vi "ControlProgram6.6_8_updateFFB.vi"() -> ()   [LabVIEW 2016]
uses:
  <vilib>/Utility/miscctls.llb/LVPoint32TypeDef.ctl
  <vilib>/Platform/TimedLoop/XDataNode/timing_clust.ctl
  <vilib>/Platform/TimedLoop/XDataNode/nitl_modes.ctl
  <vilib>/Platform/TimedLoop/XDataNode/wakeup.ctl
  <vilib>/Instr/_visa.llb/Select Event Type.ctl
  <vilib>/vision/Avi1.llb/AviRefnum.ctl
  <vilib>/Utility/error.llb/DialogType.ctl
  <vilib>/DAQmx/write.llb/DAQmx Write (Analog 1D DBL NChan 1Samp).vi
  <vilib>/DAQmx/read.llb/DAQmx Read (Analog 2D DBL NChan NSamp).vi
  <vilib>/Analysis/baseanly.llb/Mean (DBL).vi
  <vilib>/DAQmx/write.llb/DAQmx Write (Digital Bool 1Line 1Point).vi
  <vilib>/DAQmx/create/channels.llb/DAQmx Create Channel (DO-Digital Output).vi
  <vilib>/DAQmx/create/channels.llb/DAQmx Create Channel (AI-Voltage-Basic).vi
  <vilib>/DAQmx/create/channels.llb/DAQmx Create Channel (AO-Voltage-Basic).vi
  <vilib>/DAQmx/configure/timing.llb/DAQmx Timing (Sample Clock).vi
  <vilib>/DAQmx/miscellaneous.llb/DAQmx Fill In Error Info.vi
  <vilib>/Instr/_visa.llb/VISA Configure Serial Port (Instr).vi
  Arnulf--joystick/git(most_up_to_date)/Logitech-joystick/Old Trap/FAST_Global_var.vi
  <vilib>/Utility/inputDevices.llb/mouseAcquire.vi
  <vilib>/Utility/inputDevices.llb/closeMouse.vi
  <vilib>/platform/TimedLoop/XDataNode/XDataNode.xnode
  <vilib>/Platform/TimedLoop/XDataNode/XDNodeRunTimeDep.lvlib
  <resource>/objmgr/daqmx.rc
  <vilib>/Analysis/NI_AALBase.lvlib
panel:
  out "offset ffb param":T1
  in  "Save file index":i32
  out "Saving Move":bool
  out "Move time":string
  out "Primary Video Display":T2(plugin-control)
  out "Flush Sample Start Time":u32=2111292881
  out "Sample flush time (s)":dbl=48.0
  in  "Inject Sample":bool
  out "Cal values":T3={"AX alpha"=612.9626061060078, "BX alpha"=549.6584469744151, "AX kappa"=0.3485731373010688, "BX kappa"=0.3853424216291352, "AX offset"=-0.03900484438240665, "BX offset"=-0.11295550662085417, "AY alpha"=582.7562541114835, "BY alpha"=571.1587543790358, "AY kappa"=0.37498408087930674, "BY kappa"=0.36252029651198364, "AY offset"=-0.21125584642206058, "BY offset"=-0.12469077200400738}
  in  "Inject Pump 1":bool
  in  "Inject Pump 2":bool
  in  "Tab Control 2":T4(tab)
  in  "Force FB script":bool
  in  "Got ADig bead":bool
  in  "Move Cap. 2 (ADig Top)":bool
  in  "Dump beads":bool
  in  "Got DNA bead":bool
  in  "Flow on\ncap 2?":bool=TRUE
  in  "Flow on\ncap 1?":bool=TRUE
  in  "Flow on\ndump?":bool=TRUE
  in  "Raster set":i32=1
  in  "Fish After TA?":bool=TRUE
  in  "Delta after tether":dbl=1700.0
  in  "TA Cancel Save?":bool=TRUE
  in  "Min fish\ndelta (nm)":dbl=1425.0 min=0.0 max=5000.0 step=50.0
  in  "Max fish\ndelta (nm)":dbl=1900.0 min=0.0 max=5000.0 step=25.0
  in  "Fish Speed (ms)":i32=5000
  in  "Wait (ms)":i32=1500
  in  "# attempts":dbl=10.0
  in  "Cutoff force (pN)":dbl=4.5
  in  "Raster after\n tether?":bool=TRUE
  out "Tether":bool
  out "Attempt #":i32
  in  "Flow on\nwhile fish?":bool=TRUE
  in  "Flow on\nafter raster?":bool=TRUE
  in  "Offset raster set":i32
  in  "Offset @ Delta (nm)":dbl=1700.0
  in  "Cal @ Delta (nm)":dbl=2500.0
  in  "Cal stage position":i32=3
  out "Cal Final Sampling Rate":dbl=125000.0
  in  "Cal Averaging":i32=1
  in  "Wait before dip (s)":dbl=3.0
  in  "Start dipping after?":bool
  in  "Start trap delta (nm)":dbl=1700.0
  in  "Repeat Dip":bool
  out "Dip #":i32
  in  "Dip attempts":dbl=3.0
  in  "Cancel Rep\n Dip":bool
  out "Return elasped time":i32
  in  "Return duration":dbl=15.0
  in  "Cancel dwell":bool=TRUE
  in  "Pause dwell":bool
  in  "Start/Return position":dbl=3.0
  in  "Dip duration":dbl=15.0
  in  "Dip position":dbl=4.0
  in  "Dip":bool
  out "Dip elasped time":i32
  in  "Stop":bool=TRUE
  in  "?":T5(tab)
  out "FAST X-Y":bool
  out "FAST Z":bool
  in  "Cal time (s)":dbl=5.0
  in  "Save N sets":bool
  in  "N sets":i32=200
  out "Cal sets to save":i32=500
  in  "Reset data stream":bool
  out "Buffer Overflow":bool
  out "Stage moving":bool
  in  "Comment":string
  in  "Raster scan":bool
  out "Saving":bool
  in  "Save cal":bool
  in  "Save Data":bool
  in  "Stop saving":bool
  out "Calibrating":bool
  out "Progress":dbl(slide) scale=0.0..100.0
  in  "Read Cal":bool
  in  "Fish":bool
  in  "Averaging Number":i32=1250
  out "Final Sampling Rate":dbl=100.0
  in  "Trap position (V)":cluster{"X":dbl, "Y":dbl}={"X"=3.9042624789680316, "Y"=0.2}
  in  "Trap delta (nm)":dbl=2500.0 min=0.0 max=5000.0 step=50.0
  in  "Fixed X":dbl=1.1
  in  "Fixed Y":dbl=0.15
  in  "Shutter 1 (B)":bool
  in  "Shutter 2 (A)":bool
  in  "Pulling direction":bool
  out "Raster scanning...":bool
  out "Current file name":path=path "D:/data/160111/160111_006.dat"
  in  "AX alpha":dbl=612.9626061060078 format="%#_3p"
  in  "BX alpha":dbl=549.6584469744151 format="%#_3g"
  in  "AX kappa":dbl=0.3485731373010688 format="%#_3g"
  in  "BX kappa":dbl=0.3853424216291352 format="%#_3g"
  in  "AX offset":dbl=-0.03900484438240665 format="%#_3g"
  in  "BX offset":dbl=-0.11295550662085417 format="%#_3g"
  in  "AY alpha":dbl=582.7562541114835 format="%#_3g"
  in  "BY alpha":dbl=571.1587543790358 format="%#_3g"
  in  "AY kappa":dbl=0.37498408087930674 format="%#_3g"
  in  "BY kappa":dbl=0.36252029651198364 format="%#_3g"
  in  "AY offset":dbl=-0.21125584642206058 format="%#_3g"
  in  "BY offset":dbl=-0.12469077200400738 format="%#_3g"
  out "Buffer status":u8(slide) scale=0.0..100.0
  in  "Target":bool
  in  "Set Current\nPos to (0,0,0)":bool
  in  "dump spot":string="Dump beads spot"
  in  "up flow spot":string="Upper flow spot"
  in  "low flow spot":string="Lower flow spot"
  in  "up cap":string="Upper capillary (ADig beads)"
  in  "bottom cap":string="Lower capillary (DNA beads)"
  in  "Move to Position 5":bool
  in  "Set Position 5":bool
  in  "Saved stage positions":dbl[][](array[numeric])=[[1.0, 0.0, 0.0, 0.0], [2.0, -0.13716, -3.21132, 0.01436], [3.0, 0.45, -0.73974, 0.005], [4.0, 0.45, -2.1978, 0.005], [5.0, 0.45, -2.63158, -0.02256]]
  in  "Set Position 2":bool
  in  "Move to Position 2":bool
  in  "Set Position 1":bool
  in  "Move to Position 1":bool
  in  "Set Position 4":bool
  in  "Move to Position 4":bool
  in  "Set Position 3":bool
  in  "Move to Position 3":bool
  out "Stage error":errorcluster
  in  "Clear Volume":bool
  out "Sample Flush Meter":u8(slide) scale=0.0..100.0
  out "Flushing Sample":bool
  in  "Flush Sample":bool
  in  "Normal \nRate (ul/hr)  3":dbl=100.0
  in  "Normal \nVolume (ul) 3":dbl=250.0
  in  "Normal \nVolume (ul) 2":dbl
  in  "Normal \nRate (ul/hr)":dbl
  in  "Normal \nVolume (ul)":dbl
  in  "Flush\nRate (ul/min)":dbl
  in  "Flush\nVolume (ul)":dbl
  in  "Flush \nRate (ul/min)  2":dbl
  in  "Flush Pump 2":bool
  in  "Flush\nVolume (ul)  2":dbl
  in  "Flush Pump 1":bool
  in  "Normal \nRate (ul/hr)  2":dbl
  in  "Write Wait":i32=1000
  in  "Flush \nRate (ul/min)  3":dbl=100.0
  in  "Flush\nVolume (ul)  3":dbl=80.0
  out "error out":errorcluster
  in  "Use Mouse to Move Trap?":bool
  in  "Pause Mouse/Mirror Connection":bool
  out "Reference Voltage":cluster{dbl, dbl}={0.0, -0.0}
  out "Saved voltage":cluster{dbl, dbl}={5.766666666666665, 1.45}
  out "Real Coordinates":cluster{"Horizontal":i32, "Vertical":i32}={"Horizontal"=897, "Vertical"=-1271}
  out "CoordinatesMousePressed":T6
  in  "reset offset ffb param":bool
  in  "Read \nOffset FFB param":bool
  in  "Force Feedback 2":bool
  in  "Offset 2":cluster{"Off Y":dbl, "Off X":dbl}={"Off Y"=1.5, "Off X"=0.17}
  in  "Setpoint voltage 2":cluster{"SP Y":dbl, "SP X":dbl}={"SP Y"=0.6, "SP X"=0.0}
  out "Sum error":dbl(knob) scale=-0.2..0.2
  out "Trap sep":waveform(dbl)[](graph)=[{"t0"=timestamp(4.489999999999949 s since 1904-01-01), "dt"=0.002, "Y"=[-1157.7639781743756, -1157.678951177374, -1157.7582331070425, -1157.7490409992681, -1157.8995617642552], "attributes"=variant("NI_ChannelName"=variant(string "T2 X"))}, {"t0"=timestamp(4.489999999999949 s since 1904-01-01), "dt"=0.002, "Y"=[-909.0775466981794, -909.1316439023619, -909.1322956759037, -909.1570630705896, -909.1264297140281], "attributes"=variant("NI_ChannelName"=variant(string "T2 Y"))}]
  in  "Set reading to\nsetpoint 1":bool
  in  "Offset Y (nm)":dbl format="%0.2f"
  in  "Offset X (nm)":dbl format="%0.2f"
  in  "Remove offsets":bool
  in  "Force Feedback 1":bool
  out "Feedback Output \nVoltage 2":cluster{dbl, dbl} {"?" format="%#_4g"; "?" format="%#_4g"}
  in  "Offset 1":cluster{"Off Y":dbl, "Off X":dbl}={"Off Y"=1.5, "Off X"=0.17}
  in  "Setpoint voltage 1":cluster{"SP Y":dbl, "SP X":dbl}={"SP Y"=0.6, "SP X"=0.0}
  in  "Feedback const":T7={"Ki_B_Y"=0.5, "Ki_B_X"=0.0, "Kp Y"=1.0, "Kp X"=0.0}
  out "Mean Trap Pos X 2 (nm)":dbl=-1157.769953044463 format="%0.2f"
  out "Mean Trp Pos Y 2 (nm)":dbl=-909.1249958122125 format="%0.2f"
  out "T2 X RMS (A)":dbl=0.7168002469275427 format="%0.2f"
  out "T2 Y RMS (A)":dbl=0.25997187037503383 format="%0.2f"
  in  "Set reading to\nsetpoint 2":bool
  in  "Scan range (nm)":dbl=425.0
  in  "Scan speed (nm/s)":dbl=100.0 min=0.0 max=100.0
  in  "Step size (nm)":dbl=1.0
  in  "Save scans":bool=TRUE
  in  "# scans":i32=1
  in  "Load param":bool
  in  "Scan Parameters":T8(array[cluster])
  in  "Trap delta\nafter (nm)":dbl=1550.0
  in  "Stop raster":bool
  out "Scan range (V)":dbl=0.47672462142456534
  out "Scan steps (mirror)":u64=425
  out "Scan increment (V)":dbl=0.0011217049915872126
  out "Time per step (ms)":dbl=10.0
  out "Total raster time (s)":dbl=8.5
  out "N sets to be saved":dbl=850.0
  out "moveX":string
  out "moveY":string
  in  "Grid Movable Trap":bool
  in  "take fixed bead\n Images":bool
  in  "Zoom Factor":sgl=7.0
  in  "Center Point":cluster{"X":i32, "Y":i32}={"X"=335, "Y"=271}
  in  "Intensity Upper":dbl=88.0
  in  "Intensity Lower":dbl=66.0
  out "Window Size":cluster{"Height":i32, "Width":i32}
  in  "Image Index":dbl=1.0 min=1.0
  in  "Save Image":bool
  in  "Averaging":bool
  in  "Reset Averaging":bool
  in  "Save Video":bool
  in  "New Video File":bool
  in  "Video Index":dbl=1.0 min=1.0 step=1.0
  in  "Video Capture Rate (Hz)":dbl=30.0
  in  "Initial Window Size":cluster{"Width":i32, "Height":i32}={"Width"=884, "Height"=619}
  in  "Initial Window Position":cluster{"X Position":i32, "Y Position":i32}={"X Position"=796, "Y Position"=4}
  out "Window Position":cluster{"X Position":i32, "Y Position":i32}={"X Position"=40, "Y Position"=40}
  out "Path Out":path
  in  "Target coordinates":cluster{"X1":dbl, "Y1":dbl, "X2":dbl, "Y2":dbl}={"X1"=328.0, "Y1"=274.0, "X2"=368.0, "Y2"=314.0}
  out "image8bitArray":u8[][](array[numeric])
  out "GreyscaleArray":u32[](array[numeric])
  in  "take background images":bool
  in  "# Samples/channel (in)":i32=40000 format="%.2f"
  out "Buffer size\n(Samples/channel)":u32=511
  out "DAQ rate\n(Samples/s)":dbl=125000.0 format="%#_6p"
  out "# Samples/channel":i32=1250
  out "# Samples/channel/s":dbl=100.0
  out "AvailSampPerChan":u32=9
  out "Data update period (s/set)":dbl=0.01 format="%#_6p"
  out "AvailSampPerChan 2":u32=110
  in  "PC samp per channel":i32=1000
  in  "Sampling Rate":dbl=125000.0 format="%0.0p"
  in  "DAQ Rate2":dbl=1000000.0 format="%#_6p"
  out "Data period (s)":dbl=8e-06 format="%#_6p"
  in  "Save user params":bool
  in  "User":string(combo)
  in  "Load user params":bool
  in  "Tether break\nforce (pN)":dbl=1.0
  in  "Path":path=path "E:/Data"
  out "Mirror task":refnum<k21>
  in  "Conv X (nm/V)":dbl=891.5
  in  "Conv Y (nm/V)":dbl=505.7
  in  "Min value Y":dbl format="%.1g"
  in  "Max value Y":dbl=10.0 format="%.1f"
  in  "Min value X":dbl format="%0.1f"
  in  "Max value X":dbl=10.0 format="%.1f"
  in  "HWP1":string="Half waveplate 1: differential trap power"
  in  "HWP0":string="Half waveplate 0: total trap power"
  in  "Move 1":bool
  in  "\"Degrees\" 1":dbl
  in  "Move 0":bool
  in  "\"Degrees\" 0":dbl
  in  "Y command":enum16{"Fish", "Dump", "Got ADig", "Got DNA"}(ring)
  in  "B command":enum16{"Got DNA", "Got ADig", "Dump", "Fish"}(ring)
  in  "A command":enum16{"Got ADig", "Dump", "Fish", "Got DNA"}(ring)
  in  "X command":enum16{"Dump", "Fish", "Got ADig", "Got DNA"}(ring)
  out "Logitech":bool
  out "START":bool
  out "BACK":bool
  out "Right stick button":bool
  out "Left Y":i8(slide) scale=-128.0..127.0
  out "Left X":i8(slide) scale=-128.0..127.0
  out "Right Y":i8(slide) scale=-128.0..127.0
  out "Right X":i8(slide) scale=-128.0..127.0
  out "X":bool
  out "Y":bool
  out "A":bool
  out "B":bool
  out "RB":bool
  out "LB":bool
  out "R":bool
  out "L":bool
  out "D":bool
  out "U":bool
  out "Left stick button":bool
  out "FAST Z":bool
  out "FAST X-Y":bool
  in  "XY Speed Definitions":T9={"Slow X velocity input"="0.05", "Slow Y velocity input"="0.05", "Fast1 X velocity input"="0.1", "Fast1 Y velocity input"="0.1", "Fast2 X velocity input"="0.2", "Fast2 Y velocity input"="0.2"}
  in  "Z Speed Definitions":cluster{"Slow Z":string, "Fast Z":string}={"Slow Z"="0.025", "Fast Z"="0.05"}
  in  "Z Wait time":string="120"
  in  "X-Y Wait time":string="125"
  in  "USB port":refnum<visa-resource-name>="USB0::0x046D::0xC21D::CC66247B::RAW"
  out "Deflection":T6
  in  "Sampling Rate":dbl=125000.0 format="%0.2f"
  in  "Averaging Number":i32=12500
  in  "DAQ Rate":dbl=1000000.0
  out "Final Sampling Rate":dbl
  in  "Tab Control":T10(tab)
  in  "Downsamp\nfact":dbl=250.0
  out "Bead sep":waveform(dbl)[](graph)=[{"t0"=timestamp(4.489999999999949 s since 1904-01-01), "dt"=0.002, "Y"=[8093.963535945606, 8103.1617772716045, 8385.72390184118, 8245.733099167523, 8154.925676756515], "attributes"=variant("NI_ChannelName"=variant(string "T2"))}, {"t0"=timestamp(4.489999999999949 s since 1904-01-01), "dt"=0.002, "Y"=[1717.924930434114, 1628.723007842151, 1787.6888378897193, 1598.475730715916, 1776.2517588078954], "attributes"=variant("NI_ChannelName"=variant(string "T1"))}]
  out "Force (pN)":waveform(dbl)[](graph)=[{"t0"=timestamp(4.489999999999949 s since 1904-01-01), "dt"=0.002, "Y"=[2821.5994183803123, 2824.8226375853515, 2923.3663028678166, 2874.5254578927593, 2842.869034836209], "attributes"=variant("NI_ChannelName"=variant(string "T2"))}, {"t0"=timestamp(4.489999999999949 s since 1904-01-01), "dt"=0.002, "Y"=[623.5850847499229, 591.0680427774053, 648.761979867749, 579.944408346982, 644.7436619059413], "attributes"=variant("NI_ChannelName"=variant(string "T1"))}]
  out "Mean force (pN)":dbl=1737.5286029210451 format="%0.2f"
  out "Force noise (pN)":dbl=26.83032703631318 format="%0.2f"
  out "Mean Bead Sep\n(nm)":dbl=4949.257225667222 format="%0.2f"
  out "Bead Sep Noise\n(A)":dbl=757.8078481959694 format="%0.2f"
  out "PSD 2":cluster{dbl[], dbl[]}(graph)
  out "PSD 1":cluster{dbl[], dbl[]}(graph)
  out "PSD 1 Sum":dbl(slide) scale=0.0..10.0
  out "PSD 2 Sum":dbl(slide) scale=0.0..10.0
  in  "Start":bool
  out "All signals 2":waveform(dbl)[](graph)=[{"t0"=timestamp(4.489999999999949 s since 1904-01-01), "dt"=0.002, "Y"=[0.0010396217068286443, 0.0010666908927528754, 0.001103298744846499, 0.0010651440823993424, 0.0010656596859401936], "attributes"=variant("NI_ChannelName"=variant(string "A y"))}, {"t0"=timestamp(4.489999999999949 s since 1904-01-01), "dt"=0.002, "Y"=[0.02000680227246931, 0.020097032918054827, 0.02003412926844257, 0.020136734401221615, 0.020087494249822452], "attributes"=variant("NI_ChannelName"=variant(string "A x"))}, {"t0"=timestamp(4.489999999999949 s since 1904-01-01), "dt"=0.002, "Y"=[-0.0014958587831537804, -0.0015046240440107857, -0.0014930229638311983, -0.001533240041751485, -0.0015262793936602433], "attributes"=variant("NI_ChannelName"=variant(string "B y"))}, {"t0"=timestamp(4.489999999999949 s since 1904-01-01), "dt"=0.002, "Y"=[0.0002901198559372817, 0.0002731049385577592, 0.00026511308349727467, 0.0002517073909711183, 0.0002916666665966012], "attributes"=variant("NI_ChannelName"=variant(string "B x"))}, {"t0"=timestamp(4.489999999999949 s since 1904-01-01), "dt"=0.002, "Y"=[-0.001511556786147372, -0.0015167122027053212, -0.0014612914746018214, -0.0014935128282145193, -0.0015064013696263116], "attributes"=variant("NI_ChannelName"=variant(string "A sum"))}, {"t0"=timestamp(4.489999999999949 s since 1904-01-01), "dt"=0.002, "Y"=[-0.0005242945138364382, -0.0005565158674093218, -0.000501095139248956, -0.0005771375336978897, -0.0005165613890095197], "attributes"=variant("NI_ChannelName"=variant(string "B sum"))}, {"t0"=timestamp(4.489999999999949 s since 1904-01-01), "dt"=0.002, "Y"=[0.0013303666019343777, 0.0014257418088905328, 0.0013368108726387405, 0.0013471217058124534, 0.0011782818123890176], "attributes"=variant("NI_ChannelName"=variant(string "Trap x"))}, {"t0"=timestamp(4.489999999999949 s since 1904-01-01), "dt"=0.002, "Y"=[0.0023382505474007294, 0.002231275652833831, 0.002229986798687363, 0.0021810103409340116, 0.002241586486003531], "attributes"=variant("NI_ChannelName"=variant(string "Trap y"))}]
  out "All signals":waveform(dbl)[](graph)=[{"t0"=timestamp(4.489999999999949 s since 1904-01-01), "dt"=0.002, "Y"=[0.0010396217068286443, 0.0010666908927528754, 0.001103298744846499, 0.0010651440823993424, 0.0010656596859401936], "attributes"=variant("NI_ChannelName"=variant(string "A y"))}, {"t0"=timestamp(4.489999999999949 s since 1904-01-01), "dt"=0.002, "Y"=[0.02000680227246931, 0.020097032918054827, 0.02003412926844257, 0.020136734401221615, 0.020087494249822452], "attributes"=variant("NI_ChannelName"=variant(string "A x"))}, {"t0"=timestamp(4.489999999999949 s since 1904-01-01), "dt"=0.002, "Y"=[-0.0014958587831537804, -0.0015046240440107857, -0.0014930229638311983, -0.001533240041751485, -0.0015262793936602433], "attributes"=variant("NI_ChannelName"=variant(string "B y"))}, {"t0"=timestamp(4.489999999999949 s since 1904-01-01), "dt"=0.002, "Y"=[0.0002901198559372817, 0.0002731049385577592, 0.00026511308349727467, 0.0002517073909711183, 0.0002916666665966012], "attributes"=variant("NI_ChannelName"=variant(string "B x"))}, {"t0"=timestamp(4.489999999999949 s since 1904-01-01), "dt"=0.002, "Y"=[-0.001511556786147372, -0.0015167122027053212, -0.0014612914746018214, -0.0014935128282145193, -0.0015064013696263116], "attributes"=variant("NI_ChannelName"=variant(string "A sum"))}, {"t0"=timestamp(4.489999999999949 s since 1904-01-01), "dt"=0.002, "Y"=[-0.0005242945138364382, -0.0005565158674093218, -0.000501095139248956, -0.0005771375336978897, -0.0005165613890095197], "attributes"=variant("NI_ChannelName"=variant(string "B sum"))}, {"t0"=timestamp(4.489999999999949 s since 1904-01-01), "dt"=0.002, "Y"=[0.0013303666019343777, 0.0014257418088905328, 0.0013368108726387405, 0.0013471217058124534, 0.0011782818123890176], "attributes"=variant("NI_ChannelName"=variant(string "Trap x"))}, {"t0"=timestamp(4.489999999999949 s since 1904-01-01), "dt"=0.002, "Y"=[0.0023382505474007294, 0.002231275652833831, 0.002229986798687363, 0.0021810103409340116, 0.002241586486003531], "attributes"=variant("NI_ChannelName"=variant(string "Trap y"))}]
  out "Chart Freq (Hz)":dbl=500.0
  # "Bead Calibration"
  # "Y"
  # "X"
  # "Pump #1 Controls"
  # "Pump #2 Controls"
  # "Sample Pump Controls"
  # "Retract the pumps manually. Change it back to INFUSE when you're done. Suck it up, don't whine."
  # "Shutter 1 (B)"
  # "Move to Lower Cap"
  # "Inject Sample"
  # "Move to Upper Cap"
  # "Shutter 2 (A)"
  # "Select the Joystick input:"
  # "Overflow happens when >40 commands\nsent in 5 seconds. Then 4 consecutive beeps."
  # "Try increasing wait time to reduce 'following error threshold exceeded' occurances."
  # "Left stick controls Z axis.\nRight on stick: neg Z-dir\nUp on stick: neg Z-dir"
  # "Toggles FAST Z"
  # "Toggles FAST X-Y"
  # "The default Newport max velocity is 0.4"
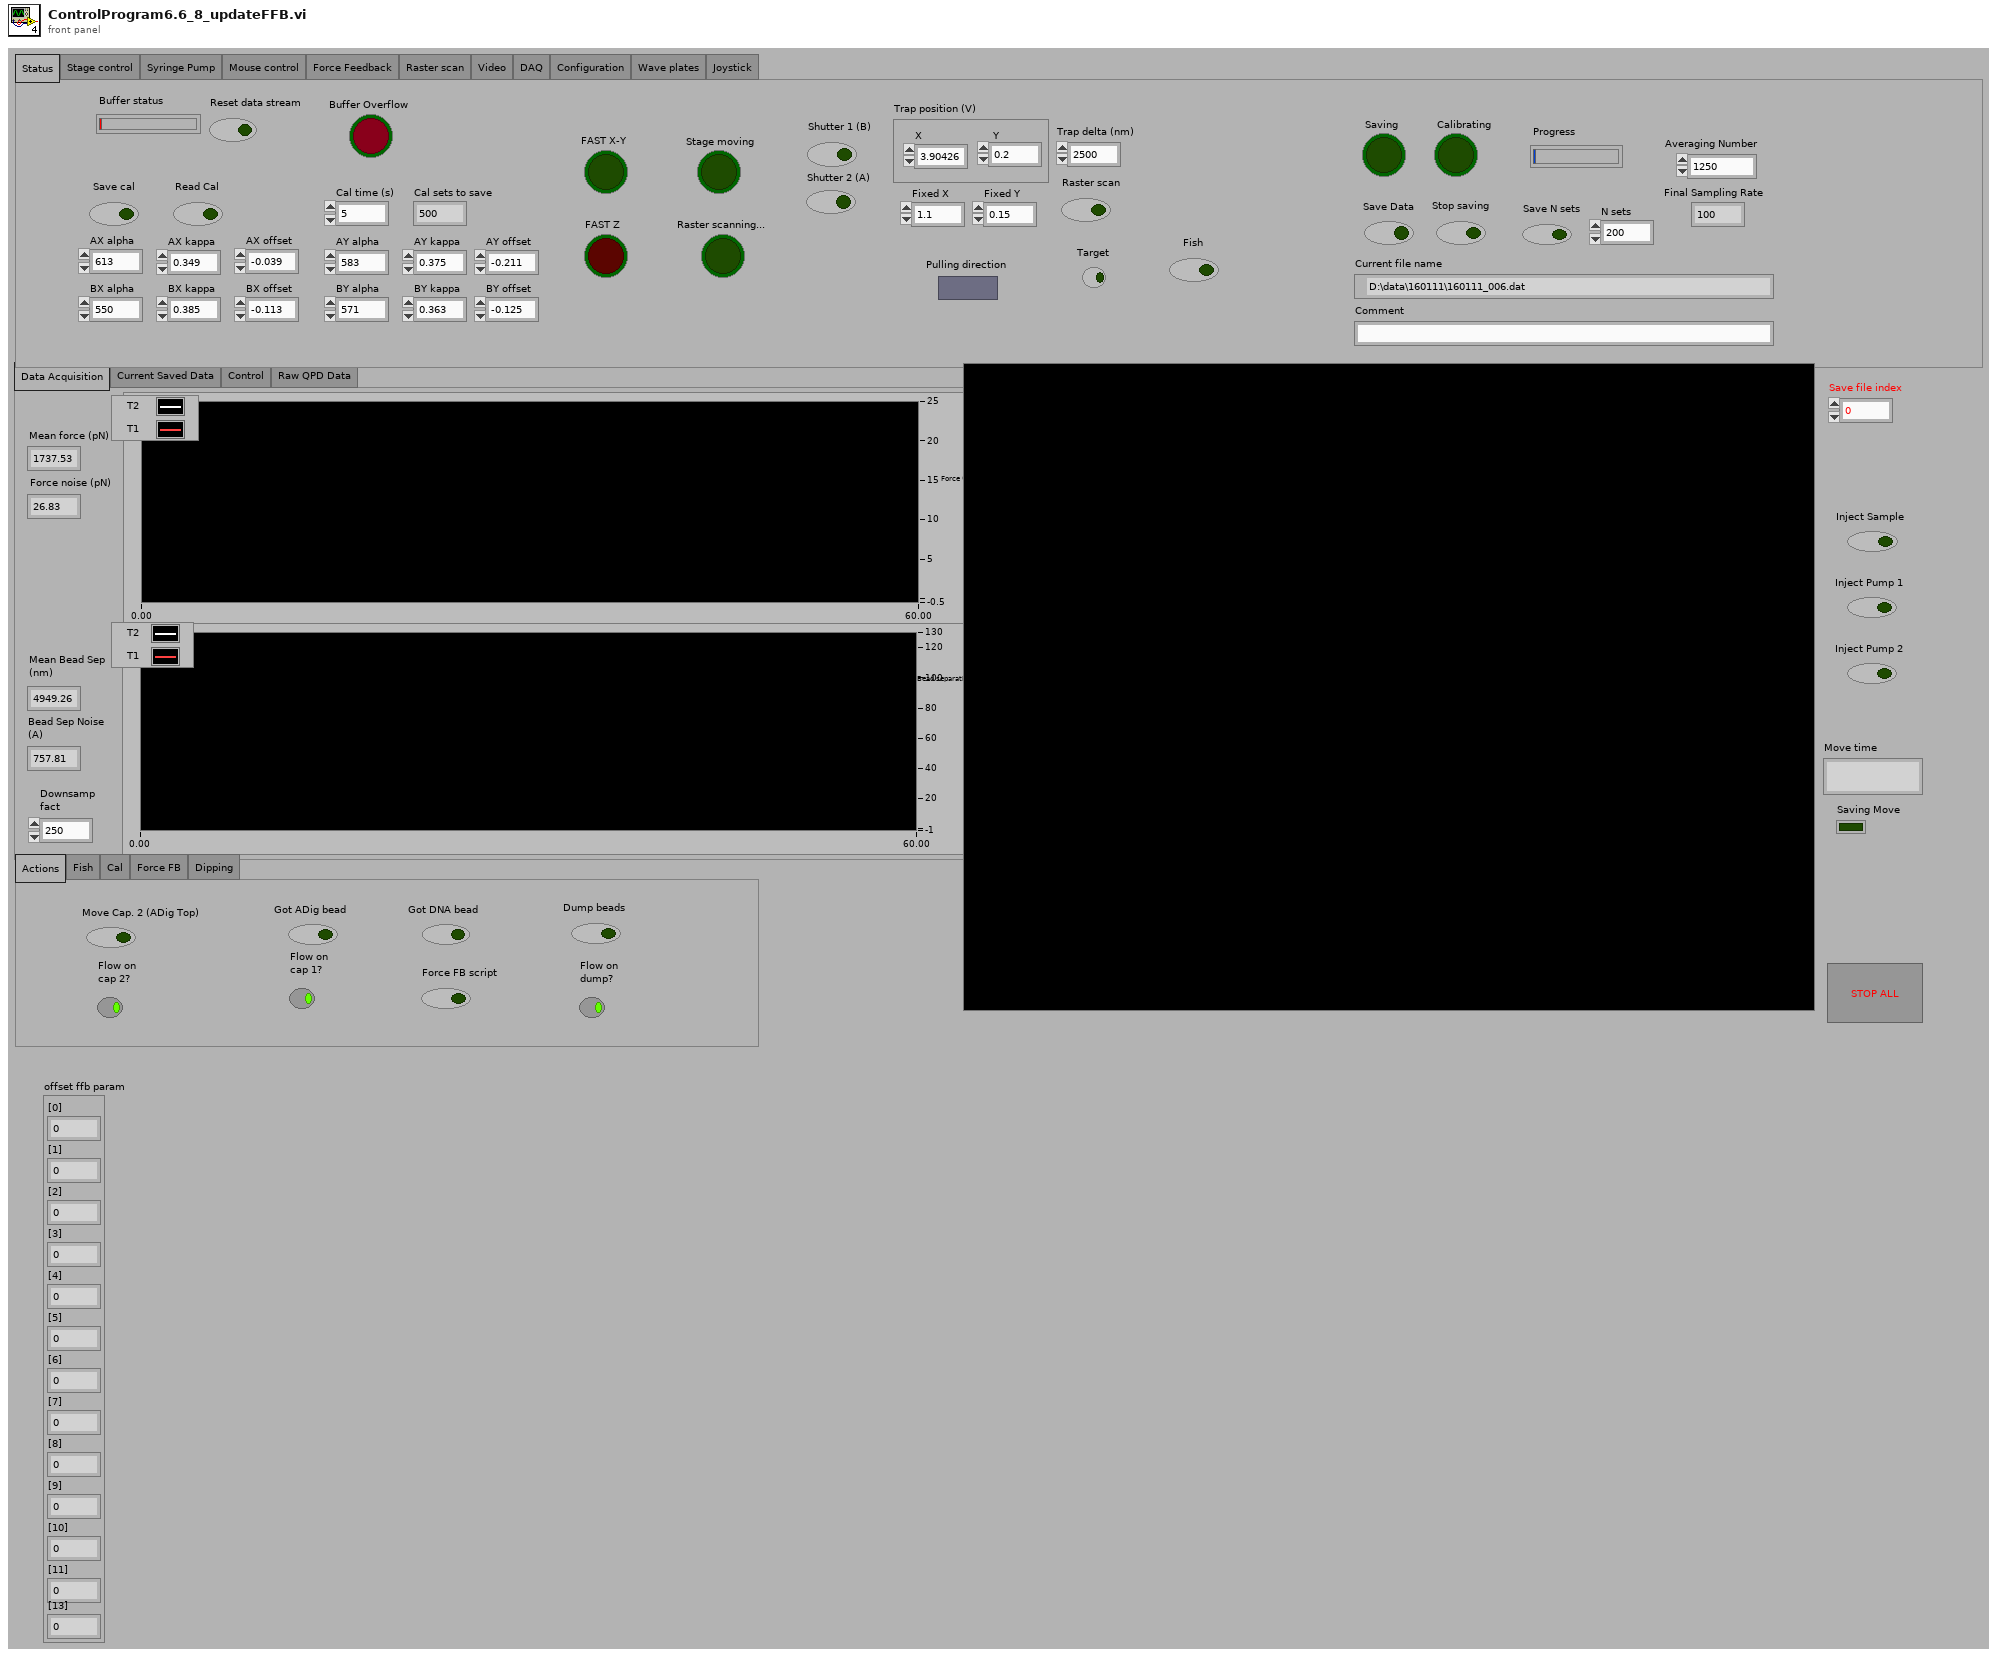
[diagram p1: front panel]
types:
  T1 = cluster{"[0]":dbl, "[1]":dbl, "[2]":dbl, "[3]":dbl, "[4]":dbl, "[5]":dbl, "[6]":dbl, "[7]":dbl, "[8]":dbl, "[9]":dbl, "[10]":dbl, "[11]":dbl, "[13]":dbl}
  T2 = typedef "IMAQ Image.ctl" = refnum<image>
  T3 = cluster{"AX alpha":dbl, "BX alpha":dbl, "AX kappa":dbl, "BX kappa":dbl, "AX offset":dbl, "BX offset":dbl, "AY alpha":dbl, "BY alpha":dbl, "AY kappa":dbl, "BY kappa":dbl, "AY offset":dbl, "BY offset":dbl}
  T4 = enum32{"Actions", "Fish", "Cal", "Force FB", "Dipping"}
  T5 = enum32{"Status", "Stage control", "Syringe Pump", "Mouse control", "Force Feedback", "Raster scan", "Video", "DAQ", "Configuration", "Wave plates", "Joystick"}
  T6 = typedef "LVPoint32TypeDef.ctl" = cluster{"Horizontal":i32, "Vertical":i32}
  T7 = cluster{"Ki_B_Y":dbl, "Ki_B_X":dbl, "Kp Y":dbl, "Kp X":dbl}
  T8 = cluster{"Label":string, "Scan range 1":dbl, "Step size 1":dbl, "Scan speed 1":i32, "# scans 2":i32}[]
  T9 = cluster{"Slow X velocity input":string, "Slow Y velocity input":string, "Fast1 X velocity input":string, "Fast1 Y velocity input":string, "Fast2 X velocity input":string, "Fast2 Y velocity input":string}
  T10 = enum32{"Data Acquisition", "Current Saved Data", "Control", "Raw QPD Data"}
  T11 = typedef "Select Event Type.ctl" = u32
  T12 = enum32{"setting", "request", "request control", "info", "statistics", "system settings", "I/O sub system", "HRT control", "camera descriptions", "device specific data", "event sub system settings", "event sub system results", "image memory manager"}
  T13 = typedef "AviRefnum.ctl" = refnum<k1>
  T14 = typedef "XDNodeRunTimeDep.lvlib/timing_clust.ctl" = cluster{"Expected End [f-1]":u64, "Actual End [f-1]":u64, "Finished Late? [f-1]":bool, "Expected End [i-1]":u64, "Actual End [i-1]":u64, "Finished Late? [i-1]":bool, "Expected Start [i]":u64, "Actual Start [i]":u64, "Expected Start [f]":u64, "Actual Start [f]":u64, "Source Name":string, "Structure Name":string, "Period":i64, "Deadline":i64, "Offset":i64, "Start":i64, "Priority":i32, "Timeout":i32, "Mode":T15, "Wakeup Reason":T16, "Error":errorcluster, "Source Type":string, "Secondary Source Type":string, "Global End Time":u64, "Global Start Time":u64, "Frame Duration":u64, "Iteration Duration":u64, "Assigned CPU":i32, "I/O Scan Engine Mode":u32}
  T15 = typedef "XDNodeRunTimeDep.lvlib/nitl_modes.ctl" = enum32{"No Change", "Process missed periods, maintain original phase", "Discard missed periods, maintain original phase", "Process missed periods, ignore original phase", "Discard missed periods, ignore original phase"}
  T16 = typedef "XDNodeRunTimeDep.lvlib/wakeup.ctl" = enum32{"Normal", "Aborted", "Asynchronous wakeup", "Timing source error", "Timed loop error", "Timeout"}
  T17 = typedef "Image Type" = u32
  T18 = typedef "imagedata.ctl" = cluster{"image type":i32, "image depth":i32, "image":u8[], "mask":u8[], "colors":u32[], "Rectangle":cluster{"left":i16, "top":i16, "right":i16, "bottom":i16}}
  T19 = enum16{"open", "replace", "create", "open or create", "replace or create", "replace or create with confirmation"}
  T20 = enum16{"big-endian, network order", "native, host order", "little-endian"}
  T21 = cluster{string, string, string, string, string, string, string, string}
  T22 = cluster{"LB":bool, "RB":bool, "BACK":bool, "Logitech":bool, "START":bool}
  T23 = cluster{"Right X":i8, "Right Y":i8, "Left X":i8, "Left Y":i8}
  T24 = enum32{"Status", "Stage control", "Syringe Pump", "Mouse control", "Force Feedback", "Raster scan", "Video", "DAQ", "Configuration", "Wave plates"}
  T25 = typedef "DialogType.ctl" = u16
  T26 = cluster{"button 1":bool, "button 2":bool, "button 3":bool, "button 4":bool}
  T27 = cluster{"[0]":dbl, "[1]":dbl, "[2]":dbl, "[3]":dbl, "[4]":dbl, "[5]":dbl, "[6]":dbl, "[7]":dbl, "[8]":dbl, "[9]":dbl, "[10]":dbl, "[11]":dbl}
  T28 = cluster{"[0]":dbl, "[1]":dbl, "[2]":dbl, "[3]":dbl, "[4]":dbl, "[5]":dbl, "[6]":dbl, "[7]":dbl, "[8]":dbl, "[9]":dbl, "[10]":dbl, "[11]":dbl, "[12]":dbl}
  T29 = cluster{"array[0]":dbl, "array[1]":dbl, "array[2]":dbl, "array[3]":dbl, "array[4]":dbl, "array[5]":dbl, "array[6]":dbl, "array[7]":dbl, "array[8]":dbl, "array[9]":dbl, "array[10]":dbl, "array[11]":dbl, "array[12]":dbl}
  T30 = cluster{"Label":string, "Scan range 1":dbl, "Step size 1":dbl, "Scan speed 1":i32, "# scans 2":i32}
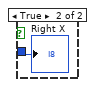
[diagram p5: hidden frame]
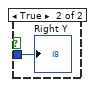
[diagram p6: hidden frame]
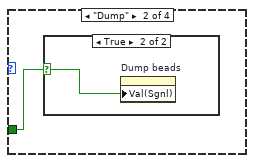
[diagram p10: hidden frame]
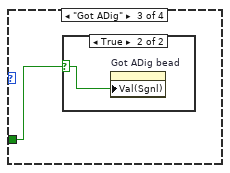
[diagram p12: hidden frame]
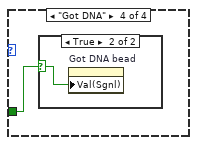
[diagram p14: hidden frame]
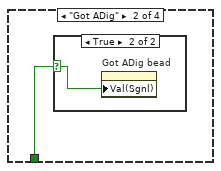
[diagram p17: hidden frame]
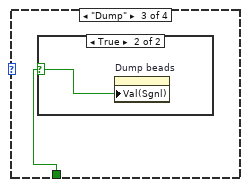
[diagram p19: hidden frame]
diagram:
  w10 = T11 1073684535 items=["Service Request"=1073684491, "Trigger"=3221168138, "Clear"=1073684493, "VXI Signal"=1073684512, "VXI/VME Interrupt"=3221168161, "VXI/VME Sysfail"=1073684509, "VXI/VME Sysreset"=1073684510, "GPIB CIC"=1073684498, "GPIB Talk"=1073684499, "GPIB Listen"=1073684500, "PXI Interrupt"=1073684514, "Serial Break"=1073684515, "Serial TermChar"=1073684516, "Serial CTS"=1073684521, "Serial DSR"=1073684522, "Serial DCD"=1073684524, "Serial RI"=1073684526, "Serial Character"=1073684533, "USB Interrupt"=1073684535, "All Enabled"=1073709055] ("Event Type")
  w49 = 10.0 ("Minimum Value")
  w50 = -10.0 ("Minimum Value")
  w52 = -2.0 ("Minimum Value")
  w53 = 2.0 ("Maximum Value")
  w78 = 10123 items=["Finite Samples"=10178, "Continuous Samples"=10123] ("sample mode")
  w98 = tag "Dev1/port2/line1"  # Shutter 2
  w101 = tag "Dev1/port1/line4"  # Shutter 1
  # "Open the RAW resource"
  # "Enable USB Interrupt Event"
  # "Create channels for movable mirror"
  # "Create channels for detectors"
  n1 = call-poly <vilib>:"DAQmx Create Virtual Channel.vi"("maximum value"=w53, "minimum value"=w52, "physical channels"=tag "Dev1/ai0" ("Physical Channel")) -> ("task out"=w54:refnum<k21>, "error out"=w77:errorcluster)  [unwired: 11 in]
  n2 = call-poly <vilib>:"DAQmx Create Virtual Channel.vi"("task in"=w54, "maximum value"=w53, "minimum value"=w52, "physical channels"=tag "Dev1/ai1", "error in"=w77) -> ("task out"=w75:refnum<k21>, "error out"=w74:errorcluster)  [unwired: 9 in]
  n3 = call-poly <vilib>:"DAQmx Create Virtual Channel.vi"("task in"=w75, "maximum value"=w53, "minimum value"=w52, "physical channels"=tag "Dev1/ai2", "error in"=w74) -> ("task out"=w66:refnum<k21>, "error out"=w65:errorcluster)  [unwired: 9 in]
  n4 = call-poly <vilib>:"DAQmx Create Virtual Channel.vi"("task in"=w66, "maximum value"=w53, "minimum value"=w52, "physical channels"=tag "Dev1/ai3" ("Physical Channel"), "error in"=w65) -> ("task out"=w51:refnum<k21>, "error out"=w71:errorcluster)  [unwired: 9 in]
  n5 = call-poly <vilib>:"DAQmx Create Virtual Channel.vi"("task in"=w51, "maximum value"=w49, "minimum value"=w50, "physical channels"=tag "Dev1/ai4", "error in"=w71) -> ("task out"=w69:refnum<k21>, "error out"=w68:errorcluster)  [unwired: 9 in]
  n6 = call-poly <vilib>:"DAQmx Create Virtual Channel.vi"("task in"=w69, "maximum value"=w49, "minimum value"=w50, "physical channels"=tag "Dev1/ai5", "error in"=w68) -> ("task out"=w64:refnum<k21>, "error out"=w63:errorcluster)  [unwired: 9 in]
  n7 = call-poly <vilib>:"DAQmx Create Virtual Channel.vi"("task in"=w64, "maximum value"=w49, "minimum value"=w50, "physical channels"=tag "Dev1/ai6", "error in"=w63) -> ("task out"=w58:refnum<k21>, "error out"=w56:errorcluster)  [unwired: 9 in]
  n8 = call-poly <vilib>:"DAQmx Create Virtual Channel.vi"("task in"=w58, "maximum value"=w49, "minimum value"=w50, "physical channels"=tag "Dev1/ai7", "error in"=w56) -> ("task out"=w57:refnum<k21>, "error out"=w55:errorcluster)  [unwired: 9 in]
  n9 = call-poly <vilib>:"DAQmx Timing.vi"("task/channels in"=w57, "sample mode"=w78, "samples per channel"="PC samp per channel", "rate"="Sampling Rate", "error in"=w55) -> ("task out"=w61:refnum<k21>, "error out"=w60:errorcluster)  [unwired: 9 in]
  n10 = call-poly <vilib>:"DAQmx Create Virtual Channel.vi"("maximum value"="Max value Y", "minimum value"="Min value Y", "physical channels"=tag "Dev1/ao1" ("Trap X Axis")) -> ("task out"=w46:refnum<k21>, "error out"=w48:errorcluster)  [unwired: 11 in]
  n11 = property class="DAQmx Timing"(reference=w61, error in=w60, "More:AI Convert:Rate"="DAQ Rate2") -> (reference out=w19:refnum<k21>, error out=w18:errorcluster, "SampClk.Rate"=→"DAQ rate\n(Samples/s)":dbl)
  n12 = call-poly <vilib>:"DAQmx Create Virtual Channel.vi"("task in"=w46, "maximum value"="Max value X", "minimum value"="Min value X", "physical channels"=tag "Dev1/ao0" ("Trap Y Axis"), "error in"=w48) -> ("task out"=w37:refnum<k21>, "error out"=w36:errorcluster)  [unwired: 9 in]
  "Mirror task" <- w37
  n13 = property class="DAQmx Buffer"(reference=w19, error in=w18) -> (reference out=w16:refnum<k21>, error out=w15:errorcluster, "Input.OnbrdBufSize"=→"Buffer size\n(Samples/channel)":u32)
  n14 = call <vilib>:"DAQmx Start Task.vi"("task/channels in"=w16, "error in"=w15) -> ("task out"=w38:refnum<k21>)  [unwired: 12 in, 1 out]
  n15 = flat-sequence "Video" {
    tunnel: [w114] -> w13
    tunnel: w13 -> [w155]
    frame #0 {
      n16 = while {
        stop <- w107 continue-if-true
        n17 = call "Close Video Capture.vi"() -> ("error code OUT"=w109:i32)
        n18 = Equal?(x=w109, y=0) -> (x = y?=w107:bool)
      }
      n19 = local write "Stop"(FALSE ("Stop All")) -> ()
    }
    frame #1 {
      n20 = call "DMR_Init.vi"() -> ()  [unwired: 3 out]
    }
    frame #2 {
      # "Setting the destination format to Mono8 makes sure that the image can be displayed in the intensity plot."
      n21 = call "DMR_GetDevice.vi"("search string IN"="DE514724602") -> ("device handle OUT"=w132:i32)  [unwired: 4 in, 2 out]
      n22 = call "DMR_OpenDevice.vi"("device handle IN"=w132) -> ("driver handle OUT"=w115:i32)  [unwired: 4 out]
      n23 = call "DMR_FindList.vi"("flags IN"=u32 0 ("flags"), "list name IN"="" ("String"), "list type IN"=T12."camera descriptions", "driver handle IN"=w115) -> ("list handle OUT"=w118:i32)  [unwired: 2 out]
      n24 = call "DMR_FindList.vi"("flags IN"=u32 0 ("flags"), "list name IN"="Base", "list type IN"=T12."setting", "driver handle IN"=w115) -> ("list handle OUT"=w116:i32)  [unwired: 2 out]
      n25 = call "OBJ_GetHandle.vi"("object name IN"="VideoStandard", "list handle IN"=w118) -> ("object handle OUT"=w112:i32)  [unwired: 3 out]
      n26 = call "OBJ_GetHandle.vi"("object name IN"="PixelFormat", "list handle IN"=w116) -> ("object handle OUT"=w126:i32)  [unwired: 3 out]
      n27 = call "OBJ_SetS.vi"("value index IN"=0, "value IN"="NTSC M", "object handle IN"=w112) -> ()  [unwired: 2 out]
      n28 = call "OBJ_SetS.vi"("value index IN"=0, "value IN"="Mono8" ("value"), "object handle IN"=w126) -> ()  [unwired: 2 out]
      n29 = call "OBJ_GetHandle.vi"("object name IN"="VideoChannel", "list handle IN"=w116) -> ("object handle OUT"=w122:i32)  [unwired: 3 out]
      n30 = while {
        tunnel: [w137] -> w114
        tunnel: w115 -> [w134]
        stop <- w135 continue-if-true
        n31 = call "DMR_ImageRequestSingle.vi"("request control IN"=0, "driver handle IN"=w134) -> ("error code OUT"=w136:i32, "driver handle OUT"=w137:i32)  [unwired: 2 out]
        n32 = Equal To 0?(x=w136) -> (x = 0?=w135:bool)
      }
      n33 = call "OBJ_SetI.vi"("value index IN"=0, "value IN"=0 ("Video channel"), "object handle IN"=w122) -> ()  [unwired: 2 out]
    }
    frame #3 {
      w143 = T17 0 items=["Grayscale (U8)", "Grayscale (I16)", "Grayscale (SGL)", "Complex (CSG)", "RGB (U32)", "HSL (U32)", "RGB (U64)"] ("Image Type")
      w151 = T17 0 items=["Grayscale (U8)", "Grayscale (I16)", "Grayscale (SGL)", "Complex (CSG)", "RGB (U32)", "HSL (U32)", "RGB (U64)"] ("Image Type")
      n34 = for "Create Greyscale map" {
        N: 256 -> [_]
        tunnel: [w157] -> w140 mode=indexing
        workers-P: _ -> [_]
        i -> [w160]
        n35 = To Unsigned Byte Integer(number=w160) -> (unsigned 8bit integer=w156:u8)
        n36 = Join Numbers(hi=w156, lo=w156) -> ((hi.lo)=w159:u16)
        n37 = Join Numbers(hi=w156, lo=w156) -> ((hi.lo)=w158:u16)
        n38 = Join Numbers(hi=w159, lo=w158) -> ((hi.lo)=w157:u32)
      }
      n39 = call "IMAQ Create"("Image Name"="Scaled video", "Image Type"=w143) -> ("New Image"=w142:T2)  [unwired: 2 in, 2 out]
      n40 = call "IMAQ Create"("Image Name"="Main video", "Image Type"=w151) -> ("New Image"=w152:T2)  [unwired: 2 in, 2 out]
      n41 = node-c288(0 ("Processor")) -> (w150:T14)  [unwired: 3 out]
      n42 = Initialize Array(u32 0 ("Window Number (0...15)"), 480 ("dimension size"), 640 ("dimension size")) -> (w145:u32[][])
      n43 = timed-loop {
        tunnel: w155 -> [w177]
        tunnel: [w176] -> w154
        tunnel: w152 -> [w175]
        timing: w150 -> [_]
        timing-out: [_] -> w149
        tunnel: w145 -> [w164]
        tunnel: w142 -> [w162]
        tunnel: w140 -> [w161]
        stop <- w163 stop-if-true
        # "This block performs the \nactual image capture."
        n44 = node-c288() -> ()  [unwired: 2 out]
        n45 = local read "Stop"() -> (w163:bool)
        n46 = Reciprocal(x="Video Capture Rate (Hz)") -> (1/x=w167:dbl)
        n47 = Multiply(x=w167, y=1000.0) -> (x*y=w165:dbl)
        n48 = call "DMR_ImageRequestWaitFor.vi"("queue number IN"=0, "timeout(ms) IN"=500, "driver handle IN"=w177) -> ("error code OUT"=w181:i32, "request number OUT"=w178:i32, "driver handle OUT"=w179:i32)
        n49 = feedback #1(T13 refnum ("Avi Refnum")) -> (w169:T13)
        n50 = case shown="True" "New Video File" {
          tunnel: [T13 refnum ("Avi Refnum") w198] -> w171
          tunnel: [FALSE TRUE] -> w172
          tunnel: w169 -> [_ w194]
          frame False {
          }
          frame True {
            n51 = call "Create new save file.vi"("Ext"=".avi" ("string"), "Index In"="Video Index") -> ("Path Out"=w190:path, "Index Out"=w191:dbl)  [unwired: 1 in]
            "Path Out" <- w190
            n52 = Not Equal?(x=w194, y=T13 refnum ("Avi Refnum")) -> (x != y?=w195:bool)
            n53 = Increment(x=w191) -> (x+1=w200:dbl)
            n54 = case shown="True" w195 {
              tunnel: w194 -> [_ w201]
              frame False {
              }
              frame True {
                n55 = call "IMAQ AVI Close"("Avi Refnum"=w201) -> ()  [unwired: 1 in, 10 out]
              }
            }
            n56 = local write "Video Index"(w200) -> ()
            n57 = call "IMAQ AVI Create"("Frames Per Second"=u32 30, "AVI Path"=w190) -> ("Avi Refnum"=w198:T13)  [unwired: 5 in, 4 out]
          }
        }
        n58 = Equal To 0?(x=w181) -> (x = 0?=w180:bool)
        n59 = Select(t=w171, s=w172, f=w169) -> (s? t:f=w170:T13)
        n60 = feedback-in #1(w170) -> ()
        n61 = case shown="True" w180 {
          tunnel: w179 -> [w202 w231]
          tunnel: w178 -> [_ w230]
          tunnel: [w202 w227] -> w176
          tunnel: w175 -> [_ w210]
          tunnel: w164 -> [_ w215]
          tunnel: w170 -> [_ w213]
          tunnel: w162 -> [_ w211]
          tunnel: w161 -> [_ w204]
          frame False {
          }
          frame True {
            w221 = u32 0 ("X-offset IN")
            n62 = call "DMR_GetImageRequestBufferData.vi"("driver handle IN"=w231, "request number IN"=w230) -> ("width OUT"=w220:i32, "height OUT"=w219:i32, "driver handle OUT"=w226:i32, "request number OUT"=w225:i32, "bytes per pixel OUT"=w222:i32)  [unwired: 13 out]
            n63 = call "DMR_GetImageRequestBufferImageData.vi"("driver handle IN"=w226, "request number IN"=w225, "bytes per pixel IN"=w222, "X-offset IN"=w221, "Y-offset IN"=w221, "height IN"=w219, "width IN"=w220) -> ("driver handle OUT"=w224:u32, "request number OUT"=w223:u32, "image OUT"=w216:u32[][])  [unwired: 10 out]
            n64 = call "DMR_ImageRequestUnlock.vi"("request number IN"=w223, "driver handle IN"=w224) -> ("driver handle OUT"=w229:i32)  [unwired: 1 in, 2 out]
            n65 = case shown="False" "Averaging" {
              tunnel: w216 -> [w307 w312]
              tunnel: [w307 w311] -> w212
              tunnel: w215 -> [_ w309]
              frame False {
              }
              frame True {
                (unwired) 1
                w317 = 1
                n66 = feedback #2(w309) -> (w308:u32[][])
                n67 = Add(x=w312, y=w308) -> (x+y=w313:u32[][])
                n68 = Select(t=w309, s="Reset Averaging", f=w313) -> (s? t:f=w315:u32[][])
                n69 = feedback-in #2(w315) -> ()
                n70 = feedback #3(w317) -> (w310:i32)
                n71 = Divide(x=w313, y=w310) -> (x/y=w314:dbl[][])
                n72 = Increment(x=w310) -> (x+1=w318:i32)
                n73 = To Unsigned Long Integer(number=w314) -> (unsigned 32bit integer=w311:u32[][])
                n74 = Select(t=w317, s="Reset Averaging", f=w318) -> (s? t:f=w316:i32)
                n75 = feedback-in #3(w316) -> ()
              }
            }
            n76 = call "DMR_ImageRequestSingle.vi"("request control IN"=0, "driver handle IN"=w229) -> ("driver handle OUT"=w227:i32)  [unwired: 3 out]
            n77 = disable-structure shown="Disabled" {
              disable-tunnel: w212 -> [w284 _]
              disable-tunnel: w211 -> [w283 _]
              frame Disabled {
                n78 = To Double Precision Float(number=w284) -> (double precision float=w282:dbl[][])
                n79 = In Range and Coerce(upper limit="Intensity Upper", x=w282, lower limit="Intensity Lower") -> (coerced(x)=w281:dbl[][])  [unwired: 1 out]
                n80 = Subtract(x="Intensity Upper", y="Intensity Lower") -> (x-y=w278:dbl)
                n81 = Subtract(x=w281, y="Intensity Lower") -> (x-y=w279:dbl[][])
                n82 = Divide(x=w279, y=w278) -> (x/y=w280:dbl[][])
                n83 = Multiply(x=255.0, y=w280) -> (x*y=w276:dbl[][])
                n84 = To Unsigned Byte Integer(number=w276) -> (unsigned 8bit integer=w285:u8[][])
                n85 = call "IMAQ ArrayToImage"("Image Pixels (U8)"=w285, "Image"=w283) -> ("Image Out"=w272:T2)  [unwired: 4 in, 5 out]
                n86 = First Call?() -> (First Call?: T/F=w273:bool)
                n87 = case shown="True" w273 {
                  tunnel: w272 -> [w286 w297]
                  frame False {
                    n88 = flat-sequence {
                      tunnel: w286 -> [w292]
                      frame #0 {
                        w289 = FALSE ("Get/Set Status? (Set)")
                        w288 = 0 ("Window Number (0...15)")
                        n89 = call "IMAQ WindSize"("Get/Set Status? (Set)"=w289, "Window Number"=w288) -> ("Width & Height out"=→"Window Size":cluster{"Width":i32, "Height":i32})  [unwired: 4 in, 2 out]
                        n90 = call "IMAQ WindMove"("Window Number (0...15)"=w288, "Get/Set Status? (Set)"=w289) -> ("Coordinates (screen)"=→"Window Position":cluster{"X Position":i32, "Y Position":i32})  [unwired: 3 in, 1 out]
                        n91 = call "IMAQ WindDraw"("Resize to Image Size? (Y)"=FALSE, "Window Number (0...15)"=w288, "Image"=w292) -> ()  [unwired: 7 in, 2 out]
                      }
                      frame #1 {
                        n92 = call "IMAQ WindZoom 2"("Center Point"="Center Point", "Zoom to Fit? (False)"=FALSE, "Zoom Factor"="Zoom Factor") -> ()  [unwired: 5 in, 4 out]
                      }
                    }
                  }
                  frame True {
                    n93 = flat-sequence {
                      tunnel: w297 -> [w300]
                      tunnel: [w298] -> w296
                      tunnel: w296 -> [w302]
                      frame #0 {
                        w299 = TRUE ("Resize to Image Size? (Y)")
                        w298 = 0 ("Window Number (0...15)")
                        n94 = call "IMAQ WindNonTearing"("Window Number"=w298, "NonTearing? (True)"=w299) -> ()  [unwired: 8 in, 2 out]
                        n95 = call "IMAQ WindDraw"("Resize to Image Size? (Y)"=w299, "Window Number (0...15)"=w298, "Image"=w300) -> ()  [unwired: 7 in, 2 out]
                      }
                      frame #1 {
                        n96 = call "IMAQ WindSize"("Scrollbars? (N)"=FALSE, "Width & Height"="Initial Window Size", "Window Number"=w302) -> ()  [unwired: 3 in, 3 out]
                        n97 = call "IMAQ WindMove"("Window Number (0...15)"=w302, "Coordinates (screen)"="Initial Window Position") -> ()  [unwired: 3 in, 2 out]
                      }
                    }
                  }
                }
              }
              frame Enabled {
              }
            }
            n98 = To Unsigned Byte Integer(number=w212) -> (unsigned 8bit integer=w203:u8[][])
            "image8bitArray" <- w203
            n99 = call "IMAQ ArrayToImage"("Image Pixels (U8)"=w203, "Image"=w210) -> ("Image Out"=w208:T2)  [unwired: 4 in, 5 out]
            n100 = case shown="True" "take fixed bead\n Images" {
              tunnel: w203 -> [_ w251]
              tunnel: w204 -> [_ w250]
              frame False {
              }
              frame True {
                n101 = local write "take fixed bead\n Images"(FALSE ("Save 10 Images")) -> ()
                n102 = while {
                  tunnel: w251 -> [w253]
                  tunnel: w250 -> [w252]
                  i -> [w255]
                  stop <- w254 stop-if-true
                  n103 = flat-sequence {
                    tunnel: w253 -> [w265]
                    tunnel: w252 -> [w264]
                    frame #0 {
                      n104 = local read "Image Index"() -> (w261:dbl)
                      n105 = call "Create new save file.vi"("Insert"="fixed_" ("string"), "Ext"=".bmp" ("string"), "Index In"=w261) -> ("Path Out"=w262:path, "Index Out"=w258:dbl)
                      n106 = call <vilib>:"Flatten Pixmap.vi"("colors"=w264, "8-bit pixmap"=w265) -> ("image data"=w263:T18)  [unwired: 4 in, 5 out]
                      n107 = Increment(x=w258) -> (x+1=w257:dbl)
                      n108 = call <vilib>:"Write BMP File.vi"("image data"=w263, "path to BMP file"=w262) -> ()  [unwired: 1 in, 9 out]
                      n109 = local write "Image Index"(w257) -> ()
                    }
                    frame #1 {
                      n110 = Wait (ms)(milliseconds to wait=u32 50) -> ()  [unwired: 1 out]
                    }
                  }
                  n111 = Equal?(x=w255, y=9) -> (x = y?=w254:bool)
                }
              }
            }
            n112 = case shown="True" "Save Video" {
              tunnel: w213 -> [_ w306]
              tunnel: w208 -> [_ w305]
              frame False {
              }
              frame True {
                n113 = call "IMAQ AVI Write Frame"("Image"=w305, "Avi Refnum"=w306) -> ()  [unwired: 2 in, 8 out]
              }
            }
            n114 = case shown="True" "take background images" {
              tunnel: w204 -> [_ w233]
              tunnel: w203 -> [_ w232]
              frame False {
              }
              frame True {
                n115 = while {
                  tunnel: w233 -> [w235]
                  tunnel: w232 -> [w234]
                  i -> [w238]
                  stop <- w236 stop-if-true
                  n116 = flat-sequence {
                    tunnel: w235 -> [w240]
                    tunnel: w234 -> [w239]
                    frame #0 {
                      n117 = local read "Image Index"() -> (w246:dbl)
                      n118 = call "Create new save file.vi"("Insert"="background_" ("string"), "Ext"=".bmp" ("string"), "Index In"=w246) -> ("Path Out"=w242:path, "Index Out"=w243:dbl)
                      n119 = call <vilib>:"Flatten Pixmap.vi"("colors"=w240, "8-bit pixmap"=w239) -> ("image data"=w241:T18)  [unwired: 4 in, 5 out]
                      n120 = Increment(x=w243) -> (x+1=w247:dbl)
                      n121 = local write "Image Index"(w247) -> ()
                      n122 = call <vilib>:"Write BMP File.vi"("image data"=w241, "path to BMP file"=w242) -> ()  [unwired: 1 in, 9 out]
                    }
                    frame #1 {
                      n123 = Wait (ms)(milliseconds to wait=u32 50) -> ()  [unwired: 1 out]
                    }
                  }
                  n124 = Equal?(x=w238, y=9) -> (x = y?=w236:bool)
                }
              }
            }
            n125 = case shown="False" "Target" {
              tunnel: w208 -> [w267 w271]
              tunnel: [w267 w269] -> w207
              frame False {
              }
              frame True {
                n126 = local read "Target coordinates"() -> (w268:cluster{"X1":dbl, "Y1":dbl, "X2":dbl, "Y2":dbl})
                n127 = call "IMAQ Overlay Oval"("Color"=u32 16711680, "Bounding Rectangle"=w268, "Image"=w271) -> ("Image Out"=w269:T2)  [unwired: 7 in, 1 out]
              }
            }
            "Primary Video Display" <- w207
            n128 = case shown="True" "Save Image" {
              tunnel: w203 -> [_ w321]
              tunnel: w204 -> [_ w320]
              frame False {
              }
              frame True {
                n129 = call <vilib>:"Flatten Pixmap.vi"("colors"=w320, "8-bit pixmap"=w321) -> ("image data"=w327:T18)  [unwired: 4 in, 5 out]
                n130 = call "Create new save file.vi"("Insert"="video_frame_" ("string"), "Ext"=".bmp" ("string"), "Index In"="Image Index") -> ("Path Out"=w323:path, "Index Out"=w328:dbl)
                n131 = Increment(x=w328) -> (x+1=w322:dbl)
                n132 = local write "Image Index"(w322) -> ()
                n133 = call <vilib>:"Write BMP File.vi"("image data"=w327, "path to BMP file"=w323) -> ()  [unwired: 1 in, 9 out]
              }
            }
            "GreyscaleArray" <- w204
          }
        }
        n134 = node-c288(w165) -> ()  [unwired: 1 out]
      }
      n135 = node-c288(w149) -> ()  [unwired: 1 out]
      n136 = call "DMR_CloseDevice2.vi"("driver handle IN"=w154) -> ()  [unwired: 3 in, 2 out]
    }
    frame #4 {
      n137 = call "DMR_Close.vi"() -> ()  [unwired: 1 out]
    }
  }
  n138 = while {
    tunnel: [w402] -> w84
    tunnel: [w576] -> w85
    tunnel: [w400] -> w83
    tunnel: [w684] -> w80
    tunnel: w38 -> [w387]
    tunnel: w37 -> [w680]
    tunnel: w36 -> [w685]
    stop <- w684 stop-if-true
    w439 = "NI_ChannelName" ("name")
    w343 = "NI_ChannelName" ("name")
    w504 = -1
    # "Negate these value to make Force feedback work in X. 6-14-18 A.T."
    # "BX - AX"
    # "BY - AY"
    # "Scan # counter"
    # "DAQ loop iteration\ncounter (for timing)"
    # "Step counter"
    # "Force feedback"
    # "Raster scan"
    # "Rewire everything"
    # "Invert these because changed\nfrom PSD to QPD"
    # "Trap Y"
    # "Trap X"
    # "Convert to\npN"
    # "Convert to\nnm"
    # "Subtract\noffset"
    # "Normalize by\nsum"
    # "B sum"
    # "BX"
    # "BY"
    # "AX"
    # "AY"
    # "A sum"
    # "Close files when done saving"
    n139 = disable-structure shown="Disabled" {
      frame Disabled {
        n140 = property class="DAQmx Read"() -> ("AvailSampPerChan"=→"AvailSampPerChan 2":u32)  [unwired: 2 in, 2 out]
      }
      frame Enabled {
      }
    }
    n141 = local read "Averaging Number"() -> (w410:i32)
    n142 = local read "Averaging Number"() -> (w412:i32)
    "# Samples/channel" <- w412
    n143 = local read "Sampling Rate"() -> (w683:dbl)
    n144 = call-poly <vilib>:"DAQmx Read.vi"("task/channels in"=w387, "number of samples per channel"=w410, "timeout"=10.0) -> ("task out"=w386:refnum<k21>, "data"=w411:dbl[][], "error out"=w505:errorcluster)  [unwired: 10 in]
    n145 = Unbundle By Name(w505) -> ("status"=w624:bool)
    n146 = Divide(x=w683, y="Cal Averaging") -> (x/y=→"Cal Final Sampling Rate":dbl)
    n147 = Divide(x=w683, y=w412) -> (x/y=→"Final Sampling Rate" →"# Samples/channel/s":dbl)
    n148 = Index Array(array=w411, index (row)=4) -> (element=w501:dbl[])  [unwired: 1 in]
    n149 = disable-structure shown="Disabled" {
      frame Disabled {
        n150 = local read "Buffer size\n(Samples/channel)"() -> (w702:u32)
        n151 = property class="DAQmx Read"() -> ("AvailSampPerChan"=w703:u32)  [unwired: 2 in, 2 out]
        "AvailSampPerChan" <- w703
        n152 = Divide(x=w703, y=w702) -> (x/y=→"Buffer status":dbl)
      }
      frame Enabled {
      }
    }
    n153 = Index Array(array=w411, index (row)=5) -> (element=w500:dbl[])  [unwired: 1 in]
    n154 = Index Array(array=w411, index (row)=0) -> (element=w362:dbl[])  [unwired: 1 in]
    n155 = Index Array(array=w411, index (row)=3) -> (element=w361:dbl[])  [unwired: 1 in]
    n156 = Index Array(array=w411, index (row)=1) -> (element=w360:dbl[])  [unwired: 1 in]
    n157 = Index Array(array=w411, index (row)=7) -> (element=w358:dbl[])  [unwired: 1 in]
    n158 = Index Array(array=w411, index (row)=2) -> (element=w363:dbl[])  [unwired: 1 in]
    n159 = Index Array(array=w411, index (row)=6) -> (element=w359:dbl[])  [unwired: 1 in]
    n160 = case shown="True" w624 {
      frame False {
      }
      frame True {
        n161 = call <vilib>:"Beep.vi"() -> ()  [unwired: 12 in]
        "Buffer Overflow" <- TRUE
      }
    }
    n162 = Divide(x=w363, y=w359) -> (x/y=w357:dbl[])
    n163 = Divide(x=w362, y=w359) -> (x/y=w356:dbl[])
    n164 = Divide(x=w361, y=w358) -> (x/y=w355:dbl[])
    n165 = Divide(x=w360, y=w358) -> (x/y=w354:dbl[])
    n166 = local read "Cal values"() -> (w616:T3)
    n167 = Build Array(w357, w356, w355, w354) -> (w353:dbl[][])
    n168 = Unbundle(w616) -> ("AX alpha"=w604:dbl, "BX alpha"=w600:dbl, "AX kappa"=w596:dbl, "BX kappa"=w592:dbl, "AX offset"=w610:dbl, "BX offset"=w608:dbl, "AY alpha"=w607:dbl, "BY alpha"=w602:dbl, "AY kappa"=w598:dbl, "BY kappa"=w594:dbl, "AY offset"=w614:dbl, "BY offset"=w612:dbl)
    n169 = Multiply(x=w360, y=w504) -> (x*y=w502:dbl[])
    n170 = Multiply(x=w362, y=w504) -> (x*y=w503:dbl[])
    n171 = local write "AX alpha"(w604) -> ()
    n172 = local write "BY offset"(w612) -> ()
    n173 = Build Array(w503, w363, w502, w361, w359, w358, w501, w500) -> (w436:dbl[][])
    n174 = local write "BX alpha"(w600) -> ()
    n175 = case shown="True" "Reset data stream" {
      selector: "Reset data stream" -> [_ w851]
      tunnel: w386 -> [w843 w849]
      tunnel: [w843 w847] -> w576
      tunnel: w505 -> [w842 w846]
      tunnel: [w842 w844] -> _
      frame False {
      }
      frame True {
        n176 = Not(x=w851) -> (.not. x?=w850:bool)
        n177 = call <vilib>:"DAQmx Stop Task.vi"("task/channels in"=w849, "error in"=w846) -> ("task out"=w848:refnum<k21>, "error out"=w845:errorcluster)  [unwired: 12 in]
        n178 = local write "Reset data stream"(w850) -> ()
        n179 = local write "Buffer Overflow"(w850) -> ()
        n180 = call <vilib>:"DAQmx Start Task.vi"("task/channels in"=w848, "error in"=w845) -> ("task out"=w847:refnum<k21>, "error out"=w844:errorcluster)  [unwired: 12 in]
      }
    }
    n181 = call-poly <vilib>:"Mean.vi"("X"=w500) -> ("mean"=w630:dbl)  [unwired: 1 out]
    n182 = local write "AY offset"(w614) -> ()
    n183 = call-poly <vilib>:"Mean.vi"("X"=w501) -> ("mean"=w631:dbl)  [unwired: 1 out]
    n184 = call-poly <vilib>:"Mean.vi"("X"=w363) -> ("mean"=w637:dbl)  [unwired: 1 out]
    n185 = call-poly <vilib>:"Mean.vi"("X"=w361) -> ("mean"=w635:dbl)  [unwired: 1 out]
    n186 = call-poly <vilib>:"Mean.vi"("X"=w359) -> ("mean"=w634:dbl)  [unwired: 1 out]
    n187 = call-poly <vilib>:"Mean.vi"("X"=w358) -> ("mean"=w633:dbl)  [unwired: 1 out]
    n188 = local read "Averaging Number"() -> (w409:i32)
    n189 = local write "BY kappa"(w594) -> ()
    n190 = local write "AX kappa"(w596) -> ()
    n191 = call-poly <vilib>:"Mean.vi"("X"=w502) -> ("mean"=w636:dbl)  [unwired: 1 out]
    n192 = local write "AY kappa"(w598) -> ()
    n193 = call-poly <vilib>:"Mean.vi"("X"=w503) -> ("mean"=w638:dbl)  [unwired: 1 out]
    n194 = local read "DAQ rate\n(Samples/s)"() -> (w415:dbl)
    n195 = Build Array(w631, w630) -> (w629:dbl[])
    n196 = local write "BX kappa"(w592) -> ()
    n197 = local write "BY alpha"(w602) -> ()
    n198 = local write "AX offset"(w610) -> ()
    n199 = local write "BX offset"(w608) -> ()
    n200 = local write "AY alpha"(w607) -> ()
    n201 = Build Array(w638, w637, w636, w635, w634, w633) -> (w627:dbl[])
    n202 = local read "Total raster time (s)"() -> (w383:dbl)
    n203 = local read "offset ffb param"() -> (w333:T1)
    n204 = Divide(x=w409, y=w415) -> (x/y=w379:dbl)
    "Data update period (s/set)" <- w379
    n205 = Reciprocal(x=w415) -> (1/x=w416:dbl)
    "Data period (s)" <- w416
    n206 = Divide(x=w383, y=w379) -> (x/y=w382:dbl)
    n207 = Divide(x="Cal time (s)", y=w379) -> (x/y=w378:dbl)
    n208 = Divide(x=w638, y=w634) -> (x/y=w668:dbl)
    n209 = Divide(x=w637, y=w634) -> (x/y=w374:dbl)
    n210 = Round Toward -Infinity(1:w382) -> (0:w381:dbl)
    n211 = Divide(x=w636, y=w633) -> (x/y=w675:dbl)
    n212 = Divide(x=w635, y=w633) -> (x/y=w376:dbl)
    n213 = Round Toward -Infinity(1:w378) -> (0:→"Cal sets to save":dbl)
    n214 = local write "N sets to be saved"(w381) -> ()
    n215 = Build Array("Force Feedback 1", "Force Feedback 2") -> (w339:bool[])
    n216 = Boolean Array To Number(Boolean array=w339) -> (number=w338:u32)
    n217 = Negate(x=w374) -> (-x=w373:dbl)
    n218 = Negate(x=w376) -> (-x=w375:dbl)
    n219 = Subtract(x=w668, y="AY offset") -> (x-y=w650:dbl)
    n220 = Subtract(x=w374, y="AX offset") -> (x-y=w651:dbl)
    n221 = Subtract(x=w675, y="BY offset") -> (x-y=w649:dbl)
    n222 = Subtract(x=w376, y="BX offset") -> (x-y=w652:dbl)
    n223 = Subtract(x=w675, y=w668) -> (x-y=w666:dbl)
    n224 = Subtract(x=w375, y=w373) -> (x-y=w667:dbl)
    n225 = feedback #4(0.0) -> (w575:dbl)
    n226 = Multiply(x="Downsamp\nfact", y=w416) -> (x*y=w351:dbl)
    n227 = Multiply(x=w650, y="AY alpha") -> (x*y=w584:dbl)
    n228 = Multiply(x=w651, y="AX alpha") -> (x*y=w582:dbl)
    n229 = Multiply(x=w652, y="BX alpha") -> (x*y=w583:dbl)
    n230 = Multiply(x=w649, y="BY alpha") -> (x*y=w585:dbl)
    n231 = Add(x=w379, y=w575) -> (x+y=w573:dbl)
    n232 = feedback-in #4(w573) -> ()
    n233 = Square(x=w584) -> (x^2=w660:dbl)
    n234 = Square(x=w582) -> (x^2=w661:dbl)
    n235 = Square(x=w585) -> (x^2=w662:dbl)
    n236 = Square(x=w583) -> (x^2=w663:dbl)
    n237 = Bundle(w666, w667) -> (w370:cluster{dbl, dbl})  [unwired: 1 in]
    n238 = case shown="True" "Set reading to\nsetpoint 1" {
      tunnel: w370 -> [_ w840]
      frame False {
      }
      frame True {
        n239 = property on="Setpoint voltage 1" class="Clust (strict)"("Val(Sgnl)"=w840) -> ()  [unwired: 2 in, 2 out]
        n240 = local read "Trap position (V)"() -> (w839:cluster{"X":dbl, "Y":dbl})
        n241 = local write "Set reading to\nsetpoint 1"(FALSE ("Set reading to\nsetpoint")) -> ()
        n242 = Unbundle(w839) -> ("X"=w838:dbl, "Y"=w837:dbl)
        n243 = Bundle("Y"=w837, "X"=w838) -> (w836:cluster{"Y":dbl, "X":dbl})  [unwired: 1 in]
        n244 = property on="Offset 1" class="Clust (strict)"("Val(Sgnl)"=w836) -> ()  [unwired: 2 in, 2 out]
      }
    }
    n245 = Reciprocal(x=w351) -> (1/x=→"Chart Freq (Hz)":dbl)
    n246 = To Time Stamp(1:w573) -> (0:w350:timestamp)
    n247 = Add(x=w660, y=w661) -> (x+y=w664:dbl)
    n248 = Add(x=w662, y=w663) -> (x+y=w674:dbl)
    n249 = Multiply(x=w582, y="AX kappa") -> (x*y=w578:dbl)
    n250 = Bundle("A y", "A x", "B y", "B x", "A sum", "B sum", "Trap x", "Trap y") -> (w564:T21)  [unwired: 1 in]
    n251 = Multiply(x=w583, y="BX kappa") -> (x*y=w579:dbl)
    n252 = Square Root(x=w664) -> (sqrt(x)=w678:dbl)
    n253 = Square Root(x=w674) -> (sqrt(x)=w677:dbl)
    n254 = Multiply(x=w584, y="AY kappa") -> (x*y=w580:dbl)
    n255 = Multiply(x=w585, y="BY kappa") -> (x*y=w581:dbl)
    n256 = Subtract(x=w630, y="Fixed Y") -> (x-y=w665:dbl)
    n257 = Subtract(x=w631, y="Fixed X") -> (x-y=w669:dbl)
    n258 = Cluster To Array(cluster=w564) -> (array=w563:string[])
    n259 = for {
      tunnel: w436 -> [w829] mode=indexing
      tunnel: w351 -> [w828]
      tunnel: "Downsamp\nfact" -> [w834]
      tunnel: [w832] -> w369 mode=indexing
      tunnel: w350 -> [w835]
      tunnel: w563 -> [w831] mode=indexing
      tunnel: w343 -> [w830]
      n260 = call "Downsample 1D array.vi"("Ave N"=w834, "Arrray In"=w829) -> ("Array Out"=w827:dbl[])  [unwired: 9 in]
      n261 = Bundle By Name("Y"=w827, "dt"=w828, "t0"=w835) -> (w833:waveform(dbl))  [unwired: 1 in]
      n262 = Set Waveform Attribute(5:w831, 6:w830, 7:w833) -> (3:w832:waveform(dbl))  [unwired: 1 in, 2 out]
    }
    "All signals" <- w369
    n263 = Square(x=w580) -> (x^2=w653:dbl)
    n264 = Square(x=w578) -> (x^2=w654:dbl)
    n265 = Square(x=w581) -> (x^2=w655:dbl)
    n266 = Square(x=w579) -> (x^2=w656:dbl)
    n267 = Add(x=w653, y=w654) -> (x+y=w657:dbl)
    n268 = Add(x=w655, y=w656) -> (x+y=w658:dbl)
    n269 = Multiply(x=w665, y="Conv Y (nm/V)") -> (x*y=w587:dbl)
    n270 = Multiply(x=w669, y="Conv X (nm/V)") -> (x*y=w588:dbl)
    n271 = feedback #5() -> (w625:cluster{"B_Y":dbl, "B_X":dbl})  [unwired: 1 in]
    n272 = case shown="1" w338 {
      tunnel: [w1188 w1206 w1216] -> w403
      tunnel: [w1187 w1205 w1217] -> w401
      tunnel: w370 -> [_ w1204 w1219]
      tunnel: [cluster{"B_Y":dbl, "B_X":dbl} {"B_Y"=0.0, "B_X"=0.0} ("Sum error past") w1198 w1214] -> w626
      tunnel: w625 -> [_ w1203 w1215]
      tunnel: w680 -> [w1188 w1201 w1210]
      tunnel: w685 -> [w1187 w1200 w1218]
      tunnel: [0.0 ("B_X") w1193 w1208] -> w336
      tunnel: [cluster{"B_Y":dbl, "B_X":dbl} {"B_Y"=0.0, "B_X"=0.0} ("Sum error past") w1192 w1207] -> w335
      tunnel: "Feedback const" -> [_ w1191 w1209]
      tunnel: w333 -> [_ w1190 _]
      frame 0, Default {
        # "Force feedback"
      }
      frame 1 {
        n273 = local write "Force Feedback 2"(FALSE) -> ()
        n274 = call "ForceFeedback3_offset.vi"("Current Voltage(B-A)"=w1204, "offset ffb param"=w1190, "Sum error"=w1203, "task/channels in"=w1201, "error in"=w1200, "Setpoint/Desired Voltage"="Setpoint voltage 1", "Feedback const"=w1191, "offset voltage"="Offset 1") -> ("task out"=w1206:refnum<k21>, "Sum error past"=w1198:cluster{"B_Y":dbl, "B_X":dbl}, "Output Voltage"=w1192:cluster{dbl, dbl}, "error out"=w1205:errorcluster)  [unwired: 7 in, 1 out]
        n275 = local read "Pulling direction"() -> (w1197:bool)
        n276 = Unbundle(w1198) -> ("B_Y"=w1196:dbl, "B_X"=w1195:dbl)
        n277 = Select(t=w1196, s=w1197, f=w1195) -> (s? t:f=w1193:dbl)
      }
      frame 2 {
        n278 = local write "Force Feedback 1"(FALSE) -> ()
        n279 = call "ForceFeedback3_offset.vi"("Current Voltage(B-A)"=w1219, "Sum error"=w1215, "task/channels in"=w1210, "error in"=w1218, "Setpoint/Desired Voltage"="Setpoint voltage 2", "Feedback const"=w1209, "offset voltage"="Offset 2") -> ("task out"=w1216:refnum<k21>, "Sum error past"=w1214:cluster{"B_Y":dbl, "B_X":dbl}, "Output Voltage"=w1207:cluster{dbl, dbl}, "error out"=w1217:errorcluster)  [unwired: 8 in, 1 out]
        n280 = local read "Pulling direction"() -> (w1211:bool)
        n281 = Unbundle(w1214) -> ("B_Y"=w1213:dbl, "B_X"=w1212:dbl)
        n282 = Select(t=w1213, s=w1211, f=w1212) -> (s? t:f=w1208:dbl)
      }
    }
    "Sum error" <- w336
    "Feedback Output \nVoltage 2" <- w335
    n283 = feedback-in #5(w626) -> ()
    n284 = Square Root(x=w657) -> (sqrt(x)=w586:dbl)
    n285 = Square Root(x=w658) -> (sqrt(x)=w679:dbl)
    n286 = Add(x=w586, y=w679) -> (x+y=w659:dbl)
    n287 = case shown="True" "Set reading to\nsetpoint 2" {
      tunnel: w370 -> [_ w697]
      frame False {
      }
      frame True {
        n288 = local read "Trap position (V)"() -> (w700:cluster{"X":dbl, "Y":dbl})
        n289 = property on="Setpoint voltage 2" class="Clust (strict)"("Val(Sgnl)"=w697) -> ()  [unwired: 2 in, 2 out]
        n290 = local write "Set reading to\nsetpoint 2"(FALSE) -> ()
        n291 = Unbundle(w700) -> ("X"=w699:dbl, "Y"=w698:dbl)
        n292 = Bundle("Y"=w698, "X"=w699) -> (w696:cluster{"Y":dbl, "X":dbl})  [unwired: 1 in]
        n293 = property on="Offset 2" class="Clust (strict)"("Val(Sgnl)"=w696) -> ()  [unwired: 2 in, 2 out]
      }
    }
    n294 = Build Array(w668, w374, w675, w376, w634, w633, w586, w679, w678, w677, w588, w587) -> ()  [unwired: 1 out]
    n295 = Divide(x=w659, y=2.0) -> (x/y=w623:dbl)
    n296 = Bundle("AX/Asum", "AY/Asum", "BX/Bsum", "BY/Bsum") -> (w345:cluster{string, string, string, string})  [unwired: 1 in]
    n297 = Index Array(array=w369, index=6) -> (element=w441:waveform(dbl))
    n298 = Index Array(array=w369, index=7) -> (element=w443:waveform(dbl))
    n299 = Cluster To Array(cluster=w345) -> (array=w344:string[])
    n300 = for {
      tunnel: w353 -> [w695] mode=indexing
      tunnel: "Downsamp\nfact" -> [w694]
      tunnel: w351 -> [w693]
      tunnel: w350 -> [w691]
      tunnel: w344 -> [w689] mode=indexing
      tunnel: w343 -> [w688]
      tunnel: [w687] -> w342 mode=indexing
      n301 = call "Downsample 1D array.vi"("Ave N"=w694, "Arrray In"=w695) -> ("Array Out"=w692:dbl[])  [unwired: 9 in]
      n302 = Bundle By Name("Y"=w692, "dt"=w693, "t0"=w691) -> (w690:waveform(dbl))  [unwired: 1 in]
      n303 = Set Waveform Attribute(5:w689, 6:w688, 7:w690) -> (3:w687:waveform(dbl))  [unwired: 1 in, 2 out]
    }
    "All signals 2" <- w342
    n304 = local read "Fixed X"() -> (w490:dbl)
    n305 = local read "Fixed Y"() -> (w492:dbl)
    n306 = Unbundle By Name(w441) -> ("Y"=w494:dbl[])
    n307 = Unbundle By Name(w443) -> ("Y"=w493:dbl[])
    n308 = Index Array(array=w369, index=0) -> (element=w448:waveform(dbl))
    n309 = Index Array(array=w369, index=1) -> (element=w560:waveform(dbl))
    n310 = Index Array(array=w369, index=4) -> (element=w554:waveform(dbl))
    n311 = Subtract(x=w494, y=w490) -> (x-y=w491:dbl[])
    n312 = Subtract(x=w493, y=w492) -> (x-y=w488:dbl[])
    n313 = Unbundle By Name(w448) -> ("Y"=w552:dbl[])
    n314 = Unbundle By Name(w560) -> ("Y"=w551:dbl[])
    n315 = Unbundle By Name(w554) -> ("Y"=w550:dbl[])
    n316 = Index Array(array=w369, index=5) -> (element=w553:waveform(dbl))
    n317 = local read "Conv X (nm/V)"() -> (w489:dbl)
    n318 = local read "Conv Y (nm/V)"() -> (w487:dbl)
    n319 = Index Array(array=w369, index=2) -> (element=w364:waveform(dbl))
    n320 = Index Array(array=w369, index=3) -> (element=w557:waveform(dbl))
    n321 = Set Waveform Attribute(5:"T2 X", 6:w439, 7:w441) -> (3:w440:waveform(dbl))  [unwired: 1 in, 2 out]
    n322 = Set Waveform Attribute(5:"T2 Y", 6:w439, 7:w443) -> (3:w442:waveform(dbl))  [unwired: 1 in, 2 out]
    n323 = Unbundle By Name(w553) -> ("Y"=w547:dbl[])
    n324 = Unbundle By Name(w364) -> ("Y"=w549:dbl[])
    n325 = Unbundle By Name(w557) -> ("Y"=w548:dbl[])
    n326 = Divide(x=w552, y=w550) -> (x/y=w368:dbl[])
    n327 = Divide(x=w551, y=w550) -> (x/y=w367:dbl[])
    n328 = local read "AY offset"() -> (w538:dbl)
    n329 = local read "AX offset"() -> (w536:dbl)
    n330 = Multiply(x=w491, y=w489) -> (x*y=w433:dbl[])
    n331 = Multiply(x=w488, y=w487) -> (x*y=w435:dbl[])
    n332 = Divide(x=w548, y=w547) -> (x/y=w365:dbl[])
    n333 = Subtract(x=w367, y=w536) -> (x-y=w539:dbl[])
    n334 = local read "BX offset"() -> (w546:dbl)
    n335 = Subtract(x=w368, y=w538) -> (x-y=w540:dbl[])
    n336 = Divide(x=w549, y=w547) -> (x/y=w366:dbl[])
    n337 = local read "AY alpha"() -> (w537:dbl)
    n338 = local read "AX alpha"() -> (w535:dbl)
    n339 = call-poly <vilib>:"Mean.vi"("X"=w435) -> ("mean"=w470:dbl)  [unwired: 1 out]
    "Mean Trp Pos Y 2 (nm)" <- w470
    n340 = Subtract(x=w366, y=w368) -> (x-y=w460:dbl[])
    n341 = Subtract(x=w365, y=w367) -> (x-y=w459:dbl[])
    n342 = local read "BY offset"() -> (w543:dbl)
    n343 = Subtract(x=w433, y="Offset X (nm)") -> (x-y=w432:dbl[])
    n344 = Subtract(x=w435, y="Offset Y (nm)") -> (x-y=w434:dbl[])
    n345 = Subtract(x=w366, y=w543) -> (x-y=w545:dbl[])
    n346 = Subtract(x=w365, y=w546) -> (x-y=w544:dbl[])
    n347 = Subtract(x=w470, y=w435) -> (x-y=w469:dbl[])
    n348 = call-poly <vilib>:"Mean.vi"("X"=w433) -> ("mean"=w474:dbl)  [unwired: 1 out]
    "Mean Trap Pos X 2 (nm)" <- w474
    n349 = Build Array(w460, w459) -> (w457:dbl[][])
    n350 = Index Array(array=w457, index (row)=0) -> (element=w455:dbl[])  [unwired: 1 in]
    n351 = Index Array(array=w457, index (row)=1) -> (element=w454:dbl[])  [unwired: 1 in]
    n352 = call-poly <vilib>:"Mean.vi"("X"=w455) -> ("mean"=w453:dbl)  [unwired: 1 out]
    n353 = call-poly <vilib>:"Mean.vi"("X"=w454) -> ("mean"=w452:dbl)  [unwired: 1 out]
    n354 = Bundle("mean"=w453, "mean"=w452) -> ()  [unwired: 1 in, 1 out]
    n355 = local read "BX alpha"() -> (w541:dbl)
    n356 = Multiply(x=w540, y=w537) -> (x*y=w528:dbl[])
    n357 = Multiply(x=w539, y=w535) -> (x*y=w527:dbl[])
    n358 = Square(x=w469) -> (x^2=w468:dbl[])
    n359 = Subtract(x=w474, y=w433) -> (x-y=w473:dbl[])
    n360 = Bundle By Name(cluster=w442, "Y"=w434) -> (w485:waveform(dbl))
    n361 = Bundle By Name(cluster=w440, "Y"=w432) -> (w486:waveform(dbl))
    n362 = local read "BY alpha"() -> (w542:dbl)
    n363 = local read "Raster scanning..."() -> (w385:bool)
    n364 = local read "Saving"() -> (w589:bool)
    n365 = local read "Tether"() -> (w590:bool)
    n366 = Square(x=w473) -> (x^2=w472:dbl[])
    n367 = call-poly <vilib>:"Mean.vi"("X"=w468) -> ("mean"=w467:dbl)  [unwired: 1 out]
    n368 = Square(x=w528) -> (x^2=w534:dbl[])
    n369 = Multiply(x=w545, y=w542) -> (x*y=w526:dbl[])
    n370 = Square(x=w527) -> (x^2=w533:dbl[])
    n371 = Multiply(x=w544, y=w541) -> (x*y=w525:dbl[])
    n372 = Less?(x=w623, y="Tether break\nforce (pN)") -> (x < y?=w621:bool)
    n373 = call-poly <vilib>:"Mean.vi"("X"=w472) -> ("mean"=w471:dbl)  [unwired: 1 out]
    n374 = Build Array(w486, w485) -> (w404:waveform(dbl)[])
    "Trap sep" <- w404
    n375 = Square Root(x=w467) -> (sqrt(x)=w466:dbl)
    n376 = Square(x=w526) -> (x^2=w532:dbl[])
    n377 = Square(x=w525) -> (x^2=w531:dbl[])
    n378 = Add(x=w534, y=w533) -> (x+y=w530:dbl[])
    n379 = Square Root(x=w471) -> (sqrt(x)=w464:dbl)
    n380 = Compound Arithmetic op=AND(w589, w590, w621) -> (w620:bool)
    n381 = Multiply(x=w466, y=10) -> (x*y=→"T2 Y RMS (A)":dbl)
    n382 = Square Root(x=w530) -> (sqrt(x)=w428:dbl[])
    n383 = Add(x=w532, y=w531) -> (x+y=w529:dbl[])
    n384 = Set Waveform Attribute(5:"T2", 6:"NI_ChannelName" ("name"), 7:w448) -> (3:w447:waveform(dbl))  [unwired: 1 in, 2 out]
    n385 = Set Waveform Attribute(5:"T1", 6:"NI_ChannelName" ("name"), 7:w364) -> (3:w445:waveform(dbl))  [unwired: 1 in, 2 out]
    n386 = case shown="True" w620 {
      selector: w620 -> [_ w858]
      tunnel: w385 -> [w852 w854]
      tunnel: [w852 w854] -> w384
      frame False {
      }
      frame True {
        n387 = flat-sequence {
          frame #0 {
            n388 = local write "Cancel Rep\n Dip"(TRUE) -> ()
          }
          frame #1 {
            n389 = local write "Cancel Rep\n Dip"(FALSE ("Cancel Rep\n Dip")) -> ()
          }
        }
        n390 = call <vilib>:"Beep.vi"() -> ()  [unwired: 12 in]
        n391 = Not(x=w858) -> (.not. x?=w853:bool)
        n392 = And(x=w854, y="Fish After TA?") -> (x .and. y?=w856:bool)
        n393 = local write "Force Feedback 1"(w853) -> ()
        n394 = local write "Tether"(w853) -> ()
        n395 = case shown="True" w856 {
          selector: w856 -> [_ w861]
          frame False {
          }
          frame True {
            n396 = property on="Fish" class="Bool (strict)"("Val(Sgnl)"=w861) -> ()  [unwired: 2 in, 2 out]
          }
        }
        n397 = local write "Force Feedback 2"(w853) -> ()
        n398 = property on="Stop saving" class="Bool (strict)"("Val(Sgnl)"="TA Cancel Save?") -> ()  [unwired: 2 in, 2 out]
      }
    }
    n399 = Square Root(x=w529) -> (sqrt(x)=w427:dbl[])
    n400 = Multiply(x=w464, y=10) -> (x*y=→"T2 X RMS (A)":dbl)
    n401 = Bundle By Name(cluster=w447, "Y"=w428) -> (w451:waveform(dbl))
    n402 = Bundle By Name(cluster=w445, "Y"=w427) -> (w507:waveform(dbl))
    n403 = Add(x=w428, y=w427) -> (x+y=w426:dbl[])
    n404 = case shown="True" "Remove offsets" {
      selector: "Remove offsets" -> [_ w825]
      frame False {
      }
      frame True {
        n405 = local read "Mean Trp Pos Y 2 (nm)"() -> (w823:dbl)
        n406 = Not(x=w825) -> (.not. x?=w826:bool)
        n407 = local read "Mean Trap Pos X 2 (nm)"() -> (w824:dbl)
        n408 = local write "Remove offsets"(w826) -> ()
        n409 = local write "Offset Y (nm)"(w823) -> ()
        n410 = local write "Offset X (nm)"(w824) -> ()
      }
    }
    n411 = Build Array(w451, w507) -> (→"Bead sep":waveform(dbl)[])
    n412 = local read "AY kappa"() -> (w524:dbl)
    n413 = local read "AX kappa"() -> (w523:dbl)
    n414 = Divide(x=w426, y=2) -> (x/y=w424:dbl[])
    n415 = local read "BX kappa"() -> (w521:dbl)
    n416 = local read "BY kappa"() -> (w522:dbl)
    n417 = call-poly <vilib>:"Mean.vi"("X"=w424) -> ("mean"=w423:dbl)  [unwired: 1 out]
    "Mean Bead Sep\n(nm)" <- w423
    n418 = local read "Calibrating"() -> (w337:bool)
    n419 = Multiply(x=w528, y=w524) -> (x*y=w517:dbl[])
    n420 = Multiply(x=w527, y=w523) -> (x*y=w518:dbl[])
    n421 = Square(x=w517) -> (x^2=w516:dbl[])
    n422 = Square(x=w518) -> (x^2=w515:dbl[])
    n423 = Subtract(x=w424, y=w423) -> (x-y=w422:dbl[])
    n424 = Multiply(x=w526, y=w522) -> (x*y=w519:dbl[])
    n425 = Multiply(x=w525, y=w521) -> (x*y=w520:dbl[])
    n426 = Or(x=w384, y="Raster scan") -> (x .or. y?=w399:bool)
    n427 = Add(x=w516, y=w515) -> (x+y=w512:dbl[])
    n428 = Square(x=w422) -> (x^2=w421:dbl[])
    n429 = call-poly <vilib>:"Mean.vi"("X"=w421) -> ("mean"=w420:dbl)  [unwired: 1 out]
    n430 = Square Root(x=w512) -> (sqrt(x)=w484:dbl[])
    n431 = Square(x=w519) -> (x^2=w514:dbl[])
    n432 = Square(x=w520) -> (x^2=w513:dbl[])
    n433 = Add(x=w514, y=w513) -> (x+y=w511:dbl[])
    n434 = Bundle By Name(cluster=w447, "Y"=w484) -> (w510:waveform(dbl))
    n435 = Square Root(x=w511) -> (sqrt(x)=w483:dbl[])
    n436 = local read "Saving"() -> (w619:bool)
    n437 = Or(x=w337, y=w619) -> ()  [unwired: 1 out]
    n438 = Square Root(x=w420) -> (sqrt(x)=w419:dbl)
    n439 = Multiply(x=10, y=w419) -> (x*y=→"Bead Sep Noise\n(A)":dbl)
    n440 = Bundle By Name(cluster=w445, "Y"=w483) -> (w509:waveform(dbl))
    n441 = Add(x=w484, y=w483) -> (x+y=w482:dbl[])
    n442 = Build Array(w510, w509) -> (→"Force (pN)":waveform(dbl)[])
    n443 = Divide(x=w482, y=2) -> (x/y=w479:dbl[])
    n444 = call-poly <vilib>:"Mean.vi"("X"=w479) -> ("mean"=w480:dbl)  [unwired: 1 out]
    "Mean force (pN)" <- w480
    n445 = Subtract(x=w480, y=w479) -> (x-y=w478:dbl[])
    n446 = Square(x=w478) -> (x^2=w477:dbl[])
    n447 = call-poly <vilib>:"Mean.vi"("X"=w477) -> ("mean"=w476:dbl)  [unwired: 1 out]
    n448 = flat-sequence {
      tunnel: w337 -> [w904]
      tunnel: w619 -> [_]
      tunnel: w337 -> [_]
      tunnel: w619 -> [_]
      tunnel: w436 -> [w891]
      tunnel: [w891] -> w640
      tunnel: w505 -> [w890]
      tunnel: [w890] -> w639
      tunnel: w627 -> [w889]
      tunnel: [w889] -> w632
      tunnel: w629 -> [w888]
      tunnel: [w888] -> w628
      tunnel: [w885] -> w618
      tunnel: [w882] -> w617
      tunnel: [w879] -> w499
      tunnel: [w878] -> w498
      tunnel: [w875] -> w497
      tunnel: w406 -> [w872]
      tunnel: ["Save Data"] -> w405
      tunnel: [w865] -> w372
      tunnel: w640 -> [w1085]
      tunnel: w639 -> [w1084]
      tunnel: w632 -> [_]
      tunnel: w628 -> [_]
      tunnel: w618 -> [w1083]
      tunnel: w617 -> [w1082]
      tunnel: w499 -> [w1081]
      tunnel: w498 -> [w1080]
      tunnel: w497 -> [w1079]
      tunnel: w405 -> [w1078]
      tunnel: w404 -> [w1077]
      tunnel: w372 -> [w1075]
      frame #0 {
        w871 = 0.0
        # "1: old trap\n0: fleezers"
        # "Create files if saving data"
        n449 = local read "Save N sets"() -> (w874:bool)
        n450 = local read "Fixed X"() -> (w870:dbl)
        n451 = local read "Trap position (V)"() -> (w899:cluster{"X":dbl, "Y":dbl})
        n452 = local read "Fixed Y"() -> (w869:dbl)
        n453 = local read "Sampling Rate"() -> (w902:dbl)
        n454 = Or(x=w874, y="Save Data") -> (x .or. y?=w873:bool)
        n455 = Build Array(w873, "Save cal", w872) -> (w893:bool[])
        n456 = Compound Arithmetic op=OR("Save Data", "Save cal", w872) -> (w895:bool)
        n457 = Boolean Array To Number(Boolean array=w893) -> (number=w892:u32)
        n458 = Unbundle(w899) -> ("X"=w868:dbl, "Y"=w867:dbl)
        n459 = Build Array(w868, w867, w870, w869, w871, w871) -> (w898:dbl[])
        n460 = feedback #6(refnum<k0> refnum) -> (w864:refnum<file>)
        n461 = feedback #7(0) -> (w896:i32)
        n462 = feedback #8(refnum<k0> refnum) -> (w886:refnum<file>)
        n463 = feedback #9() -> (w880:dbl)  [unwired: 1 in]
        n464 = feedback #10(FALSE) -> (w876:bool)
        n465 = feedback #11(refnum<k0> refnum) -> (w883:refnum<file>)
        n466 = case shown="True" w895 {
          tunnel: w904 -> [_ _]
          tunnel: 9 -> [_ w950]
          tunnel: w902 -> [_ w949]
          tunnel: 6 -> [_ w948]
          tunnel: 5 -> [_ w947]
          tunnel: w898 -> [_ w946]
          tunnel: [w910 1] -> w879
          tunnel: w896 -> [w911 _]
          tunnel: w892 -> [_ w922]
          tunnel: [w909 w921] -> w885
          tunnel: w886 -> [w909 _]
          tunnel: [w908 w920] -> w882
          tunnel: w883 -> [w908 _]
          tunnel: 1.0 -> [_ w919]
          tunnel: [w907 w918] -> w878
          tunnel: w880 -> [w907 _]
          tunnel: [w906 w917] -> w875
          tunnel: w876 -> [w906 _]
          tunnel: [w905 w912] -> w865
          tunnel: w864 -> [w905 _]
          frame False {
            n467 = Increment(x=w911) -> (x+1=w910:i32)
          }
          frame True {
            w923 = FALSE ("Save Data")
            w928 = FALSE
            w929 = T20."big-endian, network order" ("byte order (0:big-endian, network order)")
            n468 = local write "Save cal"(w923) -> ()
            n469 = local write "Save Data"(w923) -> ()
            n470 = case shown="4" w922 {
              tunnel: w950 -> [w1025 w1043 w1074]
              tunnel: w949 -> [w1004 w1042 w1051]
              tunnel: w948 -> [w1024 w1040 w1070]
              tunnel: w947 -> [w1023 w1039 w1069]
              tunnel: w946 -> [w1022 w1036 w1066]
              tunnel: [w1021 w1035 w1055] -> w943
              tunnel: [w1002 w1026 w1046] -> w917
              tunnel: ["Averaging Number" 200 w1053] -> _
              tunnel: w919 -> [w1009 w1028 w1052]
              tunnel: [w1005 w1027 w1047] -> w918
              tunnel: [w1002 w1026 w1045] -> w914
              frame 1, Default {
                w1002 = TRUE
                w1010 = 0.0
                # "stage x,yz"
                # "Save N number/length of data. e.g. N =200 \nwill give only 200 long data points"
                # "Time trace"
                n471 = Boolean To (0,1)(Boolean=w1002) -> (0, 1=w1015:i16)
                n472 = local read "Averaging Number"() -> (w1020:i32)
                n473 = Increment(x=w1015) -> (x+1=w1014:i16)
                n474 = Divide(x=w1004, y=w1020) -> (x/y=w1019:dbl)
                n475 = To Double Precision Float(number=w1014) -> (double precision float=w1013:dbl)
                n476 = Reciprocal(x=w1019) -> (1/x=w1018:dbl)
                n477 = Reciprocal(x=w1004) -> (1/x=w1003:dbl)
                n478 = Build Array(w1025, w1003, w1018, w1024, w1023, 0 ("f")) -> (w1017:dbl[])
                n479 = Build Array(w1013, w1009, w1010, w1010, w1010) -> (w1016:dbl[])
                n480 = Build Array (concatenate)(w1017, w1022, w1016) -> (w1021:dbl[])
                n481 = Select(t="N sets", s="Save N sets", f=2147483647) -> (s? t:f=w1005:i32)
              }
              frame 2 {
                w1026 = FALSE
                w1031 = 0.0
                # "Calibration file"
                n482 = Reciprocal(x=w1042) -> (1/x=w1041:dbl)
                n483 = Boolean To (0,1)(Boolean=w1026) -> (0, 1=w1034:i16)
                n484 = To Double Precision Float(number=w1034) -> (double precision float=w1033:dbl)
                n485 = Build Array(w1043, w1041, w1041, w1040, w1039, 1) -> (w1037:dbl[])
                n486 = Build Array(w1033, w1028, w1031, w1031, w1031) -> (w1032:dbl[])
                n487 = Build Array (concatenate)(w1037, w1036, w1032) -> (w1035:dbl[])
                n488 = local read "Cal sets to save"() -> (w1027:i32)
                "Calibrating" <- TRUE ("Calibrating")
              }
              frame 4 {
                w1044 = FALSE ("Raster scan")
                w1062 = 0.0
                w1046 = TRUE
                # "Not using ncycles"
                # "FX curve"
                n489 = Not(x=w1046) -> (.not. x?=w1045:bool)
                n490 = local read "Averaging Number"() -> (w1073:i32)
                n491 = Boolean To (0,1)(Boolean=w1046) -> (0, 1=w1065:i16)
                n492 = local write "Saving Move"(w1044) -> ()
                n493 = Divide(x=w1051, y=w1073) -> (x/y=w1072:dbl)
                n494 = Increment(x=w1065) -> (x+1=w1064:i16)
                n495 = local write "Raster scan"(w1044) -> ()
                n496 = To Double Precision Float(number=w1064) -> (double precision float=w1063:dbl)
                n497 = Reciprocal(x=w1072) -> (1/x=w1071:dbl)
                n498 = Reciprocal(x=w1051) -> (1/x=w1050:dbl)
                n499 = Build Array(w1063, w1052, w1062, w1062, w1062) -> (w1061:dbl[])
                n500 = Build Array(w1074, w1050, w1071, w1070, w1069, 2) -> (w1067:dbl[])
                n501 = local read "Scan range (V)"() -> (w1048:dbl)
                n502 = local read "Pulling direction"() -> (w1059:bool)
                n503 = local read "Scan steps (mirror)"() -> (w1049:u64)
                n504 = local read "# scans"() -> (w1057:i32)
                n505 = local read "N sets to be saved"() -> (w1047:dbl)
                n506 = Not(x=w1059) -> (.not. x?=w1058:bool)
                n507 = local read "Averaging Number"() -> (w1053:i32)
                n508 = Boolean To (0,1)(Boolean=w1058) -> (0, 1=w1060:i16)
                n509 = Build Array(w1060, w1048, w1049, 0, w1057) -> (w1056:dbl[])
                n510 = Build Array (concatenate)(w1067, w1066, w1061, w1056) -> (w1055:dbl[])
              }
            }
            n511 = call "CreateSaveFile.vi"("Index In"="Save file index", "Ext"=".dat", "Insert"="", "Directory"="Path") -> ("Index Out"=w916:i32, "Path Out"=w913:path)  [unwired: 6 in]
            "Current file name" <- w913
            n512 = case shown="True" w914 {
              tunnel: w913 -> [_ w962]
              tunnel: [refnum<k0> refnum w959] -> w912
              frame False {
              }
              frame True {
                # "SY 190201 \nAdding functionality to get time points of start and stop moves. \nWehn timetrace save data starts save time point"
                n513 = Path To String(path=w962) -> (string=w966:string)
                n514 = Get Date/Time In Seconds() -> (seconds since 1Jan1904=w976:timestamp)
                n515 = String Length(string=w966) -> (length=w963:i32)
                n516 = Subtract(x=w963, y=4) -> (x-y=w965:i32)
                n517 = Format Date/Time String(time format string (%c)="%H:%M:%S%3u", seconds (now)=w976, UTC format=TRUE) -> (date/time string=w960:string)
                n518 = call <vilib>:"Space Constant.vi"() -> ("String"=w954:string)
                n519 = String Subset(string=w966, length (rest)=w965) -> (substring=w967:string)  [unwired: 1 in]
                n520 = Concatenate Strings(w967, "_stagetime.txt" ("string")) -> (w969:string)
                n521 = String To Path(string=w969) -> (path=w970:path)
                n522 = Open/Create/Replace File(file path (use dialog)=w970, operation (0:open)=T19."create", access (0:read/write)=enum16{"read/write", "read-only", "write-only"}."write-only") -> (refnum out=w974:refnum<file>, error out=w973:errorcluster)  [unwired: 3 in, 1 out]
                n523 = Deny Access(4:w973, 7:w974) -> (3:w975:refnum<file>)  [unwired: 1 in, 1 out]
                n524 = Concatenate Strings(w960, w954, "start", "\r\n") -> (w961:string)
                n525 = Write to Text File(file (use dialog)=w975, text=w961) -> (refnum out=w959:refnum<file>)  [unwired: 2 in, 2 out]
                n526 = local write "Move time"(w960) -> ()
                n527 = local read "Raster scanning..."() -> (w957:bool)
                n528 = local read "Calibrating"() -> (w958:bool)
                n529 = Or(x=w958, y=w957) -> (x .or. y?=w956:bool)
                n530 = Not(x=w956) -> (.not. x?=w955:bool)
                n531 = local write "Saving Move"(w955) -> ()
              }
            }
            n532 = Open/Create/Replace File(file path (use dialog)=w913, operation (0:open)=T19."create", access (0:read/write)=enum16{"read/write", "read-only", "write-only"}."write-only") -> (refnum out=w936:refnum<file>, error out=w937:errorcluster)  [unwired: 3 in, 1 out]
            n533 = local write "Save file index"(w916) -> ()
            n534 = Array Size(array=w943) -> (size(s)=w945:i32)
            n535 = case shown="True" w917 {
              tunnel: w913 -> [_ w1001]
              tunnel: [refnum<k0> refnum w980] -> w920
              frame False {
              }
              frame True {
                w987 = 0.0
                n536 = Path To String(path=w1001) -> (string=w997:string)
                n537 = Build Array(w987, w987, w987, w987, w987, w987, w987, w987) -> (w984:dbl[])
                n538 = String Length(string=w997) -> (length=w1000:i32)
                n539 = Array Size(array=w984) -> (size(s)=w986:i32)
                n540 = Subtract(x=w1000, y=4) -> (x-y=w998:i32)
                n541 = To Double Precision Float(number=w986) -> (double precision float=w985:dbl)
                n542 = String Subset(string=w997, length (rest)=w998) -> (substring=w996:string)  [unwired: 1 in]
                n543 = Build Array (concatenate)(w985, w984) -> (w983:dbl[])
                n544 = Concatenate Strings(w996, "_pos.dat" ("string")) -> (w994:string)
                n545 = String To Path(string=w994) -> (path=w993:path)
                n546 = Open/Create/Replace File(file path (use dialog)=w993, operation (0:open)=T19."create", access (0:read/write)=enum16{"read/write", "read-only", "write-only"}."write-only") -> (refnum out=w989:refnum<file>, error out=w990:errorcluster)  [unwired: 3 in, 1 out]
                n547 = Deny Access(4:w990, 7:w989) -> (3:w988:refnum<file>)  [unwired: 1 in, 1 out]
                n548 = Write to Binary File(file (use dialog)=w988, data=w983, 5:FALSE ("prepend array or string size? (T)"), 9:T20."big-endian, network order" ("byte order (0:big-endian, network order)")) -> (refnum out=w980:refnum<file>)  [unwired: 2 in, 2 out]
              }
            }
            n549 = Deny Access(4:w937, 7:w936) -> (0:w927:errorcluster, 3:w935:refnum<file>)  [unwired: 1 in]
            n550 = String Length(string="Comment") -> (length=w942:i32)
            n551 = To Double Precision Float(number=w945) -> (double precision float=w944:dbl)
            n552 = To Double Precision Float(number=w942) -> (double precision float=w941:dbl)
            n553 = Build Array (concatenate)(w944, w943, w941) -> (w932:dbl[])
            n554 = Write to Binary File(file (use dialog)=w935, data=w932, error in=w927, 5:w928, 9:w929) -> (refnum out=w931:refnum<file>, error out=w926:errorcluster)  [unwired: 1 in, 1 out]
            n555 = Write to Binary File(file (use dialog)=w931, data="Comment", error in=w926, 5:w928, 9:w929) -> (refnum out=w921:refnum<file>)  [unwired: 1 in, 2 out]
            "Saving" <- TRUE
          }
        }
        n556 = feedback-in #6(w865) -> ()
        n557 = feedback-in #7(w879) -> ()
        n558 = feedback-in #8(w885) -> ()
        n559 = feedback-in #9(w878) -> ()
        n560 = feedback-in #10(w875) -> ()
        n561 = feedback-in #11(w882) -> ()
      }
      frame #1 {
        n562 = local read "Saving"() -> (w1076:bool)
        n563 = case shown="True" w1076 {
          tunnel: w1085 -> [_ w1105]
          tunnel: w1084 -> [_ w1104]
          tunnel: w1083 -> [_ w1103]
          tunnel: w1082 -> [_ w1102]
          tunnel: w1081 -> [_ w1093]
          tunnel: w1080 -> [_ w1094]
          tunnel: w1079 -> [_ w1097]
          tunnel: w1078 -> [_ w1089]
          tunnel: w1077 -> [_ w1088]
          tunnel: w1075 -> [_ w1086]
          frame False {
            (unwired) FALSE ("Calibrating")
          }
          frame True {
            n564 = local read "Stop"() -> (w1100:bool)
            n565 = Less Or Equal?(x=w1093, y=w1094) -> (x <= y?=w1101:bool)
            n566 = Divide(x=w1093, y=w1094) -> (x/y=w1092:dbl)
            n567 = Or(x=w1100, y="Stop saving") -> (x .or. y?=w1087:bool)
            n568 = Multiply(x=100.0, y=w1092) -> (x*y=w1091:dbl)
            n569 = Not(x=w1087) -> (.not. x?=w1099:bool)
            n570 = And(x=w1101, y=w1099) -> (x .and. y?=w1098:bool)
            n571 = case shown="False" w1098 {
              tunnel: w1103 -> [w1110 w1135]
              tunnel: w1104 -> [_ w1134]
              tunnel: w1105 -> [_ w1133]
              tunnel: w1102 -> [w1109 w1132]
              tunnel: w1097 -> [w1106 _]
              tunnel: [0.0 ("Progress") w1131] -> w1096
              tunnel: w1091 -> [_ w1131]
              tunnel: w1089 -> [_ _]
              tunnel: w1088 -> [_ w1130]
              tunnel: w1086 -> [w1107 w1127]
              frame False {
                n572 = flat-sequence {
                  tunnel: w1110 -> [w1115]
                  tunnel: w1109 -> [w1114]
                  tunnel: w1107 -> [w1113]
                  tunnel: w1106 -> [w1112]
                  frame #0 {
                    n573 = local read "Saving Move"() -> (w1111:bool)
                    n574 = case shown="True" w1112 {
                      tunnel: w1114 -> [_ w1125]
                      frame False {
                      }
                      frame True {
                        n575 = Close File(refnum=w1125) -> ()  [unwired: 1 in, 2 out]
                      }
                    }
                    n576 = case shown="True" w1111 {
                      tunnel: w1113 -> [_ w1120]
                      frame False {
                      }
                      frame True {
                        n577 = Get Date/Time In Seconds() -> (seconds since 1Jan1904=w1124:timestamp)
                        n578 = call <vilib>:"Space Constant.vi"() -> ("String"=w1119:string)
                        n579 = Format Date/Time String(time format string (%c)="%H:%M:%S%3u", seconds (now)=w1124, UTC format=TRUE) -> (date/time string=w1117:string)
                        n580 = Concatenate Strings(w1117, w1119, "end") -> (w1116:string)
                        n581 = Write to Text File(file (use dialog)=w1120, text=w1116) -> (refnum out=w1121:refnum<file>)  [unwired: 2 in, 2 out]
                        n582 = Close File(refnum=w1121) -> ()  [unwired: 1 in, 2 out]
                        n583 = local write "Move time"(w1117) -> ()
                      }
                    }
                    n584 = Close File(refnum=w1115) -> ()  [unwired: 1 in, 2 out]
                  }
                  frame #1 {
                    w1126 = FALSE
                    n585 = local write "Saving"(w1126) -> ()
                    n586 = local write "Stop saving"(w1126) -> ()
                    n587 = local write "Saving Move"(w1126) -> ()
                    n588 = local write "Calibrating"(w1126) -> ()
                    n589 = call <vilib>:"Beep.vi"() -> ()  [unwired: 12 in]
                  }
                }
              }
              frame True {
                n590 = local read "Calibrating"() -> (w1129:bool)
                n591 = local read "Saving Move"() -> (w1128:bool)
                n592 = case shown="False" w1129 {
                  tunnel: w1135 -> [w1168 w1184]
                  tunnel: w1134 -> [_ w1183]
                  tunnel: w1133 -> [w1155 w1177]
                  tunnel: w1132 -> [w1154 _]
                  tunnel: w1130 -> [w1146 _]
                  frame False {
                    n593 = local read "Averaging Number"() -> (w1162:i32)
                    n594 = Array Subset(array=w1155, index (row)=0 ("index"), length (row)=6 ("length")) -> (w1151:dbl[][])  [unwired: 2 in]
                    n595 = Array Subset(array=w1155, index (row)=6 ("index"), length (row)=2 ("length")) -> (w1150:dbl[][])  [unwired: 2 in]
                    n596 = Array Size(array=w1150) -> (size(s)=w1161:i32[])
                    n597 = Array Size(array=w1151) -> (size(s)=w1158:i32[])
                    n598 = Index Array(array=w1146, index=0) -> (element=w1143:waveform(dbl))
                    n599 = Index Array(array=w1146, index=1) -> (element=w1142:waveform(dbl))
                    n600 = for {
                      tunnel: w1151 -> [w1172] mode=indexing
                      tunnel: w1162 -> [w1174]
                      tunnel: [w1173] -> w1149 mode=indexing
                      n601 = call "Downsample 1D array.vi"("Ave N"=w1174, "Arrray In"=w1172) -> ("Array Out"=w1173:dbl[])  [unwired: 9 in]
                    }
                    n602 = Unbundle By Name(w1143) -> ()  [unwired: 1 out]
                    n603 = Unbundle By Name(w1142) -> ()  [unwired: 1 out]
                    n604 = Multiply Array Elements(1:w1158) -> (0:w1157:i32)
                    n605 = for {
                      tunnel: w1150 -> [w1171] mode=indexing
                      tunnel: w1162 -> [w1170]
                      tunnel: [w1169] -> w1153 mode=indexing
                      n606 = call "Downsample 1D array.vi"("Ave N"=w1170, "Arrray In"=w1171) -> ("Array Out"=w1169:dbl[])  [unwired: 9 in]
                    }
                    n607 = Multiply Array Elements(1:w1161) -> (0:w1160:i32)
                    n608 = Divide(x=w1157, y=w1162) -> (x/y=w1163:dbl)
                    n609 = Divide(x=w1160, y=w1162) -> (x/y=w1159:dbl)
                    n610 = Transpose 2D Array(2D array=w1149) -> (transposed array=w1148:dbl[][])
                    n611 = Transpose 2D Array(2D array=w1153) -> (transposed array=w1147:dbl[][])
                    n612 = Reshape Array(w1148, w1163) -> (w1152:dbl[])
                    n613 = Reshape Array(w1147, w1159) -> (w1156:dbl[])
                    n614 = call <vilib>:"Write File+ [SGL].vi"("1D array"=w1156, "refnum"=w1154) -> ()  [unwired: 7 in, 3 out]
                    n615 = call <vilib>:"Write File+ [SGL].vi"("1D array"=w1152, "refnum"=w1168) -> ()  [unwired: 7 in, 3 out]
                  }
                  frame True {
                    n616 = Array Subset(array=w1177, index (row)=0 ("index"), length (row)=6 ("length")) -> (w1175:dbl[][])  [unwired: 2 in]
                    n617 = Transpose 2D Array(2D array=w1175) -> (transposed array=w1181:dbl[][])
                    n618 = Array Size(array=w1175) -> (size(s)=w1176:i32[])
                    n619 = Multiply Array Elements(1:w1176) -> (0:w1182:i32)
                    n620 = Reshape Array(w1181, w1182) -> (w1180:dbl[])
                    n621 = call <vilib>:"Write File+ [SGL].vi"("1D array"=w1180, "error in (no error)"=w1183, "refnum"=w1184) -> ()  [unwired: 6 in, 3 out]
                  }
                }
                n622 = case shown="True" w1128 {
                  tunnel: w1127 -> [_ w1136]
                  frame False {
                  }
                  frame True {
                    n623 = event shown="[0] \"Move time\": Value Change" {
                      selector: _ -> [_ _]
                      dyn-events: _ -> [_ _]
                      timeout: 1 -> [_ _]
                      tunnel: w1136 -> [w1141 _]
                      event "Move time": Value Change {
                        n624 = event-data() -> ("NewVal"=w1140:string)  [unwired: 1 in, 5 out]
                        n625 = Concatenate Strings(w1140, "\r\n") -> (w1138:string)
                        n626 = Write to Text File(file (use dialog)=w1141, text=w1138) -> ()  [unwired: 2 in, 3 out]
                      }
                      event Timeout {
                        n627 = event-data() -> ()  [unwired: 1 in, 3 out]
                      }
                    }
                  }
                }
              }
            }
            "Progress" <- w1096
          }
        }
      }
    }
    n628 = Square Root(x=w476) -> (sqrt(x)=→"Force noise (pN)":dbl)
    n629 = local read "Flushing Sample"() -> (w408:bool)
    n630 = case shown="True" w408 {
      frame False {
      }
      frame True {
        n631 = local read "Flush Sample Start Time"() -> (w819:u32)
        n632 = local read "Sample flush time (s)"() -> (w812:dbl)
        n633 = Tick Count (ms)() -> (millisecond timer value=w820:u32)
        n634 = Subtract(x=w820, y=w819) -> (x-y=w810:u32)
        n635 = Multiply(x=u32 1000, y=w812) -> (x*y=w811:dbl)
        n636 = Divide(x=w810, y=w811) -> (x/y=w815:dbl)
        n637 = Greater?(x=w810, y=w811) -> (0:w818:bool)
        n638 = Not(x=w818) -> (.not. x?=w817:bool)
        n639 = Boolean To (0,1)(Boolean=w817) -> (0, 1=w816:i16)
        n640 = Compound Arithmetic op=MULTIPLY(w816, w815, 100.0 ("value")) -> (→"Sample Flush Meter":dbl)
        n641 = case shown="True" w818 {
          frame False {
          }
          frame True {
            w822 = FALSE ("Inject Sample")
            n642 = property on="Clear Volume" class="Bool (strict)"("Val(Sgnl)"=TRUE ("Value (Signaling)")) -> ()  [unwired: 2 in, 2 out]
            n643 = local write "Inject Sample"(w822) -> ()
            n644 = local write "Flushing Sample"(w822) -> ()
          }
        }
      }
    }
    n645 = feedback #12(0) -> (w392:i32)
    n646 = feedback #13(0) -> (w389:i32)
    n647 = feedback #14(0) -> (w394:i32)
    n648 = case shown="True" w399 {
      tunnel: w403 -> [w711 w769]
      tunnel: [w711 w753] -> w402
      tunnel: w401 -> [w710 w768]
      tunnel: [w710 w752] -> w400
      tunnel: "Raster scan" -> [w709 w746]
      tunnel: [w709 w745] -> w397
      tunnel: [0 w744] -> w395
      tunnel: w394 -> [_ w738]
      tunnel: w392 -> [_ w726]
      tunnel: [0 w729] -> w391
      tunnel: w389 -> [_ w735]
      tunnel: [0 w734] -> w388
      frame False {
      }
      frame True {
        # "Reset step counter"
        # "Current position"
        # "Initial values"
        n649 = local read "Conv Y (nm/V)"() -> (w721:dbl)
        n650 = local read "Conv X (nm/V)"() -> (w722:dbl)
        n651 = local read "Trap delta (nm)"() -> (w720:dbl)
        n652 = disable-structure shown="Disabled" {
          frame Disabled {
            n653 = local write "Raster scan"(FALSE ("Raster scan")) -> ()
            n654 = property on="Reset data stream" class="Bool (strict)"("Val(Sgnl)"=TRUE) -> ()  [unwired: 2 in, 2 out]
          }
          frame Enabled {
          }
        }
        n655 = local read "Data update period (s/set)"() -> (w743:dbl)
        n656 = local read "Time per step (ms)"() -> (w740:dbl)
        n657 = Select(t=w721, s="Pulling direction", f=w722) -> (s? t:f=w719:dbl)
        n658 = Divide(x=w720, y=w719) -> (x/y=w718:dbl)
        n659 = local read "Fixed X"() -> (w762:dbl)
        n660 = local read "Fixed Y"() -> (w763:dbl)
        n661 = local read "Fixed X"() -> (w724:dbl)
        n662 = local read "Fixed Y"() -> (w723:dbl)
        n663 = local read "Trap position (V)"() -> (w725:cluster{"X":dbl, "Y":dbl})
        n664 = Select(t=w723, s="Pulling direction", f=w724) -> (s? t:f=w717:dbl)
        n665 = local read "Scan steps (mirror)"() -> (w751:u64)
        n666 = Unbundle(w725) -> ("X"=w715:dbl, "Y"=w716:dbl)
        n667 = Multiply(x=w743, y=1000.0) -> (x*y=w741:dbl)
        n668 = local read "Stop raster"() -> (w758:bool)
        n669 = local read "Stop saving"() -> (w759:bool)
        n670 = Select(t=w762, s="Pulling direction", f=w763) -> (s? t:f=w770:dbl)
        n671 = Add(x=w718, y=w717) -> ()  [unwired: 1 out]
        n672 = local write "Saving Move"(FALSE) -> ()
        n673 = Divide(x=w740, y=w741) -> (x/y=w739:dbl)
        n674 = Quotient & Remainder(x=w738, y=w739) -> (x-y*floor(x/y)=w737:dbl)  [unwired: 1 out]
        n675 = Not(x=w758) -> (.not. x?=w757:bool)
        n676 = Select(t=w716, s="Pulling direction", f=w715) -> (s? t:f=w713:dbl)
        n677 = Not(x=w759) -> (.not. x?=w756:bool)
        n678 = Multiply(x=u64 2, y=w751) -> (x*y=w747:u64)
        n679 = Equal To 0?(x=w737) -> (x = 0?=w736:bool)
        n680 = Less?(x=w726, y=w747) -> (x < y?=w748:bool)
        n681 = Compound Arithmetic op=AND(w748, w757, w756, w736) -> (w749:bool)
        n682 = Not(x=w748) -> (.not. x?=w732:bool)
        n683 = feedback #15() -> (w754:dbl)  [unwired: 1 in]
        n684 = case shown="True" w749 {
          tunnel: w770 -> [_ w805]
          tunnel: w713 -> [_ w787]
          tunnel: w769 -> [w782 w804]
          tunnel: w768 -> [w781 w803]
          tunnel: [w782 w802] -> w753
          tunnel: [w781 w801] -> w752
          tunnel: [w778 w790] -> w755
          tunnel: w726 -> [w779 w785]
          tunnel: w754 -> [w778 w784]
          tunnel: w746 -> [w780 w789]
          tunnel: [w780 w789] -> w745
          tunnel: [w779 w788] -> w730
          frame False {
          }
          frame True {
            # "Go forward or backward?"
            n685 = local read "Scan increment (V)"() -> (w783:dbl)
            n686 = local read "Scan steps (mirror)"() -> (w794:u64)
            n687 = Multiply(x=w783, y=w785) -> (x*y=w786:dbl)
            n688 = Less?(x=w785, y=w794) -> (x < y?=w793:bool)
            n689 = Add(x=w787, y=w786) -> (x+y=w796:dbl)
            n690 = Subtract(x=w784, y=w783) -> (x-y=w795:dbl)
            n691 = Select(t=w796, s=w793, f=w795) -> (s? t:f=w790:dbl)
            n692 = local read "Pulling direction"() -> (w792:bool)
            n693 = Build Array(w790, w805) -> (w799:dbl[])
            n694 = Build Array(w805, w790) -> (w798:dbl[])
            n695 = Select(t=w799, s=w792, f=w798) -> (s? t:f=w797:dbl[])
            n696 = call-poly <vilib>:"DAQmx Write.vi"("task/channels in"=w804, "auto start"=TRUE, "data"=w797, "error in"=w803) -> ("task out"=w802:refnum<k21>, "error out"=w801:errorcluster)  [unwired: 9 in, 1 out]
            n697 = Increment(x=w785) -> (x+1=w788:i32)
            "Raster scanning..." <- TRUE ("Raster scanning...")
          }
        }
        n698 = feedback-in #15(w755) -> ()
        n699 = case shown="True" w732 {
          tunnel: w735 -> [w775 w777]
          tunnel: [w775 w776] -> w734
          frame False {
          }
          frame True {
            n700 = Increment(x=w777) -> (x+1=w776:i32)
          }
        }
        n701 = local read "# scans"() -> (w733:i32)
        n702 = local read "Stop saving"() -> (w761:bool)
        n703 = Greater Or Equal?(x=w734, y=w733) -> (x >= y?=w727:bool)
        n704 = Not(x=w727) -> (.not. x?=w728:bool)
        n705 = And(x=w732, y=w728) -> (x .and. y?=w731:bool)
        n706 = Compound Arithmetic op=OR(w727, "Stop raster", w761) -> (w764:bool)
        n707 = case shown="True" w764 {
          frame False {
          }
          frame True {
            n708 = flat-sequence {
              frame #0 {
                n709 = Wait (ms)(milliseconds to wait=u32 300) -> ()  [unwired: 1 out]
              }
              frame #1 {
                n710 = property on="Trap delta (nm)" class="DigNum (strict)"("Val(Sgnl)"="Trap delta\nafter (nm)") -> ()  [unwired: 2 in, 2 out]
              }
            }
          }
        }
        n711 = And(x="Flow on\nafter raster?", y=w764) -> (x .and. y?=w765:bool)
        n712 = case shown="True" w765 {
          frame False {
          }
          frame True {
            n713 = property on="Inject Sample" class="Bool (strict)"("Val(Sgnl)"=TRUE ("Value (Signaling)")) -> ()  [unwired: 2 in, 2 out]
          }
        }
        n714 = case shown="True" w731 {
          tunnel: w730 -> [w773 _]
          tunnel: [w773 0] -> w729
          frame False {
          }
          frame True {
          }
        }
        n715 = Not(x=w764) -> (.not. x?=w767:bool)
        n716 = local write "Raster scanning..."(w767) -> ()
        n717 = Increment(x=w738) -> (x+1=w744:i32)
      }
    }
    n718 = And(x="Save scans", y=w397) -> (x .and. y?=w406:bool)
    n719 = feedback-in #12(w391) -> ()
    n720 = feedback-in #13(w388) -> ()
    n721 = feedback-in #14(w395) -> ()
    n722 = local read "Stop"() -> (w684:bool)
  }
  n723 = local write "Progress"(u8 0 ("Progress")) -> ()
  n724 = local write "Calibrating"(FALSE ("Calibrating")) -> ()
  n725 = VISA Open(VISA resource name="USB port") -> (VISA resource name=w12:refnum<visa-resource-name>, error out=w11:errorcluster)  [unwired: 1 in, 3 out]
  n726 = VISA Enable Event(8:w11, 10:w10, 11:w12) -> (0:w7:errorcluster, 3:w8:refnum<visa-resource-name>)  [unwired: 1 out]
  n727 = call-poly "VISA Configure Serial Port"("VISA resource name"=refnum<visa-resource-name> "COM5", "baud rate (9600)"=u32 19200) -> ("VISA resource name out"=w2:refnum<visa-resource-name>, "error out"=w28:errorcluster)  [unwired: 12 in]
  n728 = while {
    tunnel: w2 -> [w1269]
    shift-right: [w1265] -> w4
    shift-left: w8 -> [w1268]
    shift-right: [w1266] -> w3
    shift-left: w7 -> [w1267]
    stop <- w1264 stop-if-true
    n729 = global read "FAST_Global_var.vi" "FAST L"() -> (→"FAST Z" →"FAST Z":bool)
    n730 = global read "FAST_Global_var.vi" "FAST R"() -> (→"FAST X-Y" →"FAST X-Y":bool)
    n731 = call "LogitechSubVi.vi"("USB port"=w1268, "VISA resource name in 2 (for the Newport)"=w1269, "error in (no error)"=w1267, "X-Y Wait time"="X-Y Wait time", "Z Wait time"="Z Wait time", "XY Speed Definitions"="XY Speed Definitions", "Z Speed Definitions"="Z Speed Definitions") -> ("Right stick button"=→"Right stick button":bool, "Left stick button"=→"Left stick button":bool, "USB port out"=w1265:refnum<visa-resource-name>, "error out"=w1266:errorcluster, "A B X Y"=w1258:cluster{"A":bool, "B":bool, "X":bool, "Y":bool}, "LB RB"=w1257:T22, "U D L R"=w1263:cluster{"U":bool, "D":bool, "L":bool, "R":bool}, "Sticks"=w1256:T23)  [unwired: 5 in]
    n732 = Unbundle By Name(w1257) -> ("LB"=w1251:bool, "RB"=w1250:bool, "BACK"=w1224:bool, "Logitech"=w1223:bool, "START"=w1225:bool)
    "RB" <- w1250
    "LB" <- w1251
    "BACK" <- w1224
    "START" <- w1225
    "Logitech" <- w1223
    n733 = case shown="True" w1225 {
      selector: w1225 -> [_ w1273]
      frame False {
      }
      frame True {
        n734 = property on="Move to Position 2" class="Bool (strict)"("Val(Sgnl)"=w1273) -> ()  [unwired: 2 in, 2 out]
      }
    }
    n735 = case shown="True" w1223 {
      frame False {
      }
      frame True {
        n736 = local read "Inject Sample"() -> (w1270:bool)
        n737 = Not(x=w1270) -> (.not. x?=w1271:bool)
        n738 = property on="Inject Sample" class="Bool (strict)"("Val(Sgnl)"=w1271) -> ()  [unwired: 2 in, 2 out]
      }
    }
    n739 = case shown="True" w1251 {
      frame False {
      }
      frame True {
        n740 = local read "Shutter 1 (B)"() -> (w1317:bool)
        n741 = Not(x=w1317) -> (.not. x?=w1316:bool)
        n742 = property on="Shutter 1 (B)" class="Bool (strict)"("Val(Sgnl)"=w1316) -> ()  [unwired: 2 in, 2 out]
      }
    }
    n743 = case shown="True" w1224 {
      selector: w1224 -> [_ w1272]
      frame False {
      }
      frame True {
        n744 = property on="Move to Position 1" class="Bool (strict)"("Val(Sgnl)"=w1272) -> ()  [unwired: 2 in, 2 out]
      }
    }
    n745 = Unbundle By Name(w1263) -> ("U"=→"U":bool, "D"=→"D":bool, "L"=→"L":bool, "R"=→"R":bool)
    n746 = Unbundle By Name(w1258) -> ("A"=w1246:bool, "B"=w1244:bool, "X"=w1249:bool, "Y"=w1242:bool)
    "A" <- w1246
    "B" <- w1244
    "X" <- w1249
    "Y" <- w1242
    n747 = case shown="\"Fish\"" "A command" {
      tunnel: w1246 -> [w1296 w1298 w1300 w1303]
      frame "Got ADig", Default {
        n748 = case shown="True" w1296 {
          selector: w1296 -> [_ w1297]
          frame False {
          }
          frame True {
            n749 = property on="Got ADig bead" class="Bool (strict)"("Val(Sgnl)"=w1297) -> ()  [unwired: 2 in, 2 out]
          }
        }
      }
      frame "Dump" {
        n750 = case shown="True" w1298 {
          selector: w1298 -> [_ w1299]
          frame False {
          }
          frame True {
            n751 = property on="Dump beads" class="Bool (strict)"("Val(Sgnl)"=w1299) -> ()  [unwired: 2 in, 2 out]
          }
        }
      }
      frame "Fish" {
        n752 = case shown="True" w1300 {
          frame False {
          }
          frame True {
            n753 = local read "Fish"() -> (w1301:bool)
            n754 = Not(x=w1301) -> (.not. x?=w1302:bool)
            n755 = property on="Fish" class="Bool (strict)"("Val(Sgnl)"=w1302) -> ()  [unwired: 2 in, 2 out]
          }
        }
      }
      frame "Got DNA" {
        n756 = case shown="True" w1303 {
          selector: w1303 -> [_ w1304]
          frame False {
          }
          frame True {
            n757 = property on="Got DNA bead" class="Bool (strict)"("Val(Sgnl)"=w1304) -> ()  [unwired: 2 in, 2 out]
          }
        }
      }
    }
    n758 = case shown="True" w1250 {
      frame False {
      }
      frame True {
        n759 = local read "Shutter 2 (A)"() -> (w1315:bool)
        n760 = Not(x=w1315) -> (.not. x?=w1314:bool)
        n761 = property on="Shutter 2 (A)" class="Bool (strict)"("Val(Sgnl)"=w1314) -> ()  [unwired: 2 in, 2 out]
      }
    }
    n762 = Unbundle By Name(w1256) -> ("Right X"=w1228:i8, "Right Y"=w1230:i8, "Left X"=w1232:i8, "Left Y"=w1237:i8)
    n763 = Not Equal?(x=w1237, y=i8 0) -> (x != y?=w1238:bool)
    n764 = case shown="True" w1238 {
      tunnel: w1237 -> [_ w1277]
      frame False {
      }
      frame True {
        "Left Y" <- w1277
      }
    }
    n765 = case shown="\"Got DNA\", Default" "B command" {
      tunnel: w1244 -> [w1287 w1289 w1291 w1293]
      frame "Got DNA", Default {
        n766 = case shown="True" w1287 {
          selector: w1287 -> [_ w1288]
          frame False {
          }
          frame True {
            n767 = property on="Got DNA bead" class="Bool (strict)"("Val(Sgnl)"=w1288) -> ()  [unwired: 2 in, 2 out]
          }
        }
      }
      frame "Got ADig" {
        n768 = case shown="True" w1289 {
          selector: w1289 -> [_ w1290]
          frame False {
          }
          frame True {
            n769 = property on="Got ADig bead" class="Bool (strict)"("Val(Sgnl)"=w1290) -> ()  [unwired: 2 in, 2 out]
          }
        }
      }
      frame "Dump" {
        n770 = case shown="True" w1291 {
          selector: w1291 -> [_ w1292]
          frame False {
          }
          frame True {
            n771 = property on="Dump beads" class="Bool (strict)"("Val(Sgnl)"=w1292) -> ()  [unwired: 2 in, 2 out]
          }
        }
      }
      frame "Fish" {
        n772 = case shown="True" w1293 {
          frame False {
          }
          frame True {
            n773 = local read "Fish"() -> (w1294:bool)
            n774 = Not(x=w1294) -> (.not. x?=w1295:bool)
            n775 = property on="Fish" class="Bool (strict)"("Val(Sgnl)"=w1295) -> ()  [unwired: 2 in, 2 out]
          }
        }
      }
    }
    n776 = Not Equal?(x=w1228, y=i8 0) -> (x != y?=w1229:bool)
    n777 = Not Equal?(x=w1230, y=i8 0) -> (x != y?=w1231:bool)
    n778 = Not Equal?(x=w1232, y=i8 0) -> (x != y?=w1233:bool)
    n779 = case shown="True" w1233 {
      tunnel: w1232 -> [_ w1276]
      frame False {
      }
      frame True {
        "Left X" <- w1276
      }
    }
    n780 = case shown="False" w1229 {
      tunnel: w1228 -> [_ w1274]
      frame False {
      }
      frame True {
        "Right X" <- w1274
      }
    }
    n781 = case shown="False" w1231 {
      tunnel: w1230 -> [_ w1275]
      frame False {
      }
      frame True {
        "Right Y" <- w1275
      }
    }
    n782 = case shown="\"Dump\", Default" "X command" {
      tunnel: w1249 -> [w1305 w1307 w1310 w1312]
      frame "Dump", Default {
        n783 = case shown="True" w1305 {
          selector: w1305 -> [_ w1306]
          frame False {
          }
          frame True {
            n784 = property on="Dump beads" class="Bool (strict)"("Val(Sgnl)"=w1306) -> ()  [unwired: 2 in, 2 out]
          }
        }
      }
      frame "Fish" {
        n785 = case shown="True" w1307 {
          frame False {
          }
          frame True {
            n786 = local read "Fish"() -> (w1309:bool)
            n787 = Not(x=w1309) -> (.not. x?=w1308:bool)
            n788 = property on="Fish" class="Bool (strict)"("Val(Sgnl)"=w1308) -> ()  [unwired: 2 in, 2 out]
          }
        }
      }
      frame "Got ADig" {
        n789 = case shown="True" w1310 {
          selector: w1310 -> [_ w1311]
          frame False {
          }
          frame True {
            n790 = property on="Got ADig bead" class="Bool (strict)"("Val(Sgnl)"=w1311) -> ()  [unwired: 2 in, 2 out]
          }
        }
      }
      frame "Got DNA" {
        n791 = case shown="True" w1312 {
          selector: w1312 -> [_ w1313]
          frame False {
          }
          frame True {
            n792 = property on="Got DNA bead" class="Bool (strict)"("Val(Sgnl)"=w1313) -> ()  [unwired: 2 in, 2 out]
          }
        }
      }
    }
    n793 = case shown="\"Fish\", Default" "Y command" {
      tunnel: w1242 -> [w1278 w1281 w1283 w1285]
      frame "Fish", Default {
        n794 = case shown="True" w1278 {
          frame False {
          }
          frame True {
            n795 = local read "Fish"() -> (w1279:bool)
            n796 = Not(x=w1279) -> (.not. x?=w1280:bool)
            n797 = property on="Fish" class="Bool (strict)"("Val(Sgnl)"=w1280) -> ()  [unwired: 2 in, 2 out]
          }
        }
      }
      frame "Dump" {
        n798 = case shown="True" w1281 {
          selector: w1281 -> [_ w1282]
          frame False {
          }
          frame True {
            n799 = property on="Dump beads" class="Bool (strict)"("Val(Sgnl)"=w1282) -> ()  [unwired: 2 in, 2 out]
          }
        }
      }
      frame "Got ADig" {
        n800 = case shown="True" w1283 {
          selector: w1283 -> [_ w1284]
          frame False {
          }
          frame True {
            n801 = property on="Got ADig bead" class="Bool (strict)"("Val(Sgnl)"=w1284) -> ()  [unwired: 2 in, 2 out]
          }
        }
      }
      frame "Got DNA" {
        n802 = case shown="True" w1285 {
          selector: w1285 -> [_ w1286]
          frame False {
          }
          frame True {
            n803 = property on="Got DNA bead" class="Bool (strict)"("Val(Sgnl)"=w1286) -> ()  [unwired: 2 in, 2 out]
          }
        }
      }
    }
    n804 = local read "Stop"() -> (w1264:bool)
  }
  n805 = VISA Close(VISA resource name=w4, error in (no error)=w3) -> (error out=w5:errorcluster)
  n806 = call <vilib>:"Simple Error Handler.vi"("error in (no error)"=w5) -> ()  [unwired: 1 in, 8 out]
  n807 = node-c288(i64 100 ("Period"), 2 ("Processor")) -> (w30:T14)  [unwired: 2 in]
  n808 = timed-loop {
    timing: w30 -> [_]
    timing-out: [_] -> w29
    tunnel: w2 -> [w1318]
    tunnel: w28 -> [w1320]
    tunnel: [w1318] -> w27
    stop <- w1319 stop-if-true
    n809 = node-c288() -> ()  [unwired: 1 in, 1 out]
    n810 = event shown="[10] \"Force FB script\": Value Change" {
      selector: _ -> [_ _ _ _ _ _ _ _ _ _ _ _ _ _ _ _]
      dyn-events: _ -> [_ _ _ _ _ _ _ _ _ _ _ _ _ _ _ _]
      timeout: _ -> [_ _ _ _ _ _ _ _ _ _ _ _ _ _ _ _]
      tunnel: w1318 -> [w1327 w1379 w1399 w1417 w1434 w1455 w1503 w1518 _ w1674 _ _ _ _ _ _]
      tunnel: w1320 -> [w1326 w1378 w1398 w1416 w1433 w1454 w1502 w1517 _ w1672 _ _ _ _ _ _]
      tunnel: [_ _ _ _ _ _ _ _ _ _ _ _ _ _ _ w1862] -> w1319
      event "Got DNA bead": Value Change {
        n811 = event-data() -> ()  [unwired: 1 in, 5 out]
        n812 = flat-sequence {
          tunnel: w1326 -> [w1330]
          tunnel: ["Cal @ Delta (nm)"] -> w1322
          tunnel: w1327 -> [w1332]
          tunnel: [w1346] -> w1325
          tunnel: w1322 -> [w1345]
          tunnel: w1325 -> [w1367]
          tunnel: [w1367] -> w1324
          tunnel: w1324 -> [w1369]
          tunnel: [w1369] -> w1323
          tunnel: w1323 -> [w1371]
          frame #0 {
            n813 = local read "Saved stage positions"() -> (w1333:dbl[][])
            n814 = property on="Inject Sample" class="Bool (strict)"("Val(Sgnl)"=TRUE ("Value (Signaling)")) -> ()  [unwired: 2 in, 2 out]
            n815 = disable-structure shown="Disabled" {
              frame Disabled {
                n816 = property on="Inject Pump 2" class="Bool (strict)"("Val(Sgnl)"=FALSE ("Inject Pump 2")) -> ()  [unwired: 2 in, 2 out]
              }
              frame Enabled {
              }
            }
            n817 = local write "Stage moving"(TRUE ("Stage moving")) -> ()
            n818 = property on="Trap delta (nm)" class="DigNum (strict)"("Val(Sgnl)"="Cal @ Delta (nm)") -> ()  [unwired: 2 in, 2 out]
            n819 = call "move to saved stage position.vi"("error in"=w1330, "Stage VISA resource name in"=w1332, "Position"="Cal stage position", "Saved Stage Positions"=w1333) -> ()  [unwired: 2 out]
          }
          frame #1 {
            n820 = local write "Stage moving"(FALSE ("Stage moving")) -> ()
            n821 = property on="Inject Sample" class="Bool (strict)"("Val(Sgnl)"=FALSE ("Value (Signaling)")) -> ()  [unwired: 2 in, 2 out]
            n822 = call <vilib>:"Beep.vi"() -> ()  [unwired: 12 in]
          }
          frame #2 {
            # "increased from 1000 to 5000 v6.4. \nMar.7,2018."
            n823 = Wait (ms)(milliseconds to wait=u32 5000) -> ()  [unwired: 1 out]
          }
          frame #3 {
            n824 = property on="Save cal" class="Bool (strict)"("Val(Sgnl)"=TRUE ("Value (Signaling)")) -> ()  [unwired: 2 in, 2 out]
          }
          frame #4 {
            n825 = Wait (ms)(milliseconds to wait=u32 2000) -> ()  [unwired: 1 out]
          }
          frame #5 {
            n826 = while {
              stop <- w1342 stop-if-true
              n827 = local read "Saving"() -> (w1343:bool)
              n828 = Not(x=w1343) -> (.not. x?=w1342:bool)
              n829 = Wait (ms)(milliseconds to wait=u32 100) -> ()  [unwired: 1 out]
            }
          }
          frame #6 {
            n830 = Wait (ms)(milliseconds to wait=u32 2000) -> ()  [unwired: 1 out]
          }
          frame #7 {
            n831 = stacked-sequence {
              tunnel: [_ _ _ _ _ _ w1361 _] -> w1346
              tunnel: w1345 -> [_ _ _ _ _ _ _ w1366]
              frame #0 {
                n832 = property on="Trap delta (nm)" class="DigNum (strict)"("Val(Sgnl)"="Offset @ Delta (nm)") -> ()  [unwired: 2 in, 2 out]
                n833 = Replace Array Subset(array=i32[] [0], new element="Offset raster set", index=0) -> (w1350:i32[])
                n834 = property on="Scan Parameters" class="Arr (strict)"("Index Values"=w1350) -> ()  [unwired: 2 in, 2 out]
              }
              frame #1 {
                n835 = Wait (ms)(milliseconds to wait=u32 200) -> ()  [unwired: 1 out]
              }
              frame #2 {
                n836 = property on="Load param" class="Bool (strict)"("Val(Sgnl)"=TRUE ("Load param")) -> ()  [unwired: 2 in, 2 out]
              }
              frame #3 {
                n837 = Wait (ms)(milliseconds to wait=u32 200) -> ()  [unwired: 1 out]
              }
              frame #4 {
                # "Only continue if there is no buffer\noverflow error"
                n838 = local read "Buffer Overflow"() -> (w1356:bool)
                n839 = Not(x=w1356) -> (.not. x?=w1355:bool)
                n840 = case shown="True" w1355 {
                  frame False {
                  }
                  frame True {
                    n841 = property on="Raster scan" class="Bool (strict)"("Val(Sgnl)"=TRUE ("Value (Signaling)")) -> ()  [unwired: 2 in, 2 out]
                  }
                }
              }
              frame #5 {
                n842 = local read "Buffer Overflow"() -> (w1359:bool)
                n843 = Not(x=w1359) -> (.not. x?=w1358:bool)
                n844 = case shown="True" w1358 {
                  frame False {
                  }
                  frame True {
                    n845 = Wait (ms)(milliseconds to wait=u32 2000) -> ()  [unwired: 1 out]
                  }
                }
              }
              frame #6 {
                n846 = local read "Buffer Overflow"() -> (w1362:bool)
                n847 = Not(x=w1362) -> (.not. x?=w1361:bool)
                n848 = case shown="True" w1361 {
                  frame False {
                  }
                  frame True {
                    n849 = while {
                      stop <- w1364 stop-if-true
                      n850 = local read "Saving"() -> (w1365:bool)
                      n851 = Not(x=w1365) -> (.not. x?=w1364:bool)
                      n852 = Wait (ms)(milliseconds to wait=u32 100) -> ()  [unwired: 1 out]
                    }
                  }
                }
              }
              frame #7 {
                n853 = property on="Trap delta (nm)" class="DigNum (strict)"("Val(Sgnl)"=w1366) -> ()  [unwired: 2 in, 2 out]
              }
            }
          }
          frame #8 {
            n854 = case shown="True" w1367 {
              frame False {
              }
              frame True {
                n855 = property on="Read Cal" class="Bool (strict)"("Val(Sgnl)"=TRUE ("Value (Signaling)")) -> ()  [unwired: 2 in, 2 out]
              }
            }
          }
          frame #9 {
            n856 = case shown="True" w1369 {
              frame False {
              }
              frame True {
                n857 = Wait (ms)(milliseconds to wait=u32 1000) -> ()  [unwired: 1 out]
              }
            }
          }
          frame #10 {
            n858 = case shown="True" w1371 {
              frame False {
              }
              frame True {
                n859 = property on="Fish" class="Bool (strict)"("Val(Sgnl)"=TRUE ("Value (Signaling)")) -> ()  [unwired: 2 in, 2 out]
                n860 = case shown="False" "Flow on\nwhile fish?" {
                  frame False {
                    n861 = property on="Inject Sample" class="Bool (strict)"("Val(Sgnl)"=FALSE) -> ()  [unwired: 2 in, 2 out]
                  }
                  frame True {
                    n862 = property on="Inject Sample" class="Bool (strict)"("Val(Sgnl)"=TRUE ("Value (Signaling)")) -> ()  [unwired: 2 in, 2 out]
                  }
                }
              }
            }
          }
        }
        n863 = local write "Got DNA bead"(FALSE) -> ()
      }
      event "Dump beads": Value Change {
        n864 = event-data() -> ()  [unwired: 1 in, 5 out]
        n865 = flat-sequence {
          tunnel: w1378 -> [w1382]
          tunnel: w1379 -> [w1383]
          tunnel: [w1383] -> w1377
          tunnel: [w1382] -> w1376
          tunnel: w1377 -> [w1386]
          tunnel: w1376 -> [w1385]
          frame #0 {
            w1380 = FALSE ("Fish")
            n866 = local read "Saving"() -> (w1381:bool)
            n867 = local write "Force Feedback 2"(w1380) -> ()
            n868 = local write "Pause dwell"(w1380) -> ()
            n869 = local write "Force Feedback 1"(w1380) -> ()
            n870 = local write "Dump beads"(w1380) -> ()
            n871 = property on="Stop saving" class="Bool (strict)"("Val(Sgnl)"=w1381) -> ()  [unwired: 2 in, 2 out]
            n872 = local write "Fish"(w1380) -> ()
          }
          frame #1 {
            n873 = local read "Saved stage positions"() -> (w1388:dbl[][])
            n874 = case shown="True" "Flow on\ndump?" {
              frame False {
              }
              frame True {
                n875 = property on="Inject Sample" class="Bool (strict)"("Val(Sgnl)"=TRUE ("Value (Signaling)")) -> ()  [unwired: 2 in, 2 out]
              }
            }
            n876 = local write "Stage moving"(TRUE ("Stage moving")) -> ()
            n877 = call "move to saved stage position.vi"("error in"=w1385, "Stage VISA resource name in"=w1386, "Position"=5, "Saved Stage Positions"=w1388) -> ()  [unwired: 2 out]
          }
          frame #2 {
            n878 = local read "Shutter 1 (B)"() -> (w1393:bool)
            n879 = local read "Shutter 2 (A)"() -> (w1392:bool)
            n880 = call <vilib>:"Beep.vi"() -> ()  [unwired: 12 in]
            n881 = case shown="True" w1393 {
              frame False {
              }
              frame True {
                n882 = property on="Shutter 1 (B)" class="Bool (strict)"("Val(Sgnl)"=FALSE ("Value (Signaling)")) -> ()  [unwired: 2 in, 2 out]
              }
            }
            n883 = case shown="True" w1392 {
              frame False {
              }
              frame True {
                n884 = property on="Shutter 2 (A)" class="Bool (strict)"("Val(Sgnl)"=FALSE) -> ()  [unwired: 2 in, 2 out]
              }
            }
            n885 = local write "Stage moving"(FALSE ("Stage moving")) -> ()
            n886 = local write "Tether"(FALSE ("Tether")) -> ()
          }
          frame #3 {
            n887 = property on="Move Cap. 2 (ADig Top)" class="Bool (strict)"("Val(Sgnl)"=TRUE ("Value (Signaling)")) -> ()  [unwired: 2 in, 2 out]
          }
        }
      }
      event "Move Cap. 2 (ADig Top)": Value Change {
        n888 = event-data() -> ()  [unwired: 1 in, 5 out]
        n889 = flat-sequence {
          tunnel: w1399 -> [w1403]
          tunnel: w1398 -> [w1402]
          frame #0 {
            n890 = local read "Saved stage positions"() -> (w1401:dbl[][])
            n891 = case shown="True" "Flow on\ncap 2?" {
              frame False {
              }
              frame True {
                n892 = property on="Inject Sample" class="Bool (strict)"("Val(Sgnl)"=TRUE ("Value (Signaling)")) -> ()  [unwired: 2 in, 2 out]
              }
            }
            n893 = local write "Move Cap. 2 (ADig Top)"(FALSE ("Move Cap. 2 (ADig Top)")) -> ()
            n894 = local write "Stage moving"(TRUE ("Stage moving")) -> ()
            n895 = call "move to saved stage position.vi"("error in"=w1402, "Stage VISA resource name in"=w1403, "Position"=2, "Saved Stage Positions"=w1401) -> ()  [unwired: 2 out]
          }
          frame #1 {
            # "Make sure you don't reverse\nwhich is ON and OFF"
            n896 = local read "Cal @ Delta (nm)"() -> (w1411:dbl)
            n897 = local write "Stage moving"(FALSE ("Stage moving")) -> ()
            n898 = call <vilib>:"Beep.vi"() -> ()  [unwired: 12 in]
            n899 = property on="Trap delta (nm)" class="DigNum (strict)"("Val(Sgnl)"=w1411) -> ()  [unwired: 2 in, 2 out]
            n900 = property class="TabCtl (strict)"("Val(Sgnl)"=T5."Status" ("Value (Signaling)")) -> ()  [unwired: 2 in, 2 out]
            n901 = disable-structure shown="Disabled" {
              frame Disabled {
                n902 = property on="Inject Pump 1" class="Bool (strict)"("Val(Sgnl)"=TRUE ("Inject Pump 2")) -> ()  [unwired: 2 in, 2 out]
              }
              frame Enabled {
              }
            }
            n903 = local read "Shutter 2 (A)"() -> (w1410:bool)
            n904 = case shown="False" w1410 {
              frame False {
                n905 = property on="Shutter 2 (A)" class="Bool (strict)"("Val(Sgnl)"=TRUE ("Value (Signaling)")) -> ()  [unwired: 2 in, 2 out]
              }
              frame True {
              }
            }
            n906 = property on="Inject Sample" class="Bool (strict)"("Val(Sgnl)"=FALSE ("Value (Signaling)")) -> ()  [unwired: 2 in, 2 out]
          }
        }
      }
      event "Got ADig bead": Value Change {
        n907 = event-data() -> ()  [unwired: 1 in, 5 out]
        n908 = flat-sequence {
          tunnel: w1417 -> [w1421]
          tunnel: w1416 -> [w1420]
          frame #0 {
            n909 = local read "Saved stage positions"() -> (w1423:dbl[][])
            n910 = property on="Inject Pump 1" class="Bool (strict)"("Val(Sgnl)"=FALSE ("Inject Pump 2")) -> ()  [unwired: 2 in, 2 out]
            n911 = case shown="True" "Flow on\ncap 1?" {
              frame False {
              }
              frame True {
                n912 = property on="Inject Sample" class="Bool (strict)"("Val(Sgnl)"=TRUE ("Value (Signaling)")) -> ()  [unwired: 2 in, 2 out]
              }
            }
            n913 = local write "Stage moving"(TRUE ("Stage moving")) -> ()
            n914 = call "move to saved stage position.vi"("error in"=w1420, "Stage VISA resource name in"=w1421, "Position"=1, "Saved Stage Positions"=w1423) -> ()  [unwired: 2 out]
          }
          frame #1 {
            n915 = local read "Shutter 1 (B)"() -> (w1427:bool)
            n916 = disable-structure shown="Disabled" {
              frame Disabled {
                n917 = property on="Inject Pump 2" class="Bool (strict)"("Val(Sgnl)"=TRUE ("Inject Pump 2")) -> ()  [unwired: 2 in, 2 out]
              }
              frame Enabled {
              }
            }
            n918 = local write "Stage moving"(FALSE ("Stage moving")) -> ()
            n919 = case shown="False" w1427 {
              frame False {
                n920 = property on="Shutter 1 (B)" class="Bool (strict)"("Val(Sgnl)"=TRUE ("Value (Signaling)")) -> ()  [unwired: 2 in, 2 out]
              }
              frame True {
              }
            }
            n921 = property on="Inject Sample" class="Bool (strict)"("Val(Sgnl)"=FALSE ("Value (Signaling)")) -> ()  [unwired: 2 in, 2 out]
            n922 = call <vilib>:"Beep.vi"() -> ()  [unwired: 12 in]
          }
        }
        n923 = local write "Got ADig bead"(FALSE ("Got ADig bead")) -> ()
      }
      event "Set Position 1", "Set Position 2", "Set Position 3", "Set Position 4", "Set Position 5": Value Change {
        n924 = event-data() -> ()  [unwired: 1 in, 5 out]
        n925 = Build Array("Set Position 1", "Set Position 2", "Set Position 3", "Set Position 4", "Set Position 5") -> (w1446:bool[])
        n926 = Boolean Array To Number(Boolean array=w1446) -> (number=w1445:u32)
        n927 = call "Read Stage Position.vi"("error in"=w1433, "VISA resource name in"=w1434) -> ("Current Position"=w1431:cluster{dbl, dbl, dbl}, "error out"=→"Stage error":errorcluster)  [unwired: 1 in, 1 out]
        n928 = Logarithm Base 2(1:w1445) -> (0:w1439:dbl)
        n929 = Cluster To Array(cluster=w1431) -> (array=w1441:dbl[])
        n930 = Increment(x=w1439) -> (x+1=w1442:dbl)
        n931 = Build Array (concatenate)(w1442, w1441) -> (w1440:dbl[])
        n932 = Replace Array Subset(array="Saved stage positions", new element=w1440, index (row)=w1439) -> (w1443:dbl[][])  [unwired: 1 in]
        n933 = local write "Saved stage positions"(w1443) -> ()
      }
      event "Move to Position 2", "Move to Position 4", "Move to Position 3", "Move to Position 5", "Move to Position 1": Value Change {
        w1449 = FALSE
        n934 = event-data() -> ()  [unwired: 1 in, 5 out]
        n935 = Build Array("Move to Position 1", "Move to Position 2", "Move to Position 3", "Move to Position 4", "Move to Position 5") -> (w1458:bool[])
        n936 = Boolean Array To Number(Boolean array=w1458) -> (number=w1457:u32)
        n937 = Logarithm Base 2(1:w1457) -> (0:w1456:dbl)
        n938 = flat-sequence {
          tunnel: w1456 -> [w1467]
          tunnel: w1455 -> [w1466]
          tunnel: w1454 -> [w1465]
          tunnel: [w1460] -> w1448
          tunnel: w1448 -> [w1477]
          frame #0 {
            # "only change move time when \nsaving move in T and calibrating is F"
            n939 = local read "Saved stage positions"() -> (w1468:dbl[][])
            n940 = property on="Saving Move" class="Bool (strict)"() -> ("Value"=w1462:bool)  [unwired: 2 in, 2 out]
            n941 = property on="Calibrating" class="Bool (strict)"() -> ("Value"=w1463:bool)  [unwired: 2 in, 2 out]
            n942 = Not(x=w1463) -> (.not. x?=w1461:bool)
            n943 = Increment(x=w1467) -> (x+1=w1460:dbl)
            n944 = And(x=w1462, y=w1461) -> (x .and. y?=w1464:bool)
            n945 = case shown="True" w1464 {
              frame False {
              }
              frame True {
                n946 = Get Date/Time In Seconds() -> (seconds since 1Jan1904=w1474:timestamp)
                n947 = Format Date/Time String(time format string (%c)="%H:%M:%S%3u", seconds (now)=w1474, UTC format=TRUE) -> (date/time string=w1473:string)
                n948 = call <vilib>:"Space Constant.vi"() -> ("String"=w1472:string)
                n949 = Concatenate Strings(w1473, w1472, "moving") -> (w1470:string)
                n950 = property on="Move time" class="Str"("Val(Sgnl)"=w1470) -> ()  [unwired: 2 in, 2 out]
              }
            }
            n951 = call "move to saved stage position.vi"("error in"=w1465, "Stage VISA resource name in"=w1466, "Position"=w1460, "Saved Stage Positions"=w1468) -> ()  [unwired: 2 out]
            n952 = call <vilib>:"Beep.vi"() -> ()  [unwired: 12 in]
            "Stage moving" <- TRUE ("Stage moving")
          }
          frame #1 {
            n953 = property on="Saving Move" class="Bool (strict)"() -> ("Value"=w1479:bool)  [unwired: 2 in, 2 out]
            n954 = property on="Calibrating" class="Bool (strict)"() -> ("Value"=w1480:bool)  [unwired: 2 in, 2 out]
            n955 = call <vilib>:"Beep.vi"() -> ()  [unwired: 12 in]
            n956 = Not(x=w1480) -> (.not. x?=w1478:bool)
            n957 = local write "Stage moving"(FALSE ("Stage moving")) -> ()
            n958 = And(x=w1479, y=w1478) -> (x .and. y?=w1481:bool)
            n959 = case shown="True" w1481 {
              tunnel: w1477 -> [_ w1485]
              frame False {
              }
              frame True {
                n960 = Get Date/Time In Seconds() -> (seconds since 1Jan1904=w1489:timestamp)
                n961 = Format Date/Time String(time format string (%c)="%H:%M:%S%3u", seconds (now)=w1489, UTC format=TRUE) -> (date/time string=w1488:string)
                n962 = Number To Decimal String(number=w1485, width (-)=i16 1) -> (decimal integer string=w1483:string)
                n963 = call <vilib>:"Space Constant.vi"() -> ("String"=w1486:string)
                n964 = Concatenate Strings(w1488, w1486, w1483) -> (w1487:string)
                n965 = property on="Move time" class="Str"("Val(Sgnl)"=w1487) -> ()  [unwired: 2 in, 2 out]
              }
            }
          }
        }
        n966 = local write "Move to Position 1"(w1449) -> ()
        n967 = local write "Move to Position 2"(w1449) -> ()
        n968 = local write "Move to Position 3"(w1449) -> ()
        n969 = local write "Move to Position 4"(w1449) -> ()
        n970 = local write "Move to Position 5"(w1449) -> ()
      }
      event "Set Current\nPos to (0,0,0)": Value Change {
        w1493 = ";" ("string")
        # "DH is \"Define Home\" -KW"
        n971 = event-data() -> ()  [unwired: 1 in, 5 out]
        n972 = local write "Set Current\nPos to (0,0,0)"(FALSE ("Set Current\nPos to (0,0,0)")) -> ()
        n973 = call-poly "VISA Configure Serial Port"("VISA resource name"=w1503, "baud rate (9600)"=u32 19200, "error in (no error)"=w1502) -> ("VISA resource name out"=w1497:refnum<visa-resource-name>, "error out"=w1496:errorcluster)  [unwired: 11 in]
        n974 = Concatenate Strings("1DH" ("string"), w1493, "2DH" ("string"), w1493, "3DH" ("string"), "\r") -> (w1495:string)
        n975 = VISA Write(VISA resource name=w1497, write buffer=w1495, error in (no error)=w1496) -> (error out=w1494:errorcluster)  [unwired: 2 out]
        n976 = local write "Stage error"(w1494) -> ()
      }
      event "Dip": Value Change {
        n977 = event-data() -> ()  [unwired: 1 in, 5 out]
        n978 = property on="Calibrating" class="Bool (strict)"() -> ("Value"=w1510:bool)  [unwired: 2 in, 2 out]
        n979 = Not(x=w1510) -> (.not. x?=w1508:bool)
        n980 = property on="Saving Move" class="Bool (strict)"() -> ("Value"=w1509:bool)  [unwired: 2 in, 2 out]
        n981 = And(x=w1509, y=w1508) -> (x .and. y?=w1507:bool)
        n982 = flat-sequence {
          tunnel: w1518 -> [w1522]
          tunnel: w1517 -> [w1521]
          tunnel: [w1523] -> w1515
          tunnel: [w1522] -> w1513
          tunnel: [w1521] -> w1511
          tunnel: w1507 -> [w1520]
          tunnel: ["Dip position"] -> w1506
          tunnel: [w1539] -> w1516
          tunnel: w1515 -> [w1539]
          tunnel: [w1538] -> w1514
          tunnel: w1513 -> [w1538]
          tunnel: [w1537] -> w1512
          tunnel: w1511 -> [w1537]
          tunnel: w1507 -> [w1533]
          tunnel: w1506 -> [w1532]
          tunnel: w1516 -> [w1570]
          tunnel: w1514 -> [w1569]
          tunnel: w1512 -> [w1568]
          tunnel: w1507 -> [w1566]
          tunnel: ["Start/Return position"] -> w1505
          tunnel: w1507 -> [w1579]
          tunnel: w1505 -> [w1578]
          frame #0 {
            n983 = local read "Saved stage positions"() -> (w1523:dbl[][])
            n984 = case shown="True" w1520 {
              frame False {
              }
              frame True {
                n985 = Get Date/Time In Seconds() -> (seconds since 1Jan1904=w1531:timestamp)
                n986 = call <vilib>:"Space Constant.vi"() -> ("String"=w1527:string)
                n987 = Format Date/Time String(time format string (%c)="%H:%M:%S%3u", seconds (now)=w1531, UTC format=TRUE) -> (date/time string=w1528:string)
                n988 = Concatenate Strings(w1528, w1527, "moving") -> (w1526:string)
                n989 = property on="Move time" class="Str"("Val(Sgnl)"=w1526) -> ()  [unwired: 2 in, 2 out]
              }
            }
            n990 = local write "Stage moving"(TRUE) -> ()
            n991 = call "move to saved stage position.vi"("error in"=w1521, "Stage VISA resource name in"=w1522, "Position"="Dip position", "Saved Stage Positions"=w1523) -> ()  [unwired: 2 out]
          }
          frame #1 {
            n992 = node-c288() -> (w1536:T14)  [unwired: 4 in]
            n993 = case shown="True" w1533 {
              tunnel: w1532 -> [_ w1543]
              frame False {
              }
              frame True {
                n994 = Get Date/Time In Seconds() -> (seconds since 1Jan1904=w1548:timestamp)
                n995 = Number To Decimal String(number=w1543, width (-)=i16 1) -> (decimal integer string=w1542:string)
                n996 = Format Date/Time String(time format string (%c)="%H:%M:%S%3u", seconds (now)=w1548, UTC format=TRUE) -> (date/time string=w1541:string)
                n997 = call <vilib>:"Space Constant.vi"() -> ("String"=w1545:string)
                n998 = Concatenate Strings(w1541, w1545, w1542) -> (w1540:string)
                n999 = property on="Move time" class="Str"("Val(Sgnl)"=w1540) -> ()  [unwired: 2 in, 2 out]
              }
            }
            n1000 = timed-loop {
              timing: w1536 -> [_]
              timing-out: [_] -> w1535
              i -> [w1559]
              stop <- w1552 stop-if-true
              n1001 = node-c288() -> ()  [unwired: 1 in, 1 out]
              n1002 = local read "Cancel Rep\n Dip"() -> (w1549:bool)
              n1003 = Greater Or Equal?(x=w1559, y="Dip duration") -> (x >= y?=w1555:bool)
              n1004 = local read "Dump beads"() -> (w1550:bool)
              n1005 = Or(x=w1555, y="Cancel dwell") -> (x .or. y?=w1554:bool)
              n1006 = Not(x="Pause dwell") -> (.not. x?=w1556:bool)
              n1007 = node-c288() -> ()  [unwired: 1 in, 1 out]
              n1008 = And(x=w1556, y=w1554) -> (x .and. y?=w1553:bool)
              n1009 = Compound Arithmetic op=OR(w1553, w1550, w1549) -> (w1552:bool)
              "Dip elasped time" <- w1559
            }
            n1010 = local write "Stage moving"(FALSE ("Stage moving")) -> ()
            n1011 = node-c288(w1535) -> ()  [unwired: 1 out]
          }
          frame #2 {
            w1564 = FALSE ("Cancel dwell")
            n1012 = case shown="True" w1566 {
              frame False {
              }
              frame True {
                n1013 = Get Date/Time In Seconds() -> (seconds since 1Jan1904=w1577:timestamp)
                n1014 = Format Date/Time String(time format string (%c)="%H:%M:%S%3u", seconds (now)=w1577, UTC format=TRUE) -> (date/time string=w1574:string)
                n1015 = call <vilib>:"Space Constant.vi"() -> ("String"=w1573:string)
                n1016 = Concatenate Strings(w1574, w1573, "moving") -> (w1571:string)
                n1017 = property on="Move time" class="Str"("Val(Sgnl)"=w1571) -> ()  [unwired: 2 in, 2 out]
              }
            }
            n1018 = local write "Cancel dwell"(w1564) -> ()
            n1019 = local write "Cancel Rep\n Dip"(w1564) -> ()
            n1020 = local write "Stage moving"(TRUE) -> ()
            n1021 = call "move to saved stage position.vi"("error in"=w1568, "Stage VISA resource name in"=w1569, "Position"="Start/Return position", "Saved Stage Positions"=w1570) -> ()  [unwired: 2 out]
          }
          frame #3 {
            n1022 = case shown="True" w1579 {
              tunnel: w1578 -> [_ w1581]
              frame False {
              }
              frame True {
                n1023 = Get Date/Time In Seconds() -> (seconds since 1Jan1904=w1589:timestamp)
                n1024 = Number To Decimal String(number=w1581, width (-)=i16 1) -> (decimal integer string=w1582:string)
                n1025 = call <vilib>:"Space Constant.vi"() -> ("String"=w1586:string)
                n1026 = Format Date/Time String(time format string (%c)="%H:%M:%S%3u", seconds (now)=w1589, UTC format=TRUE) -> (date/time string=w1583:string)
                n1027 = Concatenate Strings(w1583, w1586, w1582) -> (w1584:string)
                n1028 = property on="Move time" class="Str"("Val(Sgnl)"=w1584) -> ()  [unwired: 2 in, 2 out]
              }
            }
            n1029 = local write "Stage moving"(FALSE ("Stage moving")) -> ()
          }
          frame #4 {
            n1030 = local write "Dip"(FALSE ("Dip")) -> ()
          }
        }
      }
      event "Grid Movable Trap": Value Change {
        n1031 = event-data() -> ()  [unwired: 1 in, 6 out]
        n1032 = flat-sequence {
          frame #0 {
            n1033 = local write "Shutter 1 (B)"(FALSE ("Shutter 1 (B)")) -> ()
          }
          frame #1 {
            n1034 = while {
              i -> [w1601]
              stop <- w1593 stop-if-true
              n1035 = Multiply(x=0.5, y=w1601) -> (x*y=w1599:dbl)
              n1036 = Add(x=0.0, y=w1599) -> (x+y=w1597:dbl)
              n1037 = while {
                tunnel: w1597 -> [w1607]
                tunnel: 0.5 ("x") -> [w1602]
                i -> [w1611]
                stop <- w1610 stop-if-true
                n1038 = flat-sequence {
                  tunnel: w1611 -> [w1626]
                  tunnel: [w1616] -> w1608
                  tunnel: w1607 -> [w1618]
                  tunnel: [w1621] -> w1605
                  tunnel: [w1620] -> w1603
                  tunnel: w1602 -> [w1614]
                  tunnel: [w1630] -> w1606
                  tunnel: w1605 -> [w1630]
                  tunnel: [w1629] -> w1604
                  tunnel: w1603 -> [w1629]
                  tunnel: w1606 -> [w1633]
                  tunnel: w1604 -> [w1632]
                  frame #0 {
                    w1612 = i16 2 ("precision (6)")
                    w1613 = i16 5 ("width (-)")
                    w1615 = 100.0 ("y")
                    n1039 = Multiply(x=w1614, y=w1626) -> (x*y=w1627:dbl)
                    n1040 = Add(x=0.0, y=w1627) -> (x+y=w1616:dbl)
                    n1041 = Multiply(x=w1618, y=w1615) -> (x*y=w1619:dbl)
                    n1042 = Multiply(x=w1616, y=w1615) -> (x*y=w1617:dbl)
                    n1043 = Build Array(w1616, w1618) -> (w1625:dbl[])
                    n1044 = Number To Fractional String(number=w1618, width (-)=w1613, precision (6)=w1612) -> (F-format string=→"moveY":string)  [unwired: 1 in]
                    n1045 = Number To Decimal String(number=w1619) -> (decimal integer string=w1620:string)  [unwired: 1 in]
                    n1046 = Number To Decimal String(number=w1617) -> (decimal integer string=w1621:string)  [unwired: 1 in]
                    n1047 = Number To Fractional String(number=w1616, width (-)=w1613, precision (6)=w1612) -> (F-format string=→"moveX":string)  [unwired: 1 in]
                    n1048 = Array To Cluster(array=w1625) -> (cluster=w1624:cluster{"[0]":dbl, "[1]":dbl})
                    n1049 = property on="Trap position (V)" class="Clust (strict)"("Val(Sgnl)"=w1624) -> ()  [unwired: 2 in, 2 out]
                  }
                  frame #1 {
                    n1050 = Wait (ms)(milliseconds to wait=u32 1000) -> ()  [unwired: 1 out]
                  }
                  frame #2 {
                    n1051 = while {
                      tunnel: w1633 -> [w1635]
                      tunnel: w1632 -> [w1634]
                      i -> [w1638]
                      stop <- w1636 stop-if-true
                      n1052 = flat-sequence {
                        tunnel: w1635 -> [w1642]
                        tunnel: w1634 -> [w1641]
                        frame #0 {
                          w1639 = "_" ("string")
                          n1053 = local read "Image Index"() -> (w1651:dbl)
                          n1054 = Concatenate Strings("GridMove_" ("string"), w1642, w1639, w1641, w1639) -> (w1640:string)
                          n1055 = call "Create new save file.vi"("Insert"=w1640, "Ext"=".bmp" ("string"), "Index In"=w1651) -> ("Path Out"=w1647:path, "Index Out"=w1649:dbl)
                          n1056 = local read "GreyscaleArray"() -> (w1645:u32[])
                          n1057 = local read "image8bitArray"() -> (w1646:u8[][])
                          n1058 = Increment(x=w1649) -> (x+1=w1648:dbl)
                          n1059 = local write "Image Index"(w1648) -> ()
                          n1060 = call <vilib>:"Flatten Pixmap.vi"("colors"=w1645, "8-bit pixmap"=w1646) -> ("image data"=w1644:T18)  [unwired: 4 in, 5 out]
                          n1061 = call <vilib>:"Write BMP File.vi"("image data"=w1644, "path to BMP file"=w1647) -> ()  [unwired: 1 in, 9 out]
                        }
                        frame #1 {
                          n1062 = Wait (ms)(milliseconds to wait=u32 50) -> ()  [unwired: 1 out]
                        }
                      }
                      n1063 = Equal?(x=w1638, y=9) -> (x = y?=w1636:bool)
                    }
                  }
                  frame #3 {
                    n1064 = Wait (ms)(milliseconds to wait=u32 100) -> ()  [unwired: 1 out]
                  }
                }
                n1065 = Equal?(x=w1608, y=5.0) -> (x = y?=w1610:bool)
              }
              n1066 = local read "Stop"() -> (w1595:bool)
              n1067 = Equal?(x=w1597, y=2.0) -> (x = y?=w1594:bool)
              n1068 = Or(x=w1595, y=w1594) -> (x .or. y?=w1593:bool)
            }
          }
          frame #2 {
            n1069 = property on="Shutter 2 (A)" class="Bool (strict)"("Val(Sgnl)"=FALSE ("Shutter 2 (A)")) -> ()  [unwired: 2 in, 2 out]
            n1070 = property on="Inject Sample" class="Bool (strict)"("Val(Sgnl)"=TRUE ("Inject Sample")) -> ()  [unwired: 2 in, 2 out]
          }
          frame #3 {
            n1071 = Wait (ms)(milliseconds to wait=u32 10000) -> ()  [unwired: 1 out]
          }
          frame #4 {
            n1072 = property on="Inject Sample" class="Bool (strict)"("Val(Sgnl)"=FALSE ("Inject Sample")) -> ()  [unwired: 2 in, 2 out]
          }
          frame #5 {
            n1073 = while {
              i -> [w1660]
              stop <- w1658 stop-if-true
              n1074 = flat-sequence {
                frame #0 {
                  n1075 = local read "image8bitArray"() -> (w1669:u8[][])
                  n1076 = local read "GreyscaleArray"() -> (w1668:u32[])
                  n1077 = local read "Image Index"() -> (w1667:dbl)
                  n1078 = call "Create new save file.vi"("Insert"="background_" ("string"), "Ext"=".bmp" ("string"), "Index In"=w1667) -> ("Path Out"=w1662:path, "Index Out"=w1664:dbl)
                  n1079 = call <vilib>:"Flatten Pixmap.vi"("colors"=w1668, "8-bit pixmap"=w1669) -> ("image data"=w1661:T18)  [unwired: 4 in, 5 out]
                  n1080 = Increment(x=w1664) -> (x+1=w1663:dbl)
                  n1081 = call <vilib>:"Write BMP File.vi"("image data"=w1661, "path to BMP file"=w1662) -> ()  [unwired: 1 in, 9 out]
                  n1082 = local write "Image Index"(w1663) -> ()
                }
                frame #1 {
                  n1083 = Wait (ms)(milliseconds to wait=u32 500) -> ()  [unwired: 1 out]
                }
              }
              n1084 = Equal?(x=w1660, y=9) -> (x = y?=w1658:bool)
            }
          }
          frame #6 {
            n1085 = local write "Grid Movable Trap"(FALSE ("Grid Movable Trap")) -> ()
          }
        }
      }
      event "Repeat Dip": Value Change {
        n1086 = event-data() -> ()  [unwired: 1 in, 6 out]
        n1087 = local read "Saved stage positions"() -> (w1675:dbl[][])
        n1088 = local read "Calibrating"() -> (w1678:bool)
        n1089 = local read "Saving Move"() -> (w1677:bool)
        n1090 = Not(x=w1678) -> (.not. x?=w1676:bool)
        n1091 = And(x=w1677, y=w1676) -> (x .and. y?=w1673:bool)
        n1092 = flat-sequence {
          tunnel: w1675 -> [w1682]
          tunnel: w1674 -> [w1681]
          tunnel: w1673 -> [w1680]
          tunnel: w1672 -> [w1679]
          frame #0 {
            n1093 = while {
              tunnel: w1682 -> [w1702]
              tunnel: w1681 -> [w1699]
              tunnel: w1680 -> [w1696]
              tunnel: w1680 -> [w1695]
              tunnel: w1679 -> [w1694]
              tunnel: w1679 -> [w1693]
              i -> [w1703]
              stop <- w1684 stop-if-true
              n1094 = flat-sequence {
                tunnel: w1702 -> [w1708]
                tunnel: [w1708] -> w1700
                tunnel: w1699 -> [w1707]
                tunnel: [w1707] -> w1697
                tunnel: w1696 -> [w1706]
                tunnel: w1694 -> [w1705]
                tunnel: [w1704] -> w1689
                tunnel: [w1721] -> w1701
                tunnel: w1700 -> [w1721]
                tunnel: [w1720] -> w1698
                tunnel: w1697 -> [w1720]
                tunnel: w1695 -> [w1719]
                tunnel: w1689 -> [w1718]
                tunnel: w1683 -> [w1717]
                tunnel: w1701 -> [w1755]
                tunnel: w1698 -> [w1754]
                tunnel: w1695 -> [w1753]
                tunnel: w1693 -> [w1752]
                tunnel: [w1751] -> w1688
                tunnel: w1695 -> [w1766]
                tunnel: w1688 -> [w1765]
                tunnel: w1683 -> [w1764]
                frame #0 {
                  n1095 = case shown="True" w1706 {
                    frame False {
                    }
                    frame True {
                      n1096 = Get Date/Time In Seconds() -> (seconds since 1Jan1904=w1716:timestamp)
                      n1097 = call <vilib>:"Space Constant.vi"() -> ("String"=w1712:string)
                      n1098 = Format Date/Time String(time format string (%c)="%H:%M:%S%3u", seconds (now)=w1716, UTC format=TRUE) -> (date/time string=w1713:string)
                      n1099 = Concatenate Strings(w1713, w1712, "moving") -> (w1710:string)
                      n1100 = property on="Move time" class="Str"("Val(Sgnl)"=w1710) -> ()  [unwired: 2 in, 2 out]
                    }
                  }
                  n1101 = local read "Dip position"() -> (w1704:dbl)
                  n1102 = local write "Stage moving"(TRUE) -> ()
                  n1103 = call "move to saved stage position.vi"("error in"=w1705, "Stage VISA resource name in"=w1707, "Position"=w1704, "Saved Stage Positions"=w1708) -> ()  [unwired: 2 out]
                }
                frame #1 {
                  # "IN DIPPING POSITION"
                  n1104 = node-c288() -> (w1724:T14)  [unwired: 4 in]
                  n1105 = case shown="True" w1719 {
                    tunnel: w1718 -> [_ w1729]
                    frame False {
                    }
                    frame True {
                      n1106 = Get Date/Time In Seconds() -> (seconds since 1Jan1904=w1733:timestamp)
                      n1107 = Format Date/Time String(time format string (%c)="%H:%M:%S%3u", seconds (now)=w1733, UTC format=TRUE) -> (date/time string=w1728:string)
                      n1108 = Number To Decimal String(number=w1729, width (-)=i16 1) -> (decimal integer string=w1726:string)
                      n1109 = call <vilib>:"Space Constant.vi"() -> ("String"=w1727:string)
                      n1110 = Concatenate Strings(w1728, w1727, w1726) -> (w1725:string)
                      n1111 = property on="Move time" class="Str"("Val(Sgnl)"=w1725) -> ()  [unwired: 2 in, 2 out]
                    }
                  }
                  n1112 = timed-loop {
                    timing: w1724 -> [_]
                    timing-out: [_] -> w1723
                    tunnel: w1717 -> [w1734]
                    i -> [w1744]
                    stop <- w1736 stop-if-true
                    n1113 = node-c288() -> ()  [unwired: 1 in, 1 out]
                    n1114 = local read "Cancel dwell"() -> (w1742:bool)
                    n1115 = local read "Dip duration"() -> (w1743:dbl)
                    n1116 = local write "Dip elasped time"(w1744) -> ()
                    n1117 = local read "Dump beads"() -> (w1737:bool)
                    n1118 = To Double Precision Float(number=w1744) -> (double precision float=w1745:dbl)
                    n1119 = local read "Pause dwell"() -> (w1746:bool)
                    n1120 = Greater Or Equal?(x=w1745, y=w1743) -> (x >= y?=w1741:bool)
                    n1121 = Or(x=w1741, y=w1742) -> (x .or. y?=w1740:bool)
                    n1122 = Not(x=w1746) -> (.not. x?=w1739:bool)
                    n1123 = local read "Cancel Rep\n Dip"() -> (w1735:bool)
                    n1124 = And(x=w1739, y=w1740) -> (x .and. y?=w1738:bool)
                    n1125 = node-c288() -> ()  [unwired: 1 in, 1 out]
                    n1126 = Compound Arithmetic op=OR(w1735, w1738, w1737, w1734) -> (w1736:bool)
                  }
                  n1127 = local write "Stage moving"(FALSE) -> ()
                  n1128 = node-c288(w1723) -> ()  [unwired: 1 out]
                }
                frame #2 {
                  n1129 = case shown="True" w1753 {
                    frame False {
                    }
                    frame True {
                      n1130 = Get Date/Time In Seconds() -> (seconds since 1Jan1904=w1763:timestamp)
                      n1131 = call <vilib>:"Space Constant.vi"() -> ("String"=w1759:string)
                      n1132 = Format Date/Time String(time format string (%c)="%H:%M:%S%3u", seconds (now)=w1763, UTC format=TRUE) -> (date/time string=w1760:string)
                      n1133 = Concatenate Strings(w1760, w1759, "moving") -> (w1757:string)
                      n1134 = property on="Move time" class="Str"("Val(Sgnl)"=w1757) -> ()  [unwired: 2 in, 2 out]
                    }
                  }
                  n1135 = local read "Start/Return position"() -> (w1751:dbl)
                  n1136 = local write "Stage moving"(TRUE) -> ()
                  n1137 = call "move to saved stage position.vi"("error in"=w1752, "Stage VISA resource name in"=w1754, "Position"=w1751, "Saved Stage Positions"=w1755) -> ()  [unwired: 2 out]
                }
                frame #3 {
                  # "IN RETURN POSITION"
                  n1138 = node-c288() -> (w1769:T14)  [unwired: 4 in]
                  n1139 = timed-loop {
                    timing: w1769 -> [_]
                    timing-out: [_] -> w1768
                    tunnel: w1764 -> [w1779]
                    i -> [w1790]
                    stop <- w1781 stop-if-true
                    n1140 = node-c288() -> ()  [unwired: 1 in, 1 out]
                    n1141 = local read "Return duration"() -> (w1788:dbl)
                    n1142 = local read "Dump beads"() -> (w1782:bool)
                    n1143 = local read "Cancel dwell"() -> (w1786:bool)
                    n1144 = local write "Return elasped time"(w1790) -> ()
                    n1145 = To Double Precision Float(number=w1790) -> (double precision float=w1791:dbl)
                    n1146 = local read "Pause dwell"() -> (w1789:bool)
                    n1147 = Greater Or Equal?(x=w1791, y=w1788) -> (x >= y?=w1787:bool)
                    n1148 = Or(x=w1787, y=w1786) -> (x .or. y?=w1785:bool)
                    n1149 = local read "Cancel Rep\n Dip"() -> (w1780:bool)
                    n1150 = Not(x=w1789) -> (.not. x?=w1784:bool)
                    n1151 = node-c288() -> ()  [unwired: 1 in, 1 out]
                    n1152 = And(x=w1784, y=w1785) -> (x .and. y?=w1783:bool)
                    n1153 = Compound Arithmetic op=OR(w1780, w1783, w1782, w1779) -> (w1781:bool)
                  }
                  n1154 = case shown="True" w1766 {
                    tunnel: w1765 -> [_ w1774]
                    frame False {
                    }
                    frame True {
                      n1155 = Get Date/Time In Seconds() -> (seconds since 1Jan1904=w1778:timestamp)
                      n1156 = Format Date/Time String(time format string (%c)="%H:%M:%S%3u", seconds (now)=w1778, UTC format=TRUE) -> (date/time string=w1771:string)
                      n1157 = Number To Decimal String(number=w1774, width (-)=i16 1) -> (decimal integer string=w1773:string)
                      n1158 = call <vilib>:"Space Constant.vi"() -> ("String"=w1772:string)
                      n1159 = Concatenate Strings(w1771, w1772, w1773) -> (w1770:string)
                      n1160 = property on="Move time" class="Str"("Val(Sgnl)"=w1770) -> ()  [unwired: 2 in, 2 out]
                    }
                  }
                  n1161 = local write "Stage moving"(FALSE) -> ()
                  n1162 = node-c288(w1768) -> ()  [unwired: 1 out]
                }
              }
              n1163 = local read "Tether"() -> (w1685:bool)
              n1164 = Not(x=w1685) -> (.not. x?=w1683:bool)
              n1165 = Increment(x=w1703) -> (x+1=w1691:i32)
              "Dip #" <- w1691
              n1166 = property on="Cancel Rep\n Dip" class="Bool (strict)"() -> ("Value"=w1687:bool)  [unwired: 2 in, 2 out]
              n1167 = To Double Precision Float(number=w1691) -> (double precision float=w1690:dbl)
              n1168 = Greater Or Equal?(x=w1690, y="Dip attempts") -> (x >= y?=w1686:bool)
              n1169 = Compound Arithmetic op=OR(w1687, w1686, w1683) -> (w1684:bool)
            }
          }
          frame #1 {
            w1796 = FALSE
            n1170 = local write "Cancel Rep\n Dip"(w1796) -> ()
            n1171 = call <vilib>:"Beep.vi"() -> ()  [unwired: 12 in]
            n1172 = local write "Repeat Dip"(w1796) -> ()
          }
        }
      }
      event "Force FB script": Value Change {
        n1173 = event-data() -> ()  [unwired: 1 in, 5 out]
        n1174 = flat-sequence {
          frame #0 {
            n1175 = disable-structure shown="Disabled" {
              frame Disabled {
                n1176 = local read "# Samples/channel"() -> (w1799:i32)
                n1177 = local write "# Samples/channel (in)"(w1799) -> ()
              }
              frame Enabled {
              }
            }
            n1178 = local write "Force FB script"(FALSE ("Force FB script")) -> ()
            n1179 = property on="Trap delta (nm)" class="DigNum (strict)"("Val(Sgnl)"="Start trap delta (nm)") -> ()  [unwired: 2 in, 2 out]
          }
          frame #1 {
            n1180 = Wait (ms)(milliseconds to wait=u32 500) -> ()  [unwired: 1 out]
          }
          frame #2 {
            n1181 = property on="Set reading to\nsetpoint 1" class="Bool (strict)"("Val(Sgnl)"=TRUE ("Value (Signaling)")) -> ()  [unwired: 2 in, 2 out]
          }
          frame #3 {
            n1182 = Wait (ms)(milliseconds to wait=u32 300) -> ()  [unwired: 1 out]
          }
          frame #4 {
            n1183 = local write "Force Feedback 1"(TRUE ("Force Feedback")) -> ()
            n1184 = property on="Tabs" class="TabCtl (strict)"("Val(Sgnl)"=T24."Force Feedback" ("Value (Signaling)")) -> ()  [unwired: 2 in, 2 out]
          }
          frame #5 {
            n1185 = property on="Save Data" class="Bool (strict)"("Val(Sgnl)"=TRUE ("Value (Signaling)")) -> ()  [unwired: 2 in, 2 out]
          }
          frame #6 {
            n1186 = Multiply(x="Wait before dip (s)", y=1000) -> (x*y=w1806:dbl)
            n1187 = Wait (ms)(milliseconds to wait=w1806) -> ()  [unwired: 1 out]
          }
          frame #7 {
            n1188 = case shown="True" "Start dipping after?" {
              selector: "Start dipping after?" -> [_ w1811]
              frame False {
              }
              frame True {
                n1189 = property on="Dip" class="Bool (strict)"("Val(Sgnl)"=w1811) -> ()  [unwired: 2 in, 2 out]
              }
            }
            n1190 = property on="Remove offsets" class="Bool (strict)"("Val(Sgnl)"=TRUE ("Value (Signaling)")) -> ()  [unwired: 2 in, 2 out]
          }
        }
      }
      event "Move 0": Value Change {
        n1191 = event-data() -> ()  [unwired: 1 in, 5 out]
        n1192 = local write "Move 0"(FALSE) -> ()
        n1193 = call "HalfWavePlate.vi"("Degrees"="\"Degrees\" 0", "Motor"=0) -> ()  [unwired: 1 in]
      }
      event "Move 1": Value Change {
        n1194 = event-data() -> ()  [unwired: 1 in, 5 out]
        n1195 = local write "Move 1"(FALSE) -> ()
        n1196 = call "HalfWavePlate.vi"("Degrees"="\"Degrees\" 1", "Motor"=1) -> ()  [unwired: 1 in]
      }
      event "Save user params": Value Change {
        n1197 = event-data() -> ()  [unwired: 1 in, 6 out]
        n1198 = local write "Save user params"(FALSE) -> ()
        n1199 = call "save control values.vi"("User"="User") -> ()  [unwired: 8 in, 1 out]
      }
      event "Load user params": Value Change {
        # "Exceptions. Don't load these parameters."
        n1200 = event-data() -> ()  [unwired: 1 in, 6 out]
        n1201 = local write "Load user params"(FALSE) -> ()
        n1202 = flat-sequence {
          tunnel: [w1844] -> w1835
          tunnel: [w1843] -> w1833
          tunnel: [w1842] -> w1831
          tunnel: [w1841] -> w1829
          tunnel: [w1840] -> w1827
          tunnel: [w1839] -> w1825
          tunnel: [w1838] -> w1823
          tunnel: [w1837] -> w1820
          tunnel: [w1852] -> w1836
          tunnel: w1835 -> [w1852]
          tunnel: [w1851] -> w1834
          tunnel: w1833 -> [w1851]
          tunnel: [w1850] -> w1832
          tunnel: w1831 -> [w1850]
          tunnel: [w1849] -> w1830
          tunnel: w1829 -> [w1849]
          tunnel: [w1848] -> w1828
          tunnel: w1827 -> [w1848]
          tunnel: [w1847] -> w1826
          tunnel: w1825 -> [w1847]
          tunnel: [w1846] -> w1824
          tunnel: w1823 -> [w1846]
          tunnel: [w1845] -> w1821
          tunnel: w1820 -> [w1845]
          tunnel: w1836 -> [w1861]
          tunnel: w1834 -> [w1860]
          tunnel: w1832 -> [w1859]
          tunnel: w1830 -> [w1858]
          tunnel: w1828 -> [w1857]
          tunnel: w1826 -> [w1856]
          tunnel: w1824 -> [w1855]
          tunnel: w1821 -> [w1854]
          frame #0 {
            n1203 = local read "Force Feedback 2"() -> (w1837:bool)
            n1204 = local read "Force Feedback 1"() -> (w1838:bool)
            n1205 = local read "Shutter 1 (B)"() -> (w1844:bool)
            n1206 = local read "Shutter 2 (A)"() -> (w1843:bool)
            n1207 = local read "Inject Sample"() -> (w1841:bool)
            n1208 = local read "Trap delta (nm)"() -> (w1840:dbl)
            n1209 = local read "Save file index"() -> (w1839:i32)
            n1210 = local read "Fish"() -> (w1842:bool)
          }
          frame #1 {
            n1211 = local read "User"() -> (w1853:string)
            n1212 = call "retrieve control values.vi"("User"=w1853) -> ()  [unwired: 10 in, 1 out]
          }
          frame #2 {
            n1213 = local write "Force Feedback 1"(w1855) -> ()
            n1214 = local write "Force Feedback 2"(w1854) -> ()
            n1215 = local write "Trap delta (nm)"(w1857) -> ()
            n1216 = local write "Save file index"(w1856) -> ()
            n1217 = local write "Inject Sample"(w1858) -> ()
            n1218 = local write "Shutter 2 (A)"(w1860) -> ()
            n1219 = local write "Shutter 1 (B)"(w1861) -> ()
            n1220 = local write "Fish"(w1859) -> ()
          }
        }
      }
      event "Stop": Value Change {
        n1221 = event-data() -> ()  [unwired: 1 in, 5 out]
        n1222 = local read "Stop"() -> (w1862:bool)
      }
    }
    n1223 = node-c288() -> ()  [unwired: 1 in, 1 out]
  }
  n1224 = call-poly <vilib>:"DAQmx Create Virtual Channel.vi"("lines"=w98) -> ("task out"=w97:refnum<k21>)  [unwired: 13 in, 1 out]
  n1225 = call-poly <vilib>:"DAQmx Create Virtual Channel.vi"("lines"=w101) -> ("task out"=w100:refnum<k21>)  [unwired: 13 in, 1 out]
  n1226 = node-c288(2 ("Processor")) -> (w82:T14)  [unwired: 3 in]
  n1227 = timed-loop {
    timing: w82 -> [_]
    timing-out: [_] -> w81
    stop <- w1865 stop-if-true
    n1228 = node-c288() -> ()  [unwired: 1 in, 1 out]
    n1229 = case shown="\"Control\"" "Tab Control" {
      frame "Control" {
        n1230 = case shown="True" "Start" {
          frame False {
          }
          frame True {
            w1878 = T25 3 items=["no dialog", "OK message", "continue or stop message", "OK message + warnings", "continue/stop + warnings"] ("type of dialog (OK msg:1)")
            n1231 = call "InitializeAcquireFF.vi"("DAQ Rate"="DAQ Rate", "Averaging Number"="Averaging Number", "Sampling Rate"="Sampling Rate") -> ("error out"=w1872:errorcluster, "task out"=w1871:refnum<k21>, "Final Sampling Rate"=→"Final Sampling Rate":dbl)  [unwired: 4 in, 2 out]
            n1232 = while {
              tunnel: [w1890] -> w1877
              tunnel: [w1889] -> w1870
              tunnel: "Averaging Number" -> [w1888]
              tunnel: w1872 -> [w1887]
              tunnel: w1871 -> [w1885]
              stop <- w1886 continue-if-true
              n1233 = call "Acquire2_QPD.vi"("task/channels in"=w1885, "Save Data?"=FALSE ("Take Data?"), "Averaging Number"=w1888, "error in"=w1887) -> ("PSD 1"=→"PSD 1":cluster{dbl[], dbl[]}, "PSD 1 Sum"=→"PSD 1 Sum":dbl, "PSD 2"=→"PSD 2":cluster{dbl[], dbl[]}, "PSD 2 Sum"=→"PSD 2 Sum":dbl, "task out"=w1890:refnum<k21>, "error out"=w1889:errorcluster)  [unwired: 14 in, 4 out]
              n1234 = local read "Start"() -> (w1886:bool)
            }
            n1235 = call <vilib>:"DAQmx Clear Task.vi"("task in"=w1877, "error in"=w1870) -> ("error out"=w1879:errorcluster)  [unwired: 13 in]
            n1236 = call <vilib>:"Simple Error Handler.vi"("type of dialog (OK msg:1)"=w1878, "error in (no error)"=w1879) -> ()  [unwired: 3 in, 5 out]
          }
        }
      }
      frame "Current Saved Data" {
      }
      frame "Data Acquisition" {
      }
      frame "Raw QPD Data" {
      }
    }
    n1237 = local read "Stop"() -> (w1865:bool)
    n1238 = node-c288() -> ()  [unwired: 1 in, 1 out]
  }
  n1239 = node-c288(2 ("Processor")) -> (w34:T14)  [unwired: 3 in]
  n1240 = timed-loop {
    timing: w34 -> [_]
    timing-out: [_] -> w33
    stop <- w1891 stop-if-true
    n1241 = node-c288() -> ()  [unwired: 1 in, 1 out]
    n1242 = event shown="[0] \"Pause Mouse/Mirror Connection\": Value Change" {
      selector: _ -> [_ _]
      dyn-events: _ -> [_ _]
      timeout: _ -> [_ _]
      tunnel: [w1984 _] -> w1892
      tunnel: [_ w1985] -> w1891
      event "Pause Mouse/Mirror Connection": Value Change {
        n1243 = event-data() -> ("NewVal"=w1984:bool)  [unwired: 1 in]
      }
      event "Stop": Value Change {
        n1244 = event-data() -> ("NewVal"=w1985:bool)  [unwired: 1 in]
      }
    }
    n1245 = case shown="True" w1892 {
      frame False {
      }
      frame True {
        n1246 = call "InitializeMouseControl.vi"() -> ("error out 2"=w1901:errorcluster, "task out"=w1902:refnum<k21>, "error out"=w1904:errorcluster, "device ID"=w1903:refnum<k1>)  [unwired: 8 in]
        n1247 = while {
          tunnel: w1904 -> [w1916]
          tunnel: w1903 -> [w1915]
          tunnel: w1902 -> [w1914]
          tunnel: w1901 -> [w1913]
          tunnel: [w1912] -> w1899
          tunnel: [w1911] -> w1898
          tunnel: [w1910] -> w1895
          tunnel: [w1909] -> w1896
          stop <- w1908 stop-if-true
          n1248 = case shown="True" "Use Mouse to Move Trap?" {
            tunnel: w1915 -> [w1923 w1946]
            tunnel: w1916 -> [w1922 w1945]
            tunnel: w1914 -> [w1921 w1944]
            tunnel: w1913 -> [w1920 w1943]
            tunnel: [w1923 w1942] -> w1910
            tunnel: [w1922 w1941] -> w1909
            tunnel: [w1921 w1940] -> w1912
            tunnel: [w1920 w1939] -> w1911
            frame False {
              (unwired) FALSE ("button 1")
            }
            frame True {
              w1934 = 0.0 ("y")
              w1936 = 10
              n1249 = local read "Deflection"() -> (w1947:T6)
              n1250 = call-poly <vilib>:"Acquire Input Data.vi"("device ID"=w1946, "error in (no error)"=w1945) -> ("device ID"=w1942:refnum<k1>, "button info"=w1960:T26, "error out"=w1941:errorcluster)  [unwired: 14 in, 1 out]
              n1251 = Unbundle By Name(w1947) -> ("Horizontal"=w1949:i32, "Vertical"=w1948:i32)
              n1252 = local read "Saved voltage"() -> (w1925:cluster{dbl, dbl})
              n1253 = Divide(x=w1949, y=30) -> (x/y=w1952:dbl)
              n1254 = Divide(x=w1948, y=-20) -> (x/y=w1953:dbl)
              n1255 = Unbundle By Name(w1960) -> ("button 1"=w1938:bool, "button 2"=w1954:bool)
              n1256 = Bundle(w1952, w1953) -> (w1930:cluster{dbl, dbl})  [unwired: 1 in]
              n1257 = local write "Reference Voltage"(w1930) -> ()
              n1258 = Add(x=w1930, y=w1925) -> (x+y=w1958:cluster{dbl, dbl})
              n1259 = case shown="True" w1938 {
                frame False {
                  n1260 = stacked-sequence {
                    frame #0 {
                      n1261 = local write "CoordinatesMousePressed"(T6 {"Horizontal"=0, "Vertical"=0} ("Coords when pressed")) -> ()
                      n1262 = local write "Deflection"(T6 {"Horizontal"=0, "Vertical"=0} ("deflaction")) -> ()
                    }
                  }
                }
                frame True {
                  n1263 = local read "CoordinatesMousePressed"() -> (w1983:T6)
                  n1264 = local read "Real Coordinates"() -> (w1982:cluster{"Horizontal":i32, "Vertical":i32})
                  n1265 = Subtract(x=w1982, y=w1983) -> (x-y=w1981:T6)
                  n1266 = local write "Deflection"(w1981) -> ()
                }
              }
              n1267 = Unbundle(w1958) -> (w1935:dbl, w1926:dbl)
              n1268 = case shown="True" w1954 {
                frame False {
                }
                frame True {
                  n1269 = local read "Reference Voltage"() -> (w1964:cluster{dbl, dbl})
                  n1270 = local read "Saved voltage"() -> (w1962:cluster{dbl, dbl})
                  n1271 = Add(x=w1964, y=w1962) -> (x+y=→"Saved voltage":cluster{dbl, dbl})
                  n1272 = local read "Real Coordinates"() -> (w1963:cluster{"Horizontal":i32, "Vertical":i32})
                  n1273 = local write "CoordinatesMousePressed"(w1963) -> ()
                }
              }
              n1274 = Less?(x=w1935, y=w1936) -> (x < y?=w1933:bool)
              n1275 = Greater?(x=w1935, y=w1934) -> (0:w1932:bool)
              n1276 = Greater?(x=w1926, y=w1934) -> (0:w1928:bool)
              n1277 = Less?(x=w1926, y=w1936) -> (x < y?=w1929:bool)
              n1278 = And(x=w1928, y=w1929) -> (x .and. y?=w1927:bool)
              n1279 = And(x=w1933, y=w1932) -> (x .and. y?=w1931:bool)
              n1280 = case shown="False" w1927 {
                tunnel: [w1974 w1978] -> w1937
                tunnel: w1926 -> [w1972 w1978]
                frame False {
                  n1281 = Greater?(x=w1972, y=10.0) -> (0:w1975:bool)
                  n1282 = case shown="True" w1975 {
                    tunnel: [0.0 10.0] -> w1974
                    frame False {
                    }
                    frame True {
                    }
                  }
                }
                frame True {
                }
              }
              n1283 = case shown="False" w1931 {
                tunnel: w1935 -> [w1966 w1971]
                tunnel: [w1967 w1971] -> w1959
                frame False {
                  n1284 = Greater?(x=w1966, y=10.0) -> (0:w1968:bool)
                  n1285 = case shown="True" w1968 {
                    tunnel: [0.0 10.0] -> w1967
                    frame False {
                    }
                    frame True {
                    }
                  }
                }
                frame True {
                }
              }
              n1286 = Bundle(w1959, w1937) -> (w1924:cluster{dbl, dbl})  [unwired: 1 in]
              n1287 = Cluster To Array(cluster=w1924) -> (array=w1955:dbl[])
              n1288 = call-poly <vilib>:"DAQmx Write.vi"("task/channels in"=w1944, "data"=w1955, "error in"=w1943) -> ("task out"=w1957:refnum<k21>, "error out"=w1956:errorcluster)  [unwired: 10 in, 1 out]
              n1289 = call <vilib>:"DAQmx Is Task Done.vi"("task/channels in"=w1957, "error in"=w1956) -> ("task out"=w1940:refnum<k21>, "error out"=w1939:errorcluster)  [unwired: 11 in, 1 out]
            }
          }
          n1290 = event shown="[0] \"Pane\": Mouse Move" {
            selector: _ -> [_ _ _]
            dyn-events: _ -> [_ _ _]
            timeout: _ -> [_ _ _]
            event Mouse Move {
              n1291 = event-data() -> ("Coords"=w1918:T6)  [unwired: 1 in]
              n1292 = local write "Real Coordinates"(w1918) -> ()
            }
            event Mouse Down {
              n1293 = event-data() -> ("Coords"=w1919:T6)  [unwired: 1 in]
              n1294 = local write "CoordinatesMousePressed"(w1919) -> ()
            }
            event "Pause Mouse/Mirror Connection": Value Change {
              n1295 = event-data() -> ()  [unwired: 1 in, 3 out]
            }
          }
          n1296 = local read "Stop"() -> (w1905:bool)
          n1297 = Not(x="Pause Mouse/Mirror Connection") -> (.not. x?=w1906:bool)
          n1298 = Or(x=w1906, y=w1905) -> (x .or. y?=w1908:bool)
        }
        n1299 = call <vilib>:"DAQmx Clear Task.vi"("task in"=w1899, "error in"=w1898) -> ("error out"=w1900:errorcluster)  [unwired: 13 in]
        n1300 = call <vilib>:"Simple Error Handler.vi"("error in (no error)"=w1900) -> ()  [unwired: 4 in, 5 out]
        n1301 = call-poly <vilib>:"Close Input Device.vi"("error in (no error)"=w1896, "device ID"=w1895) -> ("error out"=w1897:errorcluster)  [unwired: 8 in]
        n1302 = call <vilib>:"Simple Error Handler.vi"("error in (no error)"=w1897) -> ()  [unwired: 4 in, 5 out]
      }
    }
    n1303 = node-c288() -> ()  [unwired: 1 in, 1 out]
  }
  n1304 = node-c288(i64 100 ("Period")) -> (w95:T14)  [unwired: 3 in]
  n1305 = timed-loop {
    tunnel: w97 -> [w1988]
    tunnel: [w1987] -> w96
    tunnel: w100 -> [w1990]
    tunnel: [w1989] -> w99
    timing: w95 -> [_]
    timing-out: [_] -> w94
    stop <- w1986 stop-if-true
    n1306 = node-c288() -> ()  [unwired: 1 in, 1 out]
    n1307 = event shown="[1] \"Shutter 2 (A)\": Value Change" {
      selector: _ -> [_ _ _]
      dyn-events: _ -> [_ _ _]
      timeout: _ -> [_ _ _]
      tunnel: w1990 -> [w1994 _ w2031]
      tunnel: [w1993 _ w2031] -> w1989
      tunnel: w1988 -> [_ w2014 w2032]
      tunnel: [_ w2012 w2032] -> w1987
      tunnel: [_ _ w2033] -> w1986
      event "Shutter 1 (B)": Value Change {
        n1308 = event-data() -> ()  [unwired: 1 in, 1 out]
        n1309 = flat-sequence {
          tunnel: [w2000] -> w1997
          tunnel: w1994 -> [w1999]
          tunnel: [w2004] -> w1996
          tunnel: [w2007] -> w1995
          tunnel: w1997 -> [w2002]
          tunnel: w1996 -> [w2011]
          tunnel: w1995 -> [w2009]
          tunnel: [w2008] -> w1993
          frame #0 {
            n1310 = call-poly <vilib>:"DAQmx Write.vi"("task/channels in"=w1999, "data"=FALSE) -> ("task out"=w2000:refnum<k21>)  [unwired: 11 in, 2 out]
            n1311 = Wait (ms)(milliseconds to wait=100) -> ()  [unwired: 1 out]
          }
          frame #1 {
            n1312 = Or(x="Shutter 1 (B)", y=TRUE) -> (x .or. y?=w2004:bool)
            n1313 = call-poly <vilib>:"DAQmx Write.vi"("task/channels in"=w2002, "data"=w2004) -> ("task out"=w2007:refnum<k21>)  [unwired: 11 in, 2 out]
            n1314 = Wait (ms)(milliseconds to wait=100) -> ()  [unwired: 1 out]
          }
          frame #2 {
            n1315 = Not(x=w2011) -> (.not. x?=w2010:bool)
            n1316 = call-poly <vilib>:"DAQmx Write.vi"("task/channels in"=w2009, "data"=w2010) -> ("task out"=w2008:refnum<k21>)  [unwired: 11 in, 2 out]
          }
        }
      }
      event "Shutter 2 (A)": Value Change {
        n1317 = event-data() -> ()  [unwired: 1 in, 1 out]
        n1318 = flat-sequence {
          tunnel: w2014 -> [w2019]
          tunnel: [w2018] -> w2013
          tunnel: [w2023] -> w2016
          tunnel: [w2026] -> w2015
          tunnel: w2013 -> [w2021]
          tunnel: w2016 -> [w2030]
          tunnel: w2015 -> [w2028]
          tunnel: [w2027] -> w2012
          frame #0 {
            n1319 = call-poly <vilib>:"DAQmx Write.vi"("task/channels in"=w2019, "data"=FALSE) -> ("task out"=w2018:refnum<k21>)  [unwired: 11 in, 2 out]
            n1320 = Wait (ms)(milliseconds to wait=100) -> ()  [unwired: 1 out]
          }
          frame #1 {
            n1321 = Or(x="Shutter 2 (A)", y=TRUE) -> (x .or. y?=w2023:bool)
            n1322 = call-poly <vilib>:"DAQmx Write.vi"("task/channels in"=w2021, "data"=w2023) -> ("task out"=w2026:refnum<k21>)  [unwired: 11 in, 2 out]
            n1323 = Wait (ms)(milliseconds to wait=100) -> ()  [unwired: 1 out]
          }
          frame #2 {
            n1324 = Not(x=w2030) -> (.not. x?=w2029:bool)
            n1325 = call-poly <vilib>:"DAQmx Write.vi"("task/channels in"=w2028, "data"=w2029) -> ("task out"=w2027:refnum<k21>)  [unwired: 11 in, 2 out]
          }
        }
      }
      event "Stop": Value Change {
        n1326 = event-data() -> ("NewVal"=w2033:bool)  [unwired: 1 in, 5 out]
      }
    }
    n1327 = node-c288() -> ()  [unwired: 1 in, 1 out]
  }
  n1328 = node-c288(w94) -> ()  [unwired: 1 out]
  n1329 = node-c288(w81) -> ()  [unwired: 1 out]
  n1330 = call <vilib>:"DAQmx Clear Task.vi"("task in"=w96) -> ()  [unwired: 14 in, 1 out]
  n1331 = call <vilib>:"DAQmx Clear Task.vi"("task in"=w99) -> ()  [unwired: 14 in, 1 out]
  n1332 = node-c288(w33) -> ()  [unwired: 1 out]
  n1333 = node-c288(w29) -> ()  [unwired: 1 out]
  n1334 = local write "Tether"(FALSE ("Tether")) -> ()
  n1335 = local read "Path"() -> (w88:path)
  n1336 = node-c288(i64 1 ("Period"), 2 ("Processor")) -> (w93:T14)  [unwired: 2 in]
  n1337 = timed-loop {
    timing: w93 -> [_]
    timing-out: [_] -> w92
    tunnel: w88 -> [w2035]
    stop <- w2034 stop-if-true
    n1338 = node-c288() -> ()  [unwired: 1 in, 1 out]
    n1339 = event shown="[3] \"reset offset ffb param\": Value Change" {
      selector: _ -> [_ _ _ _ _ _ _ _ _ _ _ _]
      dyn-events: _ -> [_ _ _ _ _ _ _ _ _ _ _ _]
      timeout: _ -> [_ _ _ _ _ _ _ _ _ _ _ _]
      tunnel: w2035 -> [_ w2039 w2078 _ _ _ _ _ _ _ _ _]
      tunnel: [_ _ _ _ w2084 _ _ _ _ _ _ _] -> w2034
      event Timeout {
        n1340 = event-data() -> ()  [unwired: 1 in, 2 out]
      }
      event "Read Cal": Value Change {
        n1341 = event-data() -> ()  [unwired: 1 in, 6 out]
        n1342 = Path To String(path=w2039) -> (string=w2038:string)
        n1343 = Format Date/Time String(time format string (%c)="%y%m%d") -> (date/time string=w2040:string)  [unwired: 2 in]
        n1344 = Concatenate Strings(w2038, "\\" ("string"), w2040, "\\" ("string"), "current.cal") -> (w2058:string)
        n1345 = String To Path(string=w2058) -> (path=w2057:path)
        n1346 = Open/Create/Replace File(file path (use dialog)=w2057, operation (0:open)=T19."open", access (0:read/write)=enum16{"read/write", "read-only", "write-only"}."read-only") -> (refnum out=w2053:refnum<file>, error out=w2054:errorcluster)  [unwired: 3 in, 1 out]
        n1347 = Deny Access(4:w2054, 7:w2053) -> (0:w2052:errorcluster, 3:w2051:refnum<file>)  [unwired: 1 in]
        n1348 = Read from Binary File(5:0.0, 8:w2052, 9:T20."big-endian, network order" ("byte order (0:big-endian, network order)"), 10:12 ("count"), 11:w2051) -> (0:w2047:errorcluster, 2:w2045:dbl[], 3:w2048:refnum<file>)  [unwired: 1 in, 1 out]
        n1349 = Array To Cluster(array=w2045) -> (cluster=→"Cal values":T27)
        n1350 = Close File(refnum=w2048, error in=w2047) -> ()  [unwired: 2 out]
        n1351 = local write "Read Cal"(FALSE ("Read Cal")) -> ()
      }
      event "Read \nOffset FFB param": Value Change {
        w2075 = "\\" ("string")
        n1352 = event-data() -> ()  [unwired: 1 in, 6 out]
        n1353 = Path To String(path=w2078) -> (string=w2077:string)
        n1354 = Format Date/Time String(time format string (%c)="%y%m%d") -> (date/time string=w2076:string)  [unwired: 2 in]
        n1355 = Concatenate Strings(w2077, w2075, w2076, w2075, "current.offsetffbparam" ("string")) -> (w2073:string)
        n1356 = String To Path(string=w2073) -> (path=w2072:path)
        n1357 = Open/Create/Replace File(file path (use dialog)=w2072, operation (0:open)=T19."open", access (0:read/write)=enum16{"read/write", "read-only", "write-only"}."read-only") -> (refnum out=w2069:refnum<file>, error out=w2068:errorcluster)  [unwired: 3 in, 1 out]
        n1358 = local write "Read \nOffset FFB param"(FALSE ("Read Cal")) -> ()
        n1359 = Deny Access(4:w2068, 7:w2069) -> (0:w2066:errorcluster, 3:w2067:refnum<file>)  [unwired: 1 in]
        n1360 = Read from Binary File(5:0.0, 8:w2066, 9:T20."big-endian, network order" ("byte order (0:big-endian, network order)"), 10:13 ("count (1)"), 11:w2067) -> (0:w2064:errorcluster, 2:w2061:dbl[], 3:w2065:refnum<file>)  [unwired: 1 in, 1 out]
        n1361 = Array To Cluster(array=w2061) -> (cluster=→"offset ffb param":T28)
        n1362 = Close File(refnum=w2065, error in=w2064) -> ()  [unwired: 2 out]
      }
      event "reset offset ffb param": Value Change {
        n1363 = event-data() -> ()  [unwired: 1 in, 6 out]
        n1364 = local write "reset offset ffb param"(FALSE ("reset offset ffb param")) -> ()
        n1365 = Array To Cluster(array=dbl[] []) -> (cluster=w2082:T29)
        n1366 = local write "offset ffb param"(w2082) -> ()
      }
      event "Stop": Value Change {
        n1367 = event-data() -> ("NewVal"=w2084:bool)  [unwired: 1 in, 5 out]
      }
      event "Trap position (V)": Value Change {
        # "Need to rotate so X and Y don't get mixed up."
        n1368 = event-data() -> ()  [unwired: 1 in, 6 out]
        n1369 = local read "Mirror task"() -> (w2085:refnum<k21>)
        n1370 = Cluster To Array(cluster="Trap position (V)") -> (array=w2088:dbl[])
        n1371 = Rotate 1D Array(1:w2088, 2:1 ("n")) -> (0:w2086:dbl[])
        n1372 = call-poly <vilib>:"DAQmx Write.vi"("task/channels in"=w2085, "data"=w2086) -> ("task out"=w2091:refnum<k21>, "error out"=w2090:errorcluster)  [unwired: 11 in, 1 out]
        n1373 = call <vilib>:"DAQmx Stop Task.vi"("task/channels in"=w2091, "error in"=w2090) -> ("error out"=w2089:errorcluster)  [unwired: 12 in, 1 out]
        n1374 = call <vilib>:"Simple Error Handler.vi"("error in (no error)"=w2089) -> ()  [unwired: 4 in, 5 out]
      }
      event "Trap delta (nm)": Value Change {
        n1375 = event-data() -> ()  [unwired: 1 in, 6 out]
        n1376 = local read "Pulling direction"() -> (w2093:bool)
        n1377 = local read "Conv Y (nm/V)"() -> (w2094:dbl)
        n1378 = local read "Conv X (nm/V)"() -> (w2095:dbl)
        n1379 = Select(t=w2094, s=w2093, f=w2095) -> (s? t:f=w2096:dbl)
        n1380 = local read "Fixed Y"() -> (w2102:dbl)
        n1381 = Divide(x="Trap delta (nm)", y=w2096) -> (x/y=w2097:dbl)
        n1382 = local read "Fixed X"() -> (w2101:dbl)
        n1383 = Select(t=w2102, s=w2093, f=w2101) -> (s? t:f=w2100:dbl)
        n1384 = Add(x=w2097, y=w2100) -> (x+y=w2098:dbl)
        n1385 = case shown="False" w2093 {
          tunnel: w2098 -> [w2103 w2104]
          frame False {
            n1386 = property on="X" class="DigNum (strict)"("Val(Sgnl)"=w2103) -> ()  [unwired: 2 in, 2 out]
          }
          frame True {
            n1387 = property on="Y" class="DigNum (strict)"("Val(Sgnl)"=w2104) -> ()  [unwired: 2 in, 2 out]
          }
        }
      }
      event "Fish": Value Change {
        n1388 = event-data() -> ()  [unwired: 1 in, 6 out]
        n1389 = local read "Fish"() -> (w2105:bool)
        n1390 = case shown="True" w2105 {
          frame False {
          }
          frame True {
            w2115 = 0.0 ("minimum value")
            w2116 = 10.0 ("maximum value")
            # "Grab offset in pulling\ndirection and add to \ndelta values"
            n1391 = call-poly <vilib>:"DAQmx Create Virtual Channel.vi"("maximum value"=w2116, "minimum value"=w2115, "physical channels"=tag "Dev1/ao0") -> ("task out"=w2120:refnum<k21>, "error out"=w2119:errorcluster)  [unwired: 11 in]
            n1392 = call-poly <vilib>:"DAQmx Create Virtual Channel.vi"("task in"=w2120, "maximum value"=w2116, "minimum value"=w2115, "physical channels"=tag "Dev1/ao1", "error in"=w2119) -> ("task out"=w2114:refnum<k21>, "error out"=w2113:errorcluster)  [unwired: 9 in]
            n1393 = node-c288(i64 1 ("Period")) -> (w2122:T14)  [unwired: 3 in]
            n1394 = timed-loop {
              timing: w2122 -> [_]
              timing-out: [_] -> w2121
              tunnel: w2114 -> [w2191]
              tunnel: w2113 -> [w2190]
              tunnel: [w2189] -> w2110
              tunnel: [w2188] -> w2109
              tunnel: [w2148] -> w2111
              tunnel: [w2149] -> w2108
              i -> [w2174]
              stop <- w2149 stop-if-true
              # "x direction"
              # "y direction"
              # "Send offset in direction\nof not-pulling to DAQ"
              n1395 = node-c288() -> ()  [unwired: 1 in, 1 out]
              n1396 = local read "Pulling direction"() -> (w2153:bool)
              n1397 = local read "Conv Y (nm/V)"() -> (w2155:dbl)
              n1398 = local read "Conv X (nm/V)"() -> (w2154:dbl)
              n1399 = local read "Fixed X"() -> (w2162:dbl)
              n1400 = local read "Fixed Y"() -> (w2161:dbl)
              n1401 = Select(t=w2161, s=w2153, f=w2162) -> (s? t:f=w2163:dbl)
              n1402 = Select(t=w2162, s=w2153, f=w2161) -> (s? t:f=w2160:dbl)
              n1403 = Select(t=w2155, s=w2153, f=w2154) -> (s? t:f=w2150:dbl)
              n1404 = Divide(x="Max fish\ndelta (nm)", y=w2150) -> (x/y=w2152:dbl)
              n1405 = Divide(x="Min fish\ndelta (nm)", y=w2150) -> (x/y=w2151:dbl)
              n1406 = Add(x=w2163, y=w2152) -> (x+y=w2165:dbl)
              n1407 = Subtract(x=w2152, y=w2151) -> (x-y=w2167:dbl)
              n1408 = Divide(x=w2167, y="Fish Speed (ms)") -> (x/y=w2168:dbl)
              n1409 = flat-sequence {
                tunnel: w2153 -> [w2211]
                tunnel: w2160 -> [w2210]
                tunnel: w2191 -> [w2209]
                tunnel: w2190 -> [w2208]
                tunnel: w2168 -> [w2207]
                tunnel: w2165 -> [w2206]
                tunnel: "Fish Speed (ms)" -> [w2201]
                tunnel: [w2205] -> w2187
                tunnel: [w2204] -> w2186
                tunnel: [w2203] -> w2185
                tunnel: [w2202] -> w2184
                tunnel: [w2195] -> w2173
                tunnel: [w2194] -> w2159
                tunnel: [w2193] -> w2156
                tunnel: [w2192] -> w2146
                tunnel: [w2264] -> w2183
                tunnel: w2187 -> [w2264]
                tunnel: [w2263] -> w2182
                tunnel: w2186 -> [w2263]
                tunnel: [w2262] -> w2181
                tunnel: w2185 -> [w2262]
                tunnel: [w2261] -> w2180
                tunnel: w2184 -> [w2261]
                tunnel: w2173 -> [w2260]
                tunnel: [w2260] -> w2172
                tunnel: w2159 -> [w2259]
                tunnel: [w2258] -> w2157
                tunnel: w2156 -> [w2258]
                tunnel: [w2257] -> w2147
                tunnel: w2146 -> [w2257]
                tunnel: w2183 -> [w2276]
                tunnel: w2182 -> [w2275]
                tunnel: w2181 -> [w2274]
                tunnel: w2180 -> [w2273]
                tunnel: w2170 -> [w2272]
                tunnel: [w2271] -> w2189
                tunnel: [w2270] -> w2188
                tunnel: w2172 -> [w2269]
                tunnel: [w2268] -> w2158
                tunnel: w2157 -> [w2267]
                tunnel: [w2266] -> w2145
                tunnel: w2147 -> [w2266]
                frame #0 {
                  n1410 = local read "Mean force (pN)"() -> (w2200:dbl)
                  n1411 = local read "Cutoff force (pN)"() -> (w2199:dbl)
                  n1412 = Less Or Equal?(x=w2200, y=w2199) -> (x <= y?=w2197:bool)
                  n1413 = And(x="Fish", y=w2197) -> (x .and. y?=w2198:bool)
                  n1414 = case shown="True" w2198 {
                    selector: w2198 -> [w2214 _]
                    tunnel: w2211 -> [w2217 w2234]
                    tunnel: w2210 -> [_ w2233]
                    tunnel: w2209 -> [w2219 w2232]
                    tunnel: w2208 -> [w2218 w2231]
                    tunnel: w2207 -> [w2216 w2230]
                    tunnel: w2206 -> [w2215 w2229]
                    tunnel: [w2219 w2228] -> w2205
                    tunnel: [w2218 w2227] -> w2204
                    tunnel: [w2217 w2226] -> w2203
                    tunnel: [w2215 w2225] -> w2193
                    tunnel: [w2216 w2224] -> w2202
                    tunnel: w2201 -> [_ w2223]
                    tunnel: [w2214 w2222] -> w2195
                    tunnel: [FALSE w2221] -> w2194
                    tunnel: [FALSE w2220] -> w2192
                    frame False {
                    }
                    frame True {
                      n1415 = while {
                        tunnel: w2234 -> [w2246]
                        tunnel: w2233 -> [w2245]
                        tunnel: w2232 -> [w2253]
                        tunnel: w2231 -> [w2252]
                        tunnel: w2230 -> [w2244]
                        tunnel: w2229 -> [w2250]
                        tunnel: [w2248] -> w2228
                        tunnel: [w2247] -> w2227
                        tunnel: [w2246] -> w2226
                        tunnel: [w2245] -> w2225
                        tunnel: [w2244] -> w2224
                        tunnel: w2223 -> [w2243]
                        tunnel: [w2236] -> w2222
                        tunnel: [w2236] -> w2221
                        tunnel: [w2235] -> w2220
                        i -> [w2242]
                        stop <- w2239 stop-if-true
                        # "top: x"
                        # "x direction"
                        # "y direction"
                        n1416 = Multiply(x=w2244, y=w2242) -> (x*y=w2251:dbl)
                        n1417 = local read "Cutoff force (pN)"() -> (w2237:dbl)
                        n1418 = local read "Mean force (pN)"() -> (w2238:dbl)
                        n1419 = Subtract(x=w2250, y=w2251) -> (x-y=w2249:dbl)
                        n1420 = Build Array(w2245, w2249) -> (w2256:dbl[])
                        n1421 = Build Array(w2249, w2245) -> (w2255:dbl[])
                        n1422 = Greater Or Equal?(x=w2242, y=w2243) -> (x >= y?=w2236:bool)
                        n1423 = Select(t=w2256, s=w2246, f=w2255) -> (s? t:f=w2254:dbl[])
                        n1424 = Greater?(x=w2238, y=w2237) -> (0:w2235:bool)
                        n1425 = local read "Fish"() -> (w2240:bool)
                        n1426 = Not(x=w2240) -> (.not. x?=w2241:bool)
                        n1427 = call-poly <vilib>:"DAQmx Write.vi"("task/channels in"=w2253, "data"=w2254, "error in"=w2252) -> ("task out"=w2248:refnum<k21>, "error out"=w2247:errorcluster)  [unwired: 10 in, 1 out]
                        n1428 = Compound Arithmetic op=OR(w2236, w2241, w2235) -> (w2239:bool)
                      }
                    }
                  }
                }
                frame #1 {
                  n1429 = case shown="True" w2259 {
                    frame False {
                    }
                    frame True {
                      n1430 = Wait (ms)(milliseconds to wait="Wait (ms)") -> ()  [unwired: 1 out]
                    }
                  }
                }
                frame #2 {
                  n1431 = case shown="True" w2269 {
                    tunnel: w2276 -> [w2279 w2288]
                    tunnel: w2275 -> [w2278 w2287]
                    tunnel: w2274 -> [_ w2286]
                    tunnel: w2273 -> [_ w2285]
                    tunnel: w2272 -> [_ w2284]
                    tunnel: [w2279 w2283] -> w2271
                    tunnel: [w2278 w2282] -> w2270
                    tunnel: [FALSE w2281] -> w2268
                    tunnel: w2267 -> [_ w2280]
                    frame False {
                    }
                    frame True {
                      n1432 = while {
                        tunnel: w2288 -> [w2320]
                        tunnel: w2287 -> [w2319]
                        tunnel: w2286 -> [w2291]
                        tunnel: w2285 -> [w2317]
                        tunnel: w2284 -> [w2316]
                        tunnel: [w2314] -> w2283
                        tunnel: [w2313] -> w2282
                        tunnel: [w2298] -> w2281
                        tunnel: w2280 -> [w2289]
                        i -> [w2305]
                        stop <- w2310 stop-if-true
                        # "y direction"
                        # "If tether formed,\nimmediately change\nto new delta."
                        n1433 = local read "Conv Y (nm/V)"() -> (w2292:dbl)
                        n1434 = local read "Conv X (nm/V)"() -> (w2290:dbl)
                        n1435 = local read "Fixed Y"() -> (w2299:dbl)
                        n1436 = local read "Fixed X"() -> (w2304:dbl)
                        n1437 = Select(t=w2292, s=w2291, f=w2290) -> (s? t:f=w2293:dbl)
                        n1438 = local read "Cutoff force (pN)"() -> (w2306:dbl)
                        n1439 = Divide(x="Delta after tether", y=w2293) -> (x/y=w2294:dbl)
                        n1440 = Multiply(x=w2317, y=w2305) -> (x*y=w2318:dbl)
                        n1441 = local read "Mean force (pN)"() -> (w2307:dbl)
                        n1442 = Add(x=w2316, y=w2318) -> (x+y=w2301:dbl)
                        n1443 = Select(t=w2299, s=w2291, f=w2304) -> (s? t:f=w2303:dbl)
                        n1444 = Greater?(x=w2307, y=w2306) -> (0:w2298:bool)
                        n1445 = Add(x=w2303, y=w2294) -> (x+y=w2302:dbl)
                        n1446 = Select(t=w2302, s=w2298, f=w2301) -> (s? t:f=w2300:dbl)
                        n1447 = local read "Fish Speed (ms)"() -> (w2312:i32)
                        n1448 = Build Array(w2289, w2300) -> (w2315:dbl[])
                        n1449 = Build Array(w2300, w2289) -> (w2296:dbl[])
                        n1450 = Select(t=w2315, s=w2291, f=w2296) -> (s? t:f=w2295:dbl[])
                        n1451 = case shown="True" w2298 {
                          tunnel: w2294 -> [_ _]
                          tunnel: w2295 -> [_ w2322]
                          frame False {
                          }
                          frame True {
                            n1452 = Array To Cluster(array=w2322) -> (cluster=w2321:cluster{"[0]":dbl, "[1]":dbl})
                            n1453 = property on="Trap position (V)" class="Clust (strict)"("Val(Sgnl)"=w2321) -> ()  [unwired: 2 in, 2 out]
                          }
                        }
                        n1454 = local read "Fish"() -> (w2309:bool)
                        n1455 = Greater Or Equal?(x=w2305, y=w2312) -> (x >= y?=w2311:bool)
                        n1456 = Not(x=w2309) -> (.not. x?=w2308:bool)
                        n1457 = call-poly <vilib>:"DAQmx Write.vi"("task/channels in"=w2320, "data"=w2295, "error in"=w2319) -> ("task out"=w2314:refnum<k21>, "error out"=w2313:errorcluster)  [unwired: 10 in, 1 out]
                        n1458 = Compound Arithmetic op=OR(w2311, w2308, w2298) -> (w2310:bool)
                      }
                    }
                  }
                }
              }
              n1459 = Add(x=w2163, y=w2151) -> (x+y=w2170:dbl)
              n1460 = Decrement(x="# attempts") -> (x-1=w2178:dbl)
              n1461 = Greater Or Equal?(x=w2174, y=w2178) -> (x >= y?=w2177:bool)
              n1462 = local read "Mean force (pN)"() -> (w2176:dbl)
              n1463 = Greater?(x=w2176, y="Cutoff force (pN)") -> (0:w2171:bool)
              n1464 = Compound Arithmetic op=OR(w2145, w2158, w2171, w2177) -> (w2149:bool)
              n1465 = Or(x=w2158, y=w2145) -> (x .or. y?=w2148:bool)
              "Tether" <- w2148
              n1466 = case shown="True" w2148 {
                frame False {
                }
                frame True {
                  n1467 = call <vilib>:"Beep.vi"() -> ()  [unwired: 12 in]
                }
              }
              n1468 = node-c288() -> ()  [unwired: 1 in, 1 out]
              "Attempt #" <- w2174
            }
            n1469 = node-c288(w2121) -> ()  [unwired: 1 out]
            n1470 = flat-sequence {
              tunnel: w2111 -> [w2129]
              tunnel: [w2129] -> w2107
              tunnel: w2110 -> [w2126]
              tunnel: w2109 -> [w2125]
              tunnel: w2108 -> [w2123]
              tunnel: w2107 -> [w2131]
              tunnel: [w2131] -> w2106
              tunnel: w2106 -> [w2133]
              frame #0 {
                w2128 = T25 1 items=["no dialog", "OK message", "continue or stop message", "OK message + warnings", "continue/stop + warnings"] ("type of dialog (OK msg:1)")
                n1471 = call <vilib>:"DAQmx Clear Task.vi"("task in"=w2126, "error in"=w2125) -> ("error out"=w2127:errorcluster)  [unwired: 13 in]
                n1472 = Not(x=w2123) -> (.not. x?=w2124:bool)
                n1473 = local write "Fish"(w2124) -> ()
                n1474 = call <vilib>:"Simple Error Handler.vi"("type of dialog (OK msg:1)"=w2128, "error in (no error)"=w2127) -> ()  [unwired: 3 in, 5 out]
              }
              frame #1 {
                n1475 = Wait (ms)(milliseconds to wait=u32 500) -> ()  [unwired: 1 out]
              }
              frame #2 {
                n1476 = And(x=w2133, y="Raster after\n tether?") -> (x .and. y?=w2134:bool)
                n1477 = case shown="True" w2134 {
                  selector: w2134 -> [_ w2135]
                  frame False {
                  }
                  frame True {
                    n1478 = stacked-sequence {
                      tunnel: w2135 -> [_ _ _ _ w2144]
                      frame #0 {
                        n1479 = local read "Raster set"() -> (w2139:i32)
                        n1480 = property on="Inject Sample" class="Bool (strict)"("Val(Sgnl)"=FALSE ("Value (Signaling)")) -> ()  [unwired: 2 in, 2 out]
                        n1481 = Replace Array Subset(array=i32[] [0], new element=w2139, index=0) -> (w2136:i32[])
                        n1482 = property on="Scan Parameters" class="Arr (strict)"("Index Values"=w2136) -> ()  [unwired: 2 in, 2 out]
                      }
                      frame #1 {
                        n1483 = Wait (ms)(milliseconds to wait=u32 500) -> ()  [unwired: 1 out]
                      }
                      frame #2 {
                        n1484 = property on="Load param" class="Bool (strict)"("Val(Sgnl)"=TRUE ("Value (Signaling)")) -> ()  [unwired: 2 in, 2 out]
                      }
                      frame #3 {
                        n1485 = Wait (ms)(milliseconds to wait=u32 500) -> ()  [unwired: 1 out]
                      }
                      frame #4 {
                        n1486 = property on="Raster scan" class="Bool (strict)"("Val(Sgnl)"=w2144) -> ()  [unwired: 2 in, 2 out]
                      }
                    }
                  }
                }
              }
            }
          }
        }
      }
      event "Load param": Value Change {
        n1487 = event-data() -> ()  [unwired: 1 in, 6 out]
        n1488 = property on="Scan Parameters" class="Arr (strict)"() -> ("Index Values"=w2338:u32[])  [unwired: 2 in, 2 out]
        n1489 = Index Array(array=w2338, index=0) -> (element=w2335:u32)
        n1490 = Index Array(array="Scan Parameters", index=w2335) -> (element=w2334:T30)
        n1491 = Unbundle(w2334) -> ("Scan range 1"=w2332:dbl, "Step size 1"=w2331:dbl, "Scan speed 1"=w2329:i32, "# scans 2"=w2330:i32)  [unwired: 1 out]
        n1492 = property on="# scans" class="DigNum (strict)"("Val(Sgnl)"=w2330) -> ()  [unwired: 2 in, 2 out]
        n1493 = property on="Scan range (nm)" class="DigNum (strict)"("Val(Sgnl)"=w2332) -> ()  [unwired: 2 in, 2 out]
        n1494 = property on="Step size 1" class="DigNum (strict)"("Val(Sgnl)"=w2331) -> ()  [unwired: 2 in, 2 out]
        n1495 = property on="Scan speed (nm/s)" class="DigNum (strict)"("Val(Sgnl)"=w2329) -> ()  [unwired: 2 in, 2 out]
        n1496 = local write "Load param"(FALSE ("Load param")) -> ()
      }
      event "# scans", "Scan range (nm)", "Step size (nm)", "Scan speed (nm/s)": Value Change {
        n1497 = event-data() -> ()  [unwired: 1 in, 6 out]
        n1498 = local read "Pulling direction"() -> (w2369:bool)
        n1499 = Reciprocal(x="Scan speed (nm/s)") -> (1/x=w2361:dbl)
        n1500 = local read "Conv Y (nm/V)"() -> (w2367:dbl)
        n1501 = local read "Conv X (nm/V)"() -> (w2368:dbl)
        n1502 = Multiply(x="Step size (nm)", y=w2361) -> (x*y=w2359:dbl)
        n1503 = Divide(x="Scan range (nm)", y="Step size (nm)") -> (x/y=w2366:dbl)
        n1504 = Absolute Value(x=w2366) -> (abs(x)=w2365:dbl)
        n1505 = Multiply(x=w2359, y=1000.0) -> (x*y=w2346:dbl)
        n1506 = Select(t=w2367, s=w2369, f=w2368) -> (s? t:f=w2357:dbl)
        n1507 = Multiply(x="# scans", y=2) -> (x*y=w2345:i32)
        n1508 = To Unsigned Quad Integer(1:w2365) -> (0:w2355:u64)
        "Scan steps (mirror)" <- w2355
        n1509 = Divide(x="Scan range (nm)", y=w2357) -> (x/y=→"Scan range (V)":dbl)
        n1510 = Multiply(x=w2355, y=w2346) -> (x*y=w2354:dbl)
        n1511 = Divide(x="Step size (nm)", y=w2357) -> (x/y=→"Scan increment (V)":dbl)
        n1512 = Round Toward +Infinity(x=w2346) -> (ceil(x): smallest int >= x=w2343:dbl)
        "Time per step (ms)" <- w2343
        n1513 = local read "Data update period (s/set)"() -> (w2349:dbl)
        n1514 = Multiply(x=w2345, y=w2354) -> (x*y=w2352:dbl)
        n1515 = Divide(x=w2352, y=1000.0) -> (x/y=w2350:dbl)
        "Total raster time (s)" <- w2350
        n1516 = local read "Data update period (s/set)"() -> (w2341:dbl)
        n1517 = Divide(x=w2350, y=w2349) -> (x/y=w2348:dbl)
        n1518 = Round Toward -Infinity(1:w2348) -> (0:→"N sets to be saved":dbl)
        n1519 = Multiply(x=w2341, y=1000.0) -> (x*y=w2339:dbl)
        n1520 = Less?(x=w2343, y=w2339) -> (x < y?=w2342:bool)
        n1521 = case shown="True" w2342 {
          selector: w2342 -> [_ w2370]
          frame False {
          }
          frame True {
            n1522 = call "Display Message to User"("Enable"=w2370) -> ()  [unwired: 9 in, 2 out]
          }
        }
      }
      event "Pulling direction": Value Change {
        n1523 = event-data() -> ()  [unwired: 1 in, 6 out]
        n1524 = local read "Pulling direction"() -> (w2376:bool)
        n1525 = local read "Conv Y (nm/V)"() -> (w2378:dbl)
        n1526 = local read "Conv X (nm/V)"() -> (w2377:dbl)
        n1527 = local read "Scan range (nm)"() -> (w2375:dbl)
        n1528 = Select(t=w2378, s=w2376, f=w2377) -> (s? t:f=w2372:dbl)
        n1529 = local read "Step size (nm)"() -> (w2373:dbl)
        n1530 = case shown="False" w2376 {
          frame False {
            n1531 = local read "Fixed Y"() -> (w2381:dbl)
            n1532 = local read "Trap delta (nm)"() -> (w2386:dbl)
            n1533 = local read "Conv X (nm/V)"() -> (w2385:dbl)
            n1534 = local read "Fixed X"() -> (w2383:dbl)
            n1535 = Divide(x=w2386, y=w2385) -> (x/y=w2384:dbl)
            n1536 = Add(x=w2384, y=w2383) -> (x+y=w2382:dbl)
            n1537 = Build Array(w2382, w2381) -> (w2380:dbl[])
            n1538 = Array To Cluster(array=w2380) -> (cluster=w2379:cluster{"[0]":dbl, "[1]":dbl})
            n1539 = property on="Trap position (V)" class="Clust (strict)"("Val(Sgnl)"=w2379) -> ()  [unwired: 2 in, 2 out]
          }
          frame True {
            n1540 = local read "Trap delta (nm)"() -> (w2394:dbl)
            n1541 = local read "Conv Y (nm/V)"() -> (w2393:dbl)
            n1542 = local read "Fixed X"() -> (w2389:dbl)
            n1543 = local read "Fixed Y"() -> (w2391:dbl)
            n1544 = Divide(x=w2394, y=w2393) -> (x/y=w2392:dbl)
            n1545 = Add(x=w2392, y=w2391) -> (x+y=w2390:dbl)
            n1546 = Build Array(w2389, w2390) -> (w2388:dbl[])
            n1547 = Array To Cluster(array=w2388) -> (cluster=w2387:cluster{"[0]":dbl, "[1]":dbl})
            n1548 = property on="Trap position (V)" class="Clust (strict)"("Val(Sgnl)"=w2387) -> ()  [unwired: 2 in, 2 out]
          }
        }
        n1549 = Divide(x=w2375, y=w2372) -> (x/y=w2374:dbl)
        n1550 = Divide(x=w2373, y=w2372) -> (x/y=w2371:dbl)
        n1551 = local write "Scan range (V)"(w2374) -> ()
        n1552 = local write "Scan increment (V)"(w2371) -> ()
      }
      event "Averaging Number": Value Change {
        n1553 = event-data() -> ()  [unwired: 1 in, 6 out]
        n1554 = local read "# Samples/channel (in)"() -> (w2398:i32)
        n1555 = local read "Averaging Number"() -> (w2396:i32)
        n1556 = Quotient & Remainder(x=w2398, y=w2396) -> (floor(x/y)=w2397:i32)  [unwired: 1 out]
        n1557 = Multiply(x=w2397, y=w2396) -> (x*y=w2395:i32)
        n1558 = local write "# Samples/channel (in)"(w2395) -> ()
      }
    }
    n1559 = node-c288() -> ()  [unwired: 1 in, 1 out]
  }
  n1560 = VISA Close(VISA resource name=w27) -> (error out=w105:errorcluster)  [unwired: 1 in]
  n1561 = call <vilib>:"Simple Error Handler.vi"("error in (no error)"=w105) -> ()  [unwired: 4 in, 5 out]
  n1562 = disable-structure shown="Enabled" {
    frame Disabled {
      n1563 = node-c288(2 ("Processor")) -> (w2404:T14)  [unwired: 3 in]
      n1564 = timed-loop "Pump Control" {
        timing: w2404 -> [_]
        timing-out: [_] -> w2403
        tunnel: refnum<visa-resource-name> "COM6" ("VISA resource name") -> [w2406]
        stop <- w2405 stop-if-true
        n1565 = node-c288() -> ()  [unwired: 1 in, 1 out]
        n1566 = event shown="[2] \"Stop\": Value Change" {
          selector: _ -> [_ _ _ _ _ _ _ _ _]
          dyn-events: _ -> [_ _ _ _ _ _ _ _ _]
          timeout: _ -> [_ _ _ _ _ _ _ _ _]
          tunnel: w2406 -> [w2414 w2510 _ w2586 w2714 w2857 w2902 w2960 w3019]
          tunnel: [_ _ w2585 _ _ _ _ _ _] -> w2405
          event "Flush Pump 1": Value Change {
            w2415 = "\r"
            n1567 = event-data() -> ()  [unwired: 1 in, 5 out]
            n1568 = call-poly "VISA Configure Serial Port"("VISA resource name"=w2414) -> ("VISA resource name out"=w2428:refnum<visa-resource-name>, "error out"=w2429:errorcluster)  [unwired: 13 in]
            n1569 = local read "Write Wait"() -> (w2407:i32)
            n1570 = Concatenate Strings("enter pump1", w2415) -> (w2416:string)
            n1571 = flat-sequence {
              tunnel: w2429 -> [w2448]
              tunnel: w2428 -> [w2450]
              tunnel: [w2449] -> w2445
              tunnel: [w2447] -> w2444
              tunnel: w2416 -> [w2446]
              tunnel: w2445 -> [w2453]
              tunnel: [w2453] -> w2443
              tunnel: w2444 -> [w2452]
              tunnel: [w2452] -> w2442
              tunnel: w2407 -> [w2451]
              tunnel: [w2458] -> w2441
              tunnel: w2421 -> [w2457]
              tunnel: [w2454] -> w2440
              tunnel: w2443 -> [w2456]
              tunnel: w2442 -> [w2455]
              tunnel: w2441 -> [w2461]
              tunnel: [w2461] -> w2439
              tunnel: [w2460] -> w2438
              tunnel: w2440 -> [w2460]
              tunnel: w2407 -> [w2459]
              tunnel: w2439 -> [w2466]
              tunnel: [w2465] -> w2437
              tunnel: w2424 -> [w2464]
              tunnel: w2438 -> [w2463]
              tunnel: [w2462] -> w2436
              tunnel: w2437 -> [w2469]
              tunnel: [w2469] -> w2435
              tunnel: [w2468] -> w2434
              tunnel: w2436 -> [w2468]
              tunnel: w2407 -> [w2467]
              tunnel: w2435 -> [w2474]
              tunnel: [w2473] -> w2433
              tunnel: w2427 -> [w2472]
              tunnel: w2434 -> [w2471]
              tunnel: [w2470] -> w2432
              tunnel: [w2477] -> w2431
              tunnel: w2433 -> [w2477]
              tunnel: [w2476] -> w2430
              tunnel: w2432 -> [w2476]
              tunnel: w2407 -> [w2475]
              tunnel: w2431 -> [w2482]
              tunnel: w2430 -> [w2479]
              tunnel: [w2481] -> w2410
              tunnel: [w2480] -> w2408
              tunnel: [w2487] -> w2411
              tunnel: w2410 -> [w2487]
              tunnel: [w2486] -> w2409
              tunnel: w2408 -> [w2486]
              tunnel: w2407 -> [w2485]
              tunnel: w2411 -> [w2489]
              tunnel: w2409 -> [w2488]
              frame #0 {
                n1572 = VISA Write(VISA resource name=w2450, write buffer=w2446, error in (no error)=w2448) -> (VISA resource name out=w2449:refnum<visa-resource-name>, error out=w2447:errorcluster)  [unwired: 1 out]
              }
              frame #1 {
                n1573 = Wait (ms)(milliseconds to wait=w2451) -> ()  [unwired: 1 out]
              }
              frame #2 {
                n1574 = VISA Write(VISA resource name=w2456, write buffer=w2457, error in (no error)=w2455) -> (VISA resource name out=w2458:refnum<visa-resource-name>, error out=w2454:errorcluster)  [unwired: 1 out]
              }
              frame #3 {
                n1575 = Wait (ms)(milliseconds to wait=w2459) -> ()  [unwired: 1 out]
              }
              frame #4 {
                n1576 = VISA Write(VISA resource name=w2466, write buffer=w2464, error in (no error)=w2463) -> (VISA resource name out=w2465:refnum<visa-resource-name>, error out=w2462:errorcluster)  [unwired: 1 out]
              }
              frame #5 {
                n1577 = Wait (ms)(milliseconds to wait=w2467) -> ()  [unwired: 1 out]
              }
              frame #6 {
                n1578 = VISA Write(VISA resource name=w2474, write buffer=w2472, error in (no error)=w2471) -> (VISA resource name out=w2473:refnum<visa-resource-name>, error out=w2470:errorcluster)  [unwired: 1 out]
              }
              frame #7 {
                n1579 = Wait (ms)(milliseconds to wait=w2475) -> ()  [unwired: 1 out]
              }
              frame #8 {
                n1580 = Concatenate Strings("start ", "\r") -> (w2478:string)
                n1581 = VISA Write(VISA resource name=w2482, write buffer=w2478, error in (no error)=w2479) -> (VISA resource name out=w2481:refnum<visa-resource-name>, error out=w2480:errorcluster)  [unwired: 1 out]
              }
              frame #9 {
                n1582 = Wait (ms)(milliseconds to wait=w2485) -> ()  [unwired: 1 out]
              }
              frame #10 {
                n1583 = local write "Flush Pump 1"(FALSE ("Flush Pump 1")) -> ()
                n1584 = Concatenate Strings("enter main ", "\r") -> (w2493:string)
                n1585 = VISA Write(VISA resource name=w2489, write buffer=w2493, error in (no error)=w2488) -> (VISA resource name out=w2492:refnum<visa-resource-name>, error out=w2491:errorcluster)  [unwired: 1 out]
                n1586 = VISA Close(VISA resource name=w2492, error in (no error)=w2491) -> ()  [unwired: 1 out]
              }
            }
            n1587 = Concatenate Strings("set units 4 ", w2415) -> (w2421:string)
            n1588 = Multiply(x="Flush\nRate (ul/min)", y=60) -> (x*y=w2419:dbl)
            n1589 = Number To Decimal String(number=w2419) -> (decimal integer string=w2422:string)  [unwired: 1 in]
            n1590 = Concatenate Strings("set rate ", w2422, w2415) -> (w2424:string)
            n1591 = Number To Decimal String(number="Flush\nVolume (ul)") -> (decimal integer string=w2426:string)  [unwired: 1 in]
            n1592 = Concatenate Strings("set volume ", w2426, w2415) -> (w2427:string)
          }
          event "Flush Pump 2": Value Change {
            w2501 = "\r"
            n1593 = event-data() -> ()  [unwired: 1 in, 5 out]
            n1594 = call-poly "VISA Configure Serial Port"("VISA resource name"=w2510) -> ("VISA resource name out"=w2521:refnum<visa-resource-name>, "error out"=w2522:errorcluster)  [unwired: 13 in]
            n1595 = local read "Write Wait"() -> (w2496:i32)
            n1596 = Concatenate Strings("enter pump2", w2501) -> (w2502:string)
            n1597 = flat-sequence {
              tunnel: w2522 -> [w2537]
              tunnel: w2521 -> [w2539]
              tunnel: [w2538] -> w2507
              tunnel: [w2536] -> w2505
              tunnel: w2502 -> [w2535]
              tunnel: w2507 -> [w2542]
              tunnel: [w2542] -> w2506
              tunnel: w2505 -> [w2541]
              tunnel: [w2541] -> w2504
              tunnel: w2496 -> [w2540]
              tunnel: [w2547] -> w2534
              tunnel: w2514 -> [w2546]
              tunnel: [w2543] -> w2533
              tunnel: w2506 -> [w2545]
              tunnel: w2504 -> [w2544]
              tunnel: w2534 -> [w2550]
              tunnel: [w2550] -> w2532
              tunnel: [w2549] -> w2531
              tunnel: w2533 -> [w2549]
              tunnel: w2496 -> [w2548]
              tunnel: w2532 -> [w2555]
              tunnel: [w2554] -> w2530
              tunnel: w2517 -> [w2553]
              tunnel: w2531 -> [w2552]
              tunnel: [w2551] -> w2529
              tunnel: w2530 -> [w2558]
              tunnel: [w2558] -> w2528
              tunnel: [w2557] -> w2527
              tunnel: w2529 -> [w2557]
              tunnel: w2496 -> [w2556]
              tunnel: w2528 -> [w2563]
              tunnel: [w2562] -> w2526
              tunnel: w2520 -> [w2561]
              tunnel: w2527 -> [w2560]
              tunnel: [w2559] -> w2525
              tunnel: [w2566] -> w2524
              tunnel: w2526 -> [w2566]
              tunnel: [w2565] -> w2523
              tunnel: w2525 -> [w2565]
              tunnel: w2496 -> [w2564]
              tunnel: w2524 -> [w2573]
              tunnel: w2523 -> [w2572]
              tunnel: [w2568] -> w2500
              tunnel: [w2567] -> w2498
              tunnel: w2500 -> [w2576]
              tunnel: [w2576] -> w2499
              tunnel: w2498 -> [w2575]
              tunnel: [w2575] -> w2497
              tunnel: w2496 -> [w2574]
              tunnel: w2499 -> [w2580]
              tunnel: w2497 -> [w2579]
              frame #0 {
                n1598 = VISA Write(VISA resource name=w2539, write buffer=w2535, error in (no error)=w2537) -> (VISA resource name out=w2538:refnum<visa-resource-name>, error out=w2536:errorcluster)  [unwired: 1 out]
              }
              frame #1 {
                n1599 = Wait (ms)(milliseconds to wait=w2540) -> ()  [unwired: 1 out]
              }
              frame #2 {
                n1600 = VISA Write(VISA resource name=w2545, write buffer=w2546, error in (no error)=w2544) -> (VISA resource name out=w2547:refnum<visa-resource-name>, error out=w2543:errorcluster)  [unwired: 1 out]
              }
              frame #3 {
                n1601 = Wait (ms)(milliseconds to wait=w2548) -> ()  [unwired: 1 out]
              }
              frame #4 {
                n1602 = VISA Write(VISA resource name=w2555, write buffer=w2553, error in (no error)=w2552) -> (VISA resource name out=w2554:refnum<visa-resource-name>, error out=w2551:errorcluster)  [unwired: 1 out]
              }
              frame #5 {
                n1603 = Wait (ms)(milliseconds to wait=w2556) -> ()  [unwired: 1 out]
              }
              frame #6 {
                n1604 = VISA Write(VISA resource name=w2563, write buffer=w2561, error in (no error)=w2560) -> (VISA resource name out=w2562:refnum<visa-resource-name>, error out=w2559:errorcluster)  [unwired: 1 out]
              }
              frame #7 {
                n1605 = Wait (ms)(milliseconds to wait=w2564) -> ()  [unwired: 1 out]
              }
              frame #8 {
                n1606 = Concatenate Strings("start ", "\r") -> (w2571:string)
                n1607 = VISA Write(VISA resource name=w2573, write buffer=w2571, error in (no error)=w2572) -> (VISA resource name out=w2568:refnum<visa-resource-name>, error out=w2567:errorcluster)  [unwired: 1 out]
              }
              frame #9 {
                n1608 = Wait (ms)(milliseconds to wait=w2574) -> ()  [unwired: 1 out]
              }
              frame #10 {
                n1609 = local write "Flush Pump 2"(FALSE ("Flush Pump 1")) -> ()
                n1610 = Concatenate Strings("enter main ", "\r") -> (w2581:string)
                n1611 = VISA Write(VISA resource name=w2580, write buffer=w2581, error in (no error)=w2579) -> (VISA resource name out=w2578:refnum<visa-resource-name>, error out=w2577:errorcluster)  [unwired: 1 out]
                n1612 = VISA Close(VISA resource name=w2578, error in (no error)=w2577) -> ()  [unwired: 1 out]
              }
            }
            n1613 = Concatenate Strings("set units 4 ", w2501) -> (w2514:string)
            n1614 = Multiply(x="Flush \nRate (ul/min)  2", y=60) -> (x*y=w2512:dbl)
            n1615 = Number To Decimal String(number=w2512) -> (decimal integer string=w2515:string)  [unwired: 1 in]
            n1616 = Concatenate Strings("set rate ", w2515, w2501) -> (w2517:string)
            n1617 = Number To Decimal String(number="Flush\nVolume (ul)  2") -> (decimal integer string=w2519:string)  [unwired: 1 in]
            n1618 = Concatenate Strings("set volume ", w2519, w2501) -> (w2520:string)
          }
          event "Stop": Value Change {
            n1619 = event-data() -> ()  [unwired: 1 in, 5 out]
            n1620 = local read "Stop"() -> (w2585:bool)
          }
          event "Inject Pump 2": Value Change {
            n1621 = event-data() -> ()  [unwired: 1 in, 5 out]
            n1622 = case shown="True" "Inject Pump 2" {
              tunnel: w2586 -> [w2589 w2631]
              frame False {
                n1623 = local read "Write Wait"() -> (w2588:i32)
                n1624 = call-poly "VISA Configure Serial Port"("VISA resource name"=w2589) -> ("VISA resource name out"=w2593:refnum<visa-resource-name>, "error out"=w2594:errorcluster)  [unwired: 13 in]
                n1625 = Concatenate Strings("enter pump2", "\r") -> (w2591:string)
                n1626 = flat-sequence {
                  tunnel: w2594 -> [w2605]
                  tunnel: w2593 -> [w2607]
                  tunnel: [w2606] -> w2602
                  tunnel: [w2604] -> w2601
                  tunnel: w2591 -> [w2603]
                  tunnel: w2602 -> [w2610]
                  tunnel: w2601 -> [w2609]
                  tunnel: [w2610] -> w2600
                  tunnel: [w2609] -> w2599
                  tunnel: w2588 -> [w2608]
                  tunnel: [w2614] -> w2598
                  tunnel: [w2613] -> w2597
                  tunnel: w2600 -> [w2612]
                  tunnel: w2599 -> [w2611]
                  tunnel: w2598 -> [w2620]
                  tunnel: [w2620] -> w2596
                  tunnel: w2597 -> [w2619]
                  tunnel: [w2619] -> w2595
                  tunnel: w2588 -> [w2618]
                  tunnel: w2596 -> [w2624]
                  tunnel: w2595 -> [w2623]
                  frame #0 {
                    n1627 = VISA Write(VISA resource name=w2607, write buffer=w2603, error in (no error)=w2605) -> (VISA resource name out=w2606:refnum<visa-resource-name>, error out=w2604:errorcluster)  [unwired: 1 out]
                  }
                  frame #1 {
                    n1628 = Wait (ms)(milliseconds to wait=w2608) -> ()  [unwired: 1 out]
                  }
                  frame #2 {
                    n1629 = Concatenate Strings("stop ", "\r") -> (w2617:string)
                    n1630 = VISA Write(VISA resource name=w2612, write buffer=w2617, error in (no error)=w2611) -> (VISA resource name out=w2614:refnum<visa-resource-name>, error out=w2613:errorcluster)  [unwired: 1 out]
                  }
                  frame #3 {
                    n1631 = Wait (ms)(milliseconds to wait=w2618) -> ()  [unwired: 1 out]
                  }
                  frame #4 {
                    n1632 = Concatenate Strings("enter main ", "\r") -> (w2625:string)
                    n1633 = VISA Write(VISA resource name=w2624, write buffer=w2625, error in (no error)=w2623) -> (VISA resource name out=w2622:refnum<visa-resource-name>, error out=w2621:errorcluster)  [unwired: 1 out]
                    n1634 = VISA Close(VISA resource name=w2622, error in (no error)=w2621) -> ()  [unwired: 1 out]
                  }
                }
              }
              frame True {
                w2644 = "\r"
                n1635 = call-poly "VISA Configure Serial Port"("VISA resource name"=w2631) -> ("VISA resource name out"=w2633:refnum<visa-resource-name>, "error out"=w2632:errorcluster)  [unwired: 13 in]
                n1636 = local read "Write Wait"() -> (w2628:i32)
                n1637 = Concatenate Strings("enter pump2", w2644) -> (w2643:string)
                n1638 = flat-sequence {
                  tunnel: w2632 -> [w2667]
                  tunnel: w2633 -> [w2669]
                  tunnel: [w2668] -> w2664
                  tunnel: [w2666] -> w2663
                  tunnel: w2643 -> [w2665]
                  tunnel: w2664 -> [w2672]
                  tunnel: [w2672] -> w2662
                  tunnel: w2663 -> [w2671]
                  tunnel: [w2671] -> w2661
                  tunnel: w2628 -> [w2670]
                  tunnel: [w2677] -> w2660
                  tunnel: w2640 -> [w2676]
                  tunnel: [w2673] -> w2659
                  tunnel: w2662 -> [w2675]
                  tunnel: w2661 -> [w2674]
                  tunnel: w2660 -> [w2680]
                  tunnel: [w2680] -> w2658
                  tunnel: [w2679] -> w2657
                  tunnel: w2659 -> [w2679]
                  tunnel: w2628 -> [w2678]
                  tunnel: w2658 -> [w2685]
                  tunnel: [w2684] -> w2656
                  tunnel: w2637 -> [w2683]
                  tunnel: w2657 -> [w2682]
                  tunnel: [w2681] -> w2655
                  tunnel: w2656 -> [w2688]
                  tunnel: [w2688] -> w2654
                  tunnel: [w2687] -> w2653
                  tunnel: w2655 -> [w2687]
                  tunnel: w2628 -> [w2686]
                  tunnel: w2654 -> [w2693]
                  tunnel: [w2692] -> w2652
                  tunnel: w2634 -> [w2691]
                  tunnel: w2653 -> [w2690]
                  tunnel: [w2689] -> w2651
                  tunnel: [w2696] -> w2650
                  tunnel: w2652 -> [w2696]
                  tunnel: [w2695] -> w2649
                  tunnel: w2651 -> [w2695]
                  tunnel: w2628 -> [w2694]
                  tunnel: w2650 -> [w2703]
                  tunnel: w2649 -> [w2702]
                  tunnel: [w2698] -> w2648
                  tunnel: [w2697] -> w2647
                  tunnel: w2648 -> [w2706]
                  tunnel: [w2706] -> w2646
                  tunnel: w2647 -> [w2705]
                  tunnel: [w2705] -> w2645
                  tunnel: w2628 -> [w2704]
                  tunnel: w2646 -> [w2710]
                  tunnel: w2645 -> [w2709]
                  frame #0 {
                    n1639 = VISA Write(VISA resource name=w2669, write buffer=w2665, error in (no error)=w2667) -> (VISA resource name out=w2668:refnum<visa-resource-name>, error out=w2666:errorcluster)  [unwired: 1 out]
                  }
                  frame #1 {
                    n1640 = Wait (ms)(milliseconds to wait=w2670) -> ()  [unwired: 1 out]
                  }
                  frame #2 {
                    n1641 = VISA Write(VISA resource name=w2675, write buffer=w2676, error in (no error)=w2674) -> (VISA resource name out=w2677:refnum<visa-resource-name>, error out=w2673:errorcluster)  [unwired: 1 out]
                  }
                  frame #3 {
                    n1642 = Wait (ms)(milliseconds to wait=w2678) -> ()  [unwired: 1 out]
                  }
                  frame #4 {
                    n1643 = VISA Write(VISA resource name=w2685, write buffer=w2683, error in (no error)=w2682) -> (VISA resource name out=w2684:refnum<visa-resource-name>, error out=w2681:errorcluster)  [unwired: 1 out]
                  }
                  frame #5 {
                    n1644 = Wait (ms)(milliseconds to wait=w2686) -> ()  [unwired: 1 out]
                  }
                  frame #6 {
                    n1645 = VISA Write(VISA resource name=w2693, write buffer=w2691, error in (no error)=w2690) -> (VISA resource name out=w2692:refnum<visa-resource-name>, error out=w2689:errorcluster)  [unwired: 1 out]
                  }
                  frame #7 {
                    n1646 = Wait (ms)(milliseconds to wait=w2694) -> ()  [unwired: 1 out]
                  }
                  frame #8 {
                    n1647 = Concatenate Strings("start ", "\r") -> (w2701:string)
                    n1648 = VISA Write(VISA resource name=w2703, write buffer=w2701, error in (no error)=w2702) -> (VISA resource name out=w2698:refnum<visa-resource-name>, error out=w2697:errorcluster)  [unwired: 1 out]
                  }
                  frame #9 {
                    n1649 = Wait (ms)(milliseconds to wait=w2704) -> ()  [unwired: 1 out]
                  }
                  frame #10 {
                    n1650 = Concatenate Strings("enter main ", "\r") -> (w2711:string)
                    n1651 = VISA Write(VISA resource name=w2710, write buffer=w2711, error in (no error)=w2709) -> (VISA resource name out=w2708:refnum<visa-resource-name>, error out=w2707:errorcluster)  [unwired: 1 out]
                    n1652 = VISA Close(VISA resource name=w2708, error in (no error)=w2707) -> ()  [unwired: 1 out]
                  }
                }
                n1653 = local read "Normal \nRate (ul/hr)  2"() -> (w2629:dbl)
                n1654 = Concatenate Strings("set units 4 ", w2644) -> (w2640:string)
                n1655 = local read "Normal \nVolume (ul) 2"() -> (w2630:dbl)
                n1656 = Number To Decimal String(number=w2629) -> (decimal integer string=w2639:string)  [unwired: 1 in]
                n1657 = Concatenate Strings("set rate ", w2639, w2644) -> (w2637:string)
                n1658 = Number To Decimal String(number=w2630) -> (decimal integer string=w2635:string)  [unwired: 1 in]
                n1659 = Concatenate Strings("set volume ", w2635, w2644) -> (w2634:string)
              }
            }
          }
          event "Inject Pump 1": Value Change {
            n1660 = event-data() -> ()  [unwired: 1 in, 5 out]
            n1661 = case shown="True" "Inject Pump 1" {
              tunnel: w2714 -> [w2717 w2759]
              frame False {
                n1662 = local read "Write Wait"() -> (w2716:i32)
                n1663 = call-poly "VISA Configure Serial Port"("VISA resource name"=w2717) -> ("VISA resource name out"=w2721:refnum<visa-resource-name>, "error out"=w2722:errorcluster)  [unwired: 13 in]
                n1664 = Concatenate Strings("enter pump1", "\r") -> (w2719:string)
                n1665 = flat-sequence {
                  tunnel: w2722 -> [w2733]
                  tunnel: w2721 -> [w2735]
                  tunnel: [w2734] -> w2730
                  tunnel: [w2732] -> w2729
                  tunnel: w2719 -> [w2731]
                  tunnel: w2730 -> [w2738]
                  tunnel: w2729 -> [w2737]
                  tunnel: [w2738] -> w2728
                  tunnel: [w2737] -> w2727
                  tunnel: w2716 -> [w2736]
                  tunnel: [w2742] -> w2726
                  tunnel: [w2741] -> w2725
                  tunnel: w2728 -> [w2740]
                  tunnel: w2727 -> [w2739]
                  tunnel: w2726 -> [w2748]
                  tunnel: [w2748] -> w2724
                  tunnel: w2725 -> [w2747]
                  tunnel: [w2747] -> w2723
                  tunnel: w2716 -> [w2746]
                  tunnel: w2724 -> [w2752]
                  tunnel: w2723 -> [w2751]
                  frame #0 {
                    n1666 = VISA Write(VISA resource name=w2735, write buffer=w2731, error in (no error)=w2733) -> (VISA resource name out=w2734:refnum<visa-resource-name>, error out=w2732:errorcluster)  [unwired: 1 out]
                  }
                  frame #1 {
                    n1667 = Wait (ms)(milliseconds to wait=w2736) -> ()  [unwired: 1 out]
                  }
                  frame #2 {
                    n1668 = Concatenate Strings("stop ", "\r") -> (w2745:string)
                    n1669 = VISA Write(VISA resource name=w2740, write buffer=w2745, error in (no error)=w2739) -> (VISA resource name out=w2742:refnum<visa-resource-name>, error out=w2741:errorcluster)  [unwired: 1 out]
                  }
                  frame #3 {
                    n1670 = Wait (ms)(milliseconds to wait=w2746) -> ()  [unwired: 1 out]
                  }
                  frame #4 {
                    n1671 = Concatenate Strings("enter main ", "\r") -> (w2753:string)
                    n1672 = VISA Write(VISA resource name=w2752, write buffer=w2753, error in (no error)=w2751) -> (VISA resource name out=w2750:refnum<visa-resource-name>, error out=w2749:errorcluster)  [unwired: 1 out]
                    n1673 = VISA Close(VISA resource name=w2750, error in (no error)=w2749) -> ()  [unwired: 1 out]
                  }
                }
              }
              frame True {
                w2772 = "\r"
                n1674 = call-poly "VISA Configure Serial Port"("VISA resource name"=w2759) -> ("VISA resource name out"=w2761:refnum<visa-resource-name>, "error out"=w2760:errorcluster)  [unwired: 13 in]
                n1675 = local read "Write Wait"() -> (w2756:i32)
                n1676 = flat-sequence {
                  tunnel: w2760 -> [w2795]
                  tunnel: w2761 -> [w2797]
                  tunnel: [w2796] -> w2792
                  tunnel: [w2794] -> w2791
                  tunnel: w2771 -> [w2793]
                  tunnel: w2792 -> [w2800]
                  tunnel: [w2800] -> w2790
                  tunnel: w2791 -> [w2799]
                  tunnel: [w2799] -> w2789
                  tunnel: w2756 -> [w2798]
                  tunnel: [w2805] -> w2788
                  tunnel: w2768 -> [w2804]
                  tunnel: [w2801] -> w2787
                  tunnel: w2790 -> [w2803]
                  tunnel: w2789 -> [w2802]
                  tunnel: w2788 -> [w2808]
                  tunnel: [w2808] -> w2786
                  tunnel: [w2807] -> w2785
                  tunnel: w2787 -> [w2807]
                  tunnel: w2756 -> [w2806]
                  tunnel: w2786 -> [w2813]
                  tunnel: [w2812] -> w2784
                  tunnel: w2765 -> [w2811]
                  tunnel: w2785 -> [w2810]
                  tunnel: [w2809] -> w2783
                  tunnel: w2784 -> [w2816]
                  tunnel: [w2816] -> w2782
                  tunnel: [w2815] -> w2781
                  tunnel: w2783 -> [w2815]
                  tunnel: w2756 -> [w2814]
                  tunnel: w2782 -> [w2821]
                  tunnel: [w2820] -> w2780
                  tunnel: w2762 -> [w2819]
                  tunnel: w2781 -> [w2818]
                  tunnel: [w2817] -> w2779
                  tunnel: [w2824] -> w2778
                  tunnel: w2780 -> [w2824]
                  tunnel: [w2823] -> w2777
                  tunnel: w2779 -> [w2823]
                  tunnel: w2756 -> [w2822]
                  tunnel: w2778 -> [w2831]
                  tunnel: w2777 -> [w2830]
                  tunnel: [w2826] -> w2776
                  tunnel: [w2825] -> w2775
                  tunnel: w2776 -> [w2834]
                  tunnel: [w2834] -> w2774
                  tunnel: w2775 -> [w2833]
                  tunnel: [w2833] -> w2773
                  tunnel: w2756 -> [w2832]
                  tunnel: w2774 -> [w2838]
                  tunnel: w2773 -> [w2837]
                  frame #0 {
                    n1677 = VISA Write(VISA resource name=w2797, write buffer=w2793, error in (no error)=w2795) -> (VISA resource name out=w2796:refnum<visa-resource-name>, error out=w2794:errorcluster)  [unwired: 1 out]
                  }
                  frame #1 {
                    n1678 = Wait (ms)(milliseconds to wait=w2798) -> ()  [unwired: 1 out]
                  }
                  frame #2 {
                    n1679 = VISA Write(VISA resource name=w2803, write buffer=w2804, error in (no error)=w2802) -> (VISA resource name out=w2805:refnum<visa-resource-name>, error out=w2801:errorcluster)  [unwired: 1 out]
                  }
                  frame #3 {
                    n1680 = Wait (ms)(milliseconds to wait=w2806) -> ()  [unwired: 1 out]
                  }
                  frame #4 {
                    n1681 = VISA Write(VISA resource name=w2813, write buffer=w2811, error in (no error)=w2810) -> (VISA resource name out=w2812:refnum<visa-resource-name>, error out=w2809:errorcluster)  [unwired: 1 out]
                  }
                  frame #5 {
                    n1682 = Wait (ms)(milliseconds to wait=w2814) -> ()  [unwired: 1 out]
                  }
                  frame #6 {
                    n1683 = VISA Write(VISA resource name=w2821, write buffer=w2819, error in (no error)=w2818) -> (VISA resource name out=w2820:refnum<visa-resource-name>, error out=w2817:errorcluster)  [unwired: 1 out]
                  }
                  frame #7 {
                    n1684 = Wait (ms)(milliseconds to wait=w2822) -> ()  [unwired: 1 out]
                  }
                  frame #8 {
                    n1685 = Concatenate Strings("start ", "\r") -> (w2829:string)
                    n1686 = VISA Write(VISA resource name=w2831, write buffer=w2829, error in (no error)=w2830) -> (VISA resource name out=w2826:refnum<visa-resource-name>, error out=w2825:errorcluster)  [unwired: 1 out]
                  }
                  frame #9 {
                    n1687 = Wait (ms)(milliseconds to wait=w2832) -> ()  [unwired: 1 out]
                  }
                  frame #10 {
                    n1688 = Concatenate Strings("enter main ", "\r") -> (w2839:string)
                    n1689 = VISA Write(VISA resource name=w2838, write buffer=w2839, error in (no error)=w2837) -> (VISA resource name out=w2836:refnum<visa-resource-name>, error out=w2835:errorcluster)  [unwired: 1 out]
                    n1690 = VISA Close(VISA resource name=w2836, error in (no error)=w2835) -> ()  [unwired: 1 out]
                  }
                }
                n1691 = Concatenate Strings("enter pump1", w2772) -> (w2771:string)
                n1692 = local read "Normal \nRate (ul/hr)"() -> (w2757:dbl)
                n1693 = Concatenate Strings("set units 4 ", w2772) -> (w2768:string)
                n1694 = local read "Normal \nVolume (ul)"() -> (w2758:dbl)
                n1695 = Number To Decimal String(number=w2757) -> (decimal integer string=w2767:string)  [unwired: 1 in]
                n1696 = Concatenate Strings("set rate ", w2767, w2772) -> (w2765:string)
                n1697 = Number To Decimal String(number=w2758) -> (decimal integer string=w2763:string)  [unwired: 1 in]
                n1698 = Concatenate Strings("set volume ", w2763, w2772) -> (w2762:string)
              }
            }
          }
          event "Normal \nVolume (ul)": Value Change {
            n1699 = event-data() -> ()  [unwired: 1 in, 5 out]
            n1700 = call-poly "VISA Configure Serial Port"("VISA resource name"=w2857) -> ("VISA resource name out"=w2859:refnum<visa-resource-name>, "error out"=w2858:errorcluster)  [unwired: 13 in]
            n1701 = local read "Write Wait"() -> (w2842:i32)
            n1702 = Concatenate Strings("enter pump1", "\r") -> (w2861:string)
            n1703 = flat-sequence {
              tunnel: w2858 -> [w2871]
              tunnel: w2859 -> [w2873]
              tunnel: [w2872] -> w2851
              tunnel: [w2870] -> w2850
              tunnel: w2861 -> [w2869]
              tunnel: w2851 -> [w2876]
              tunnel: [w2876] -> w2849
              tunnel: w2850 -> [w2875]
              tunnel: [w2875] -> w2847
              tunnel: w2842 -> [w2874]
              tunnel: w2849 -> [w2880]
              tunnel: [w2881] -> w2848
              tunnel: w2847 -> [w2879]
              tunnel: [w2878] -> w2846
              tunnel: w2843 -> [w2877]
              tunnel: w2848 -> [w2884]
              tunnel: w2846 -> [w2883]
              tunnel: [w2884] -> w2868
              tunnel: [w2883] -> w2867
              tunnel: w2842 -> [w2882]
              tunnel: [w2889] -> w2866
              tunnel: [w2888] -> w2865
              tunnel: w2868 -> [w2887]
              tunnel: w2867 -> [w2886]
              tunnel: w2852 -> [w2885]
              tunnel: w2866 -> [w2892]
              tunnel: [w2892] -> w2864
              tunnel: w2865 -> [w2891]
              tunnel: [w2891] -> w2863
              tunnel: w2842 -> [w2890]
              tunnel: w2864 -> [w2896]
              tunnel: w2863 -> [w2895]
              frame #0 {
                n1704 = VISA Write(VISA resource name=w2873, write buffer=w2869, error in (no error)=w2871) -> (VISA resource name out=w2872:refnum<visa-resource-name>, error out=w2870:errorcluster)  [unwired: 1 out]
              }
              frame #1 {
                n1705 = Wait (ms)(milliseconds to wait=w2874) -> ()  [unwired: 1 out]
              }
              frame #2 {
                n1706 = VISA Write(VISA resource name=w2880, write buffer=w2877, error in (no error)=w2879) -> (VISA resource name out=w2881:refnum<visa-resource-name>, error out=w2878:errorcluster)  [unwired: 1 out]
              }
              frame #3 {
                n1707 = Wait (ms)(milliseconds to wait=w2882) -> ()  [unwired: 1 out]
              }
              frame #4 {
                n1708 = VISA Write(VISA resource name=w2887, write buffer=w2885, error in (no error)=w2886) -> (VISA resource name out=w2889:refnum<visa-resource-name>, error out=w2888:errorcluster)  [unwired: 1 out]
              }
              frame #5 {
                n1709 = Wait (ms)(milliseconds to wait=w2890) -> ()  [unwired: 1 out]
              }
              frame #6 {
                n1710 = Concatenate Strings("enter main ", "\r") -> (w2897:string)
                n1711 = VISA Write(VISA resource name=w2896, write buffer=w2897, error in (no error)=w2895) -> (VISA resource name out=w2894:refnum<visa-resource-name>, error out=w2893:errorcluster)  [unwired: 1 out]
                n1712 = VISA Close(VISA resource name=w2894, error in (no error)=w2893) -> ()  [unwired: 1 out]
              }
            }
            n1713 = Concatenate Strings("set units 4", "\r") -> (w2843:string)
            n1714 = Number To Decimal String(number="Normal \nVolume (ul)") -> (decimal integer string=w2854:string)  [unwired: 1 in]
            n1715 = Concatenate Strings("set volume", w2854, "\r") -> (w2852:string)
          }
          event "Normal \nRate (ul/hr)": Value Change {
            n1716 = event-data() -> ()  [unwired: 1 in, 5 out]
            n1717 = call-poly "VISA Configure Serial Port"("VISA resource name"=w2902) -> ("VISA resource name out"=w2910:refnum<visa-resource-name>, "error out"=w2909:errorcluster)  [unwired: 13 in]
            n1718 = local read "Write Wait"() -> (w2900:i32)
            n1719 = Concatenate Strings("enter pump1", "\r") -> (w2912:string)
            n1720 = flat-sequence {
              tunnel: w2909 -> [w2929]
              tunnel: w2910 -> [w2931]
              tunnel: [w2930] -> w2925
              tunnel: [w2928] -> w2924
              tunnel: w2912 -> [w2927]
              tunnel: w2925 -> [w2934]
              tunnel: [w2934] -> w2923
              tunnel: w2924 -> [w2933]
              tunnel: [w2933] -> w2922
              tunnel: w2900 -> [w2932]
              tunnel: w2923 -> [w2938]
              tunnel: [w2939] -> w2921
              tunnel: w2922 -> [w2937]
              tunnel: [w2936] -> w2920
              tunnel: w2903 -> [w2935]
              tunnel: w2921 -> [w2942]
              tunnel: w2920 -> [w2941]
              tunnel: [w2942] -> w2919
              tunnel: [w2941] -> w2918
              tunnel: w2900 -> [w2940]
              tunnel: [w2947] -> w2917
              tunnel: [w2946] -> w2916
              tunnel: w2919 -> [w2945]
              tunnel: w2918 -> [w2944]
              tunnel: w2906 -> [w2943]
              tunnel: w2917 -> [w2950]
              tunnel: [w2950] -> w2915
              tunnel: w2916 -> [w2949]
              tunnel: [w2949] -> w2914
              tunnel: w2900 -> [w2948]
              tunnel: w2915 -> [w2954]
              tunnel: w2914 -> [w2953]
              frame #0 {
                n1721 = VISA Write(VISA resource name=w2931, write buffer=w2927, error in (no error)=w2929) -> (VISA resource name out=w2930:refnum<visa-resource-name>, error out=w2928:errorcluster)  [unwired: 1 out]
              }
              frame #1 {
                n1722 = Wait (ms)(milliseconds to wait=w2932) -> ()  [unwired: 1 out]
              }
              frame #2 {
                n1723 = VISA Write(VISA resource name=w2938, write buffer=w2935, error in (no error)=w2937) -> (VISA resource name out=w2939:refnum<visa-resource-name>, error out=w2936:errorcluster)  [unwired: 1 out]
              }
              frame #3 {
                n1724 = Wait (ms)(milliseconds to wait=w2940) -> ()  [unwired: 1 out]
              }
              frame #4 {
                n1725 = VISA Write(VISA resource name=w2945, write buffer=w2943, error in (no error)=w2944) -> (VISA resource name out=w2947:refnum<visa-resource-name>, error out=w2946:errorcluster)  [unwired: 1 out]
              }
              frame #5 {
                n1726 = Wait (ms)(milliseconds to wait=w2948) -> ()  [unwired: 1 out]
              }
              frame #6 {
                n1727 = Concatenate Strings("enter main ", "\r") -> (w2955:string)
                n1728 = VISA Write(VISA resource name=w2954, write buffer=w2955, error in (no error)=w2953) -> (VISA resource name out=w2952:refnum<visa-resource-name>, error out=w2951:errorcluster)  [unwired: 1 out]
                n1729 = VISA Close(VISA resource name=w2952, error in (no error)=w2951) -> ()  [unwired: 1 out]
              }
            }
            n1730 = Concatenate Strings("set units 4", "\r") -> (w2903:string)
            n1731 = Number To Decimal String(number="Normal \nRate (ul/hr)") -> (decimal integer string=w2901:string)  [unwired: 1 in]
            n1732 = Concatenate Strings("set rate", w2901, "\r") -> (w2906:string)
          }
          event "Normal \nRate (ul/hr)  2": Value Change {
            n1733 = event-data() -> ()  [unwired: 1 in, 5 out]
            n1734 = call-poly "VISA Configure Serial Port"("VISA resource name"=w2960) -> ("VISA resource name out"=w2968:refnum<visa-resource-name>, "error out"=w2967:errorcluster)  [unwired: 13 in]
            n1735 = local read "Write Wait"() -> (w2958:i32)
            n1736 = Concatenate Strings("enter pump2", "\r") -> (w2970:string)
            n1737 = flat-sequence {
              tunnel: w2967 -> [w2987]
              tunnel: w2968 -> [w2989]
              tunnel: [w2988] -> w2983
              tunnel: [w2986] -> w2982
              tunnel: w2970 -> [w2985]
              tunnel: w2983 -> [w2992]
              tunnel: [w2992] -> w2981
              tunnel: w2982 -> [w2991]
              tunnel: [w2991] -> w2980
              tunnel: w2958 -> [w2990]
              tunnel: w2981 -> [w2996]
              tunnel: [w2997] -> w2979
              tunnel: w2980 -> [w2995]
              tunnel: [w2994] -> w2978
              tunnel: w2961 -> [w2993]
              tunnel: w2979 -> [w3000]
              tunnel: w2978 -> [w2999]
              tunnel: [w3000] -> w2977
              tunnel: [w2999] -> w2976
              tunnel: w2958 -> [w2998]
              tunnel: [w3005] -> w2975
              tunnel: [w3004] -> w2974
              tunnel: w2977 -> [w3003]
              tunnel: w2976 -> [w3002]
              tunnel: w2964 -> [w3001]
              tunnel: w2975 -> [w3008]
              tunnel: [w3008] -> w2973
              tunnel: w2974 -> [w3007]
              tunnel: [w3007] -> w2972
              tunnel: w2958 -> [w3006]
              tunnel: w2973 -> [w3012]
              tunnel: w2972 -> [w3011]
              frame #0 {
                n1738 = VISA Write(VISA resource name=w2989, write buffer=w2985, error in (no error)=w2987) -> (VISA resource name out=w2988:refnum<visa-resource-name>, error out=w2986:errorcluster)  [unwired: 1 out]
              }
              frame #1 {
                n1739 = Wait (ms)(milliseconds to wait=w2990) -> ()  [unwired: 1 out]
              }
              frame #2 {
                n1740 = VISA Write(VISA resource name=w2996, write buffer=w2993, error in (no error)=w2995) -> (VISA resource name out=w2997:refnum<visa-resource-name>, error out=w2994:errorcluster)  [unwired: 1 out]
              }
              frame #3 {
                n1741 = Wait (ms)(milliseconds to wait=w2998) -> ()  [unwired: 1 out]
              }
              frame #4 {
                n1742 = VISA Write(VISA resource name=w3003, write buffer=w3001, error in (no error)=w3002) -> (VISA resource name out=w3005:refnum<visa-resource-name>, error out=w3004:errorcluster)  [unwired: 1 out]
              }
              frame #5 {
                n1743 = Wait (ms)(milliseconds to wait=w3006) -> ()  [unwired: 1 out]
              }
              frame #6 {
                n1744 = Concatenate Strings("enter main ", "\r") -> (w3013:string)
                n1745 = VISA Write(VISA resource name=w3012, write buffer=w3013, error in (no error)=w3011) -> (VISA resource name out=w3010:refnum<visa-resource-name>, error out=w3009:errorcluster)  [unwired: 1 out]
                n1746 = VISA Close(VISA resource name=w3010, error in (no error)=w3009) -> ()  [unwired: 1 out]
              }
            }
            n1747 = Concatenate Strings("set units 4", "\r") -> (w2961:string)
            n1748 = Number To Decimal String(number="Normal \nRate (ul/hr)  2") -> (decimal integer string=w2959:string)  [unwired: 1 in]
            n1749 = Concatenate Strings("set rate", w2959, "\r") -> (w2964:string)
          }
          event "Normal \nVolume (ul) 2": Value Change {
            n1750 = event-data() -> ()  [unwired: 1 in, 5 out]
            n1751 = call-poly "VISA Configure Serial Port"("VISA resource name"=w3019) -> ("VISA resource name out"=w3023:refnum<visa-resource-name>, "error out"=w3024:errorcluster)  [unwired: 13 in]
            n1752 = local read "Write Wait"() -> (w3016:i32)
            n1753 = Concatenate Strings("enter pump2", "\r") -> (w3021:string)
            n1754 = flat-sequence {
              tunnel: w3024 -> [w3045]
              tunnel: w3023 -> [w3047]
              tunnel: [w3046] -> w3042
              tunnel: [w3044] -> w3041
              tunnel: w3021 -> [w3043]
              tunnel: w3042 -> [w3050]
              tunnel: [w3050] -> w3040
              tunnel: w3041 -> [w3049]
              tunnel: [w3049] -> w3039
              tunnel: w3016 -> [w3048]
              tunnel: w3040 -> [w3054]
              tunnel: [w3055] -> w3038
              tunnel: w3039 -> [w3053]
              tunnel: [w3052] -> w3037
              tunnel: w3030 -> [w3051]
              tunnel: w3038 -> [w3058]
              tunnel: w3037 -> [w3057]
              tunnel: [w3058] -> w3036
              tunnel: [w3057] -> w3035
              tunnel: w3016 -> [w3056]
              tunnel: [w3063] -> w3034
              tunnel: [w3062] -> w3033
              tunnel: w3036 -> [w3061]
              tunnel: w3035 -> [w3060]
              tunnel: w3027 -> [w3059]
              tunnel: w3034 -> [w3066]
              tunnel: [w3066] -> w3032
              tunnel: w3033 -> [w3065]
              tunnel: [w3065] -> w3031
              tunnel: w3016 -> [w3064]
              tunnel: w3032 -> [w3070]
              tunnel: w3031 -> [w3069]
              frame #0 {
                n1755 = VISA Write(VISA resource name=w3047, write buffer=w3043, error in (no error)=w3045) -> (VISA resource name out=w3046:refnum<visa-resource-name>, error out=w3044:errorcluster)  [unwired: 1 out]
              }
              frame #1 {
                n1756 = Wait (ms)(milliseconds to wait=w3048) -> ()  [unwired: 1 out]
              }
              frame #2 {
                n1757 = VISA Write(VISA resource name=w3054, write buffer=w3051, error in (no error)=w3053) -> (VISA resource name out=w3055:refnum<visa-resource-name>, error out=w3052:errorcluster)  [unwired: 1 out]
              }
              frame #3 {
                n1758 = Wait (ms)(milliseconds to wait=w3056) -> ()  [unwired: 1 out]
              }
              frame #4 {
                n1759 = VISA Write(VISA resource name=w3061, write buffer=w3059, error in (no error)=w3060) -> (VISA resource name out=w3063:refnum<visa-resource-name>, error out=w3062:errorcluster)  [unwired: 1 out]
              }
              frame #5 {
                n1760 = Wait (ms)(milliseconds to wait=w3064) -> ()  [unwired: 1 out]
              }
              frame #6 {
                n1761 = Concatenate Strings("enter main ", "\r") -> (w3071:string)
                n1762 = VISA Write(VISA resource name=w3070, write buffer=w3071, error in (no error)=w3069) -> (VISA resource name out=w3068:refnum<visa-resource-name>, error out=w3067:errorcluster)  [unwired: 1 out]
                n1763 = VISA Close(VISA resource name=w3068, error in (no error)=w3067) -> ()  [unwired: 1 out]
              }
            }
            n1764 = Concatenate Strings("set units 4", "\r") -> (w3030:string)
            n1765 = Number To Decimal String(number="Normal \nVolume (ul) 2") -> (decimal integer string=w3017:string)  [unwired: 1 in]
            n1766 = Concatenate Strings("set volume", w3017, "\r") -> (w3027:string)
          }
        }
        n1767 = node-c288() -> ()  [unwired: 1 in, 1 out]
      }
      n1768 = node-c288(w2403) -> ()  [unwired: 1 out]
    }
    frame Enabled {
      n1769 = node-c288(2 ("Processor")) -> (w3083:T14)  [unwired: 3 in]
      n1770 = timed-loop "Pump Control" {
        timing: w3083 -> [_]
        timing-out: [_] -> w3082
        tunnel: refnum<visa-resource-name> "COM4" ("VISA resource name") -> [w3085]
        stop <- w3084 stop-if-true
        n1771 = node-c288() -> ()  [unwired: 1 in, 1 out]
        n1772 = event shown="[2] \"Inject Sample\": Value Change" {
          selector: _ -> [_ _ _ _ _]
          dyn-events: _ -> [_ _ _ _ _]
          timeout: _ -> [_ _ _ _ _]
          tunnel: w3085 -> [w3091 _ w3165 w3198 w3203]
          tunnel: [_ w3163 _ _ _] -> w3084
          event "Flush Sample": Value Change {
            n1773 = event-data() -> ()  [unwired: 1 in, 5 out]
            n1774 = local read "Write Wait"() -> (w3105:i32)
            n1775 = flat-sequence {
              tunnel: [w3129] -> w3125
              tunnel: [w3128] -> w3124
              tunnel: "CLD" -> [w3127]
              tunnel: w3091 -> [w3126]
              tunnel: w3125 -> [w3132]
              tunnel: [w3132] -> w3123
              tunnel: w3124 -> [w3131]
              tunnel: [w3131] -> w3122
              tunnel: w3105 -> [w3130]
              tunnel: [w3137] -> w3121
              tunnel: [w3134] -> w3120
              tunnel: w3123 -> [w3136]
              tunnel: w3122 -> [w3135]
              tunnel: "MODVOL" -> [w3133]
              tunnel: w3121 -> [w3140]
              tunnel: [w3140] -> w3119
              tunnel: [w3139] -> w3118
              tunnel: w3120 -> [w3139]
              tunnel: w3105 -> [w3138]
              tunnel: w3119 -> [w3145]
              tunnel: [w3144] -> w3117
              tunnel: w3107 -> [w3143]
              tunnel: w3118 -> [w3142]
              tunnel: [w3141] -> w3116
              tunnel: w3117 -> [w3148]
              tunnel: [w3148] -> w3115
              tunnel: [w3147] -> w3114
              tunnel: w3116 -> [w3147]
              tunnel: w3105 -> [w3146]
              tunnel: w3115 -> [w3153]
              tunnel: [w3152] -> w3113
              tunnel: w3109 -> [w3151]
              tunnel: w3114 -> [w3150]
              tunnel: [w3149] -> w3112
              tunnel: [w3156] -> w3110
              tunnel: w3113 -> [w3156]
              tunnel: [w3155] -> w3111
              tunnel: w3112 -> [w3155]
              tunnel: w3105 -> [w3154]
              tunnel: w3111 -> [w3161]
              tunnel: w3110 -> [w3162]
              tunnel: [w3160] -> w3100
              tunnel: "RUN " -> [w3159]
              frame #0 {
                n1776 = call "Write to pump 2.vi"("String to write"=w3127, "VISA resource name"=w3126) -> ("error out"=w3128:errorcluster, "VISA resource name out"=w3129:refnum<visa-resource-name>)  [unwired: 8 in]
              }
              frame #1 {
                n1777 = Wait (ms)(milliseconds to wait=w3130) -> ()  [unwired: 1 out]
              }
              frame #2 {
                n1778 = call "Write to pump 2.vi"("error in (no error)"=w3135, "String to write"=w3133, "VISA resource name"=w3136) -> ("error out"=w3134:errorcluster, "VISA resource name out"=w3137:refnum<visa-resource-name>)  [unwired: 7 in]
              }
              frame #3 {
                n1779 = Wait (ms)(milliseconds to wait=w3138) -> ()  [unwired: 1 out]
              }
              frame #4 {
                n1780 = call "Write to pump 2.vi"("error in (no error)"=w3142, "String to write"=w3143, "VISA resource name"=w3145) -> ("error out"=w3141:errorcluster, "VISA resource name out"=w3144:refnum<visa-resource-name>)  [unwired: 7 in]
              }
              frame #5 {
                n1781 = Wait (ms)(milliseconds to wait=w3146) -> ()  [unwired: 1 out]
              }
              frame #6 {
                n1782 = call "Write to pump 2.vi"("error in (no error)"=w3150, "String to write"=w3151, "VISA resource name"=w3153) -> ("error out"=w3149:errorcluster, "VISA resource name out"=w3152:refnum<visa-resource-name>)  [unwired: 7 in]
              }
              frame #7 {
                n1783 = Wait (ms)(milliseconds to wait=w3154) -> ()  [unwired: 1 out]
              }
              frame #8 {
                w3158 = TRUE ("Inject Pump 3")
                n1784 = Tick Count (ms)() -> (millisecond timer value=→"Flush Sample Start Time":u32)
                n1785 = call "Write to pump 2.vi"("error in (no error)"=w3161, "String to write"=w3159, "VISA resource name"=w3162) -> ("error out"=w3160:errorcluster)  [unwired: 7 in, 1 out]
                n1786 = local write "Inject Sample"(w3158) -> ()
                "Flushing Sample" <- w3158
              }
            }
            n1787 = Number To Fractional String(number="Flush \nRate (ul/min)  3") -> (F-format string=w3093:string)  [unwired: 3 in]
            n1788 = String Subset(string=w3093, length (rest)=6 ("length (rest)")) -> (substring=w3092:string)  [unwired: 1 in]
            n1789 = Concatenate Strings("RAT", w3092, "UM") -> (w3107:string)
            n1790 = Divide(x="Flush\nVolume (ul)  3", y=1000.0) -> (x/y=w3098:dbl)
            n1791 = Number To Fractional String(number=w3098) -> (F-format string=w3097:string)  [unwired: 3 in]
            n1792 = Divide(x="Flush\nVolume (ul)  3", y="Flush \nRate (ul/min)  3") -> (x/y=w3088:dbl)
            n1793 = Multiply(x=w3088, y=60.0) -> (x*y=→"Sample flush time (s)":dbl)
            n1794 = String Subset(string=w3097, length (rest)=6 ("length (rest)")) -> (substring=w3096:string)  [unwired: 1 in]
            n1795 = Concatenate Strings("TGT", w3096) -> (w3109:string)
            "error out" <- w3100
          }
          event "Stop": Value Change {
            n1796 = event-data() -> ()  [unwired: 1 in, 5 out]
            n1797 = local read "Stop"() -> (w3163:bool)
          }
          event "Inject Sample": Value Change {
            n1798 = event-data() -> ()  [unwired: 1 in, 5 out]
            n1799 = case shown="True" "Inject Sample" {
              tunnel: w3165 -> [w3167 w3171]
              frame False {
                n1800 = call "Write to pump 2.vi"("String to write"="STP", "VISA resource name"=w3167) -> ()  [unwired: 8 in, 2 out]
              }
              frame True {
                n1801 = local read "Normal \nRate (ul/hr)  3"() -> (w3172:dbl)
                n1802 = Number To Fractional String(number=w3172) -> (F-format string=w3175:string)  [unwired: 3 in]
                n1803 = String Subset(string=w3175, length (rest)=6 ("length (rest)")) -> (substring=w3173:string)  [unwired: 1 in]
                n1804 = flat-sequence {
                  tunnel: w3171 -> [w3189]
                  tunnel: [w3188] -> w3170
                  tunnel: [w3187] -> w3169
                  tunnel: w3168 -> [w3186]
                  tunnel: "RUN " -> [w3192]
                  tunnel: w3170 -> [w3191]
                  tunnel: w3169 -> [w3190]
                  frame #0 {
                    n1805 = call "Write to pump 2.vi"("String to write"=w3186, "VISA resource name"=w3189) -> ("error out"=w3187:errorcluster, "VISA resource name out"=w3188:refnum<visa-resource-name>)  [unwired: 8 in]
                  }
                  frame #1 {
                    n1806 = call "Write to pump 2.vi"("error in (no error)"=w3190, "String to write"=w3192, "VISA resource name"=w3191) -> ()  [unwired: 7 in, 2 out]
                  }
                }
                n1807 = Concatenate Strings("RAT", w3173, "UH" ("string")) -> ()  [unwired: 1 out]
                n1808 = local read "Normal \nVolume (ul) 3"() -> (w3181:dbl)
                n1809 = Divide(x=w3181, y=1000.0) -> (x/y=w3176:dbl)
                n1810 = Number To Fractional String(number=w3176) -> (F-format string=w3179:string)  [unwired: 3 in]
                n1811 = String Subset(string=w3179, length (rest)=6 ("length (rest)")) -> (substring=w3177:string)  [unwired: 1 in]
                n1812 = Concatenate Strings("TGT", w3177) -> (w3168:string)
              }
            }
          }
          event "Normal \nRate (ul/hr)  3": Value Change {
            n1813 = event-data() -> ()  [unwired: 1 in, 5 out]
            n1814 = Number To Fractional String(number="Normal \nRate (ul/hr)  3") -> (F-format string=w3196:string)  [unwired: 3 in]
            n1815 = String Subset(string=w3196, length (rest)=6 ("length (rest)")) -> (substring=w3194:string)  [unwired: 1 in]
            n1816 = Concatenate Strings("RAT", w3194, "UH") -> (w3197:string)
            n1817 = call "Write to pump 2.vi"("String to write"=w3197, "VISA resource name"=w3198) -> ()  [unwired: 8 in, 2 out]
          }
          event "Clear Volume": Value Change {
            n1818 = event-data() -> ()  [unwired: 1 in, 5 out]
            n1819 = Divide(x="Normal \nVolume (ul) 3", y=1000.0) -> (x/y=w3216:dbl)
            n1820 = Number To Fractional String(number=w3216) -> (F-format string=w3219:string)  [unwired: 3 in]
            n1821 = String Subset(string=w3219, length (rest)=6 ("length (rest)")) -> (substring=w3217:string)  [unwired: 1 in]
            n1822 = flat-sequence {
              tunnel: [w3226] -> w3214
              tunnel: [w3225] -> w3213
              tunnel: w3203 -> [w3224]
              tunnel: w3202 -> [w3223]
              tunnel: [w3228] -> w3211
              tunnel: [w3227] -> w3212
              tunnel: w3208 -> [w3229]
              tunnel: w3214 -> [w3228]
              tunnel: w3213 -> [w3227]
              tunnel: w3212 -> [w3233]
              tunnel: w3211 -> [w3234]
              tunnel: [w3232] -> _
              tunnel: [w3231] -> _
              tunnel: w3201 -> [w3230]
              frame #0 {
                n1823 = call "Write to pump 2.vi"("String to write"=w3223, "VISA resource name"=w3224) -> ("error out"=w3225:errorcluster, "VISA resource name out"=w3226:refnum<visa-resource-name>)  [unwired: 8 in]
              }
              frame #1 {
                n1824 = Wait (ms)(milliseconds to wait=w3229) -> ()  [unwired: 1 out]
              }
              frame #2 {
                n1825 = call "Write to pump 2.vi"("error in (no error)"=w3233, "String to write"=w3230, "VISA resource name"=w3234) -> ("error out"=w3231:errorcluster, "VISA resource name out"=w3232:refnum<visa-resource-name>)  [unwired: 7 in]
              }
            }
            n1826 = local read "Write Wait"() -> (w3208:i32)
            n1827 = Concatenate Strings("TGT", w3217) -> (w3202:string)
            n1828 = local read "Normal \nRate (ul/hr)  3"() -> (w3204:dbl)
            n1829 = local write "Clear Volume"(FALSE ("Clear Volume")) -> ()
            n1830 = Number To Fractional String(number=w3204) -> (F-format string=w3207:string)  [unwired: 3 in]
            n1831 = String Subset(string=w3207, length (rest)=6 ("length (rest)")) -> (substring=w3205:string)  [unwired: 1 in]
            n1832 = Concatenate Strings("RAT", w3205, "UH" ("string")) -> (w3201:string)
          }
        }
        n1833 = node-c288() -> ()  [unwired: 1 in, 1 out]
      }
      n1834 = node-c288(w3082) -> ()  [unwired: 1 out]
    }
  }
  n1835 = node-c288() -> (w90:T14)  [unwired: 4 in]
  n1836 = timed-loop {
    timing: w90 -> [_]
    timing-out: [_] -> w89
    stop <- w3241 stop-if-true
    n1837 = node-c288() -> ()  [unwired: 1 in, 1 out]
    n1838 = event shown="[1] \"Stop\": Value Change" {
      selector: _ -> [_ _]
      dyn-events: _ -> [_ _]
      timeout: _ -> [_ _]
      tunnel: [_ w3242] -> w3241
      event Timeout {
        n1839 = event-data() -> ()  [unwired: 1 in, 2 out]
      }
      event "Stop": Value Change {
        n1840 = event-data() -> ()  [unwired: 1 in, 4 out]
        n1841 = flat-sequence {
          tunnel: ["Stop"] -> w3242
          frame #0 {
            w3243 = FALSE ("Force Feedback")
            n1842 = local write "Force Feedback 1"(w3243) -> ()
            n1843 = local write "Force Feedback 2"(w3243) -> ()
            n1844 = property on="Cancel dwell" class="Bool (strict)"("Val(Sgnl)"=TRUE ("Value (Signaling)")) -> ()  [unwired: 2 in, 2 out]
          }
          frame #1 {
            w3245 = FALSE
            n1845 = local write "Raster scanning..."(w3245) -> ()
            n1846 = local write "Cancel dwell"(w3245) -> ()
            n1847 = local write "Stage moving"(w3245) -> ()
            n1848 = local write "Saving Move"(w3245) -> ()
          }
        }
      }
    }
    n1849 = node-c288() -> ()  [unwired: 1 in, 1 out]
  }
  n1850 = case shown="True" w80 {
    tunnel: w85 -> [_ w3251]
    tunnel: w84 -> [_ w3250]
    tunnel: w83 -> [_ w3249]
    frame False {
    }
    frame True {
      w3253 = T25 3 items=["no dialog", "OK message", "continue or stop message", "OK message + warnings", "continue/stop + warnings"] ("type of dialog (OK msg:1)")
      w3252 = T25 3 items=["no dialog", "OK message", "continue or stop message", "OK message + warnings", "continue/stop + warnings"] ("type of dialog (OK msg:1)")
      n1851 = call <vilib>:"DAQmx Clear Task.vi"("task in"=w3251, "error in"=w3249) -> ("error out"=w3254:errorcluster)  [unwired: 13 in]
      n1852 = call <vilib>:"DAQmx Clear Task.vi"("task in"=w3250) -> ("error out"=w3255:errorcluster)  [unwired: 14 in]
      n1853 = call <vilib>:"Simple Error Handler.vi"("type of dialog (OK msg:1)"=w3253, "error in (no error)"=w3254) -> ()  [unwired: 3 in, 5 out]
      n1854 = call <vilib>:"Simple Error Handler.vi"("type of dialog (OK msg:1)"=w3252, "error in (no error)"=w3255) -> ()  [unwired: 3 in, 5 out]
    }
  }
  n1855 = case shown="\"Raster scan\"" "?" {
    frame "Force Feedback", Default {
    }
    frame "Raster scan" {
    }
  }
  n1856 = node-c288(w89) -> ()  [unwired: 1 out]
  n1857 = node-c288(w92) -> ()  [unwired: 1 out]
  n1858 = local write "Pause Mouse/Mirror Connection"(FALSE ("Pause Mouse/Mirror Connection")) -> ()
  n1859 = local write "Stop"(FALSE ("Stop all")) -> ()
  "CoordinatesMousePressed" <- T6 {"Horizontal"=0, "Vertical"=0} ("Coords when pressed")
  "Deflection" <- T6 {"Horizontal"=0, "Vertical"=0} ("Coords when pressed")
